vi "Main HMI.vi"() -> ()   [LabVIEW 2023]
uses:
  Classes/DCIR_HPPC_class/HPPC Parameters.ctl
  Classes/DCIR_HPPC_class/HPPC Mode.ctl
  Types/Tabs.ctl
  Types/Power Function.ctl
  Types/Setpoints.ctl
  Classes/Battery_class/Simulation Parameters.ctl
  Types/Range.ctl
  Classes/Battery_class/Battery.lvclass
  Classes/Grapher_class/Grapher.lvclass
  Classes/DCIR_HPPC_class/DCIR_HPPC.lvclass
  Classes/ACIR_EIS_class/ACIR_EIS.lvclass
  Classes/Logger_class/Logger.lvclass
  builds/PowerModuleInterface/PowerModuleInterface.lvlibp/Classes/PowerModule_interface/PowerModuleInterface.lvclass
  Classes/ACIR_EIS_class/EIS Parameters.ctl
  Classes/ACIR_EIS_class/EIS Mode.ctl
  builds/PowerModuleInterface/PowerModuleInterface.lvlibp/Classes/PowerModule_interface/Range.ctl
  builds/PowerModuleInterface/PowerModuleInterface.lvlibp/Classes/PowerModule_interface/Slew Rates.ctl
  Types/Indicators.ctl
  <vilib>/Utility/miscctls.llb/LVStringsAndValuesArrayTypeDef_I16.ctl
  <vilib>/addons/_JKI Toolkits/State Machine/_JKI_lib_State_Machine.llb/Select State(s)_err__jki_lib_state_machine.vi
  <vilib>/Utility/TDMS File Viewer/TDMS - File Viewer (NXG Style).vi
  <vilib>/Utility/file.llb/Read Delimited Spreadsheet (DBL).vi
  <userlib>/_OpenG.lib/appcontrol/appcontrol.llb/openg_application_control.lvlib
  <vilib>/Utility/TDMS File Viewer/NI_TDMS File Viewer.lvlib
panel:
  out "Charge Counter":dbl caption="CHARGE (Ah)" format="%#.2f"
  out "Current Range":T1 caption="RANGE"
  out "Voltage Range":T1 caption="RANGE"
  out "Charging":bool caption="CHARGE"
  out "Discharging":bool caption="DISCHARGE"
  in  "Module Selection":i16(ring)=-1 caption="MODULE" items=["NONE"=-1, "HPS-17000"=0, "Simulated"=1]
  out "EMO Indicator":u16(ring)
  in  "Start Logging":bool
  out "Function":T2=enum."STANDBY" caption="FUNCTION"
  out "MODE":string
  in  "PMOD Clear":bool
  out "Status Message":string
  in  "PMOD Reserve":bool
  in  "PMOD Connect":bool
  out "Fault Message":string
  in  "Acknowledge Faults":bool
  out "Power Maximum":dbl caption="MAX"
  out "Power Minimum":dbl caption="MIN"
  out "Current Maximum":dbl caption="MAX"
  out "Current Minimum":dbl caption="MIN"
  out "Voltage Maximum":dbl caption="MAX"
  out "Voltage Minimum":dbl caption="MIN"
  in  "Main Tab Control":T3=enum."CONTROL"
  out "XY Graph":T4(graph)
  in  "Use Local Time":bool=TRUE caption="LOCAL TIME"
  in  "Pause Chart":bool
  in  "Save Chart":bool
  in  "Erase Chart":bool
  out "Module Plugin Directory":path caption="MODULE PLUGIN DIRECTORY"
  in  "Profile Step dT (ns)":i64=10000 caption="PROFILE STEP TIME (ns)"
  in  "Graph Samples":u32=10000 caption="CHART SAMPLES"
  in  "Graph Data Decimation":i32=100 caption="CHART DECIMATION"
  in  "Log File Directory":path caption="LOG FILE DIRECTORY"
  in  "Power Module Plugins":i32(listbox)=-1 caption="POWER MODULE PLUGINS"
  in  "Apply Slew Rates":bool
  in  "Slew Rates":T5={"Voltage Inc. [V/sec]"=inf, "Voltage Dec. [V/sec]"=inf, "Current Inc. [A/sec]"=inf, "Current Dec. [A/sec]"=inf, "Resistance Inc. [Ohms/sec]"=inf, "Resistance Dec. [Ohms/sec]"=inf} caption="SLEW RATES"
  in  "Output":bool caption="OUTPUT"
  in  "Apply Limits":bool
  in  "Limits":T6 caption="LIMITS"
  in  "Apply Setpoints":bool
  in  "Setpoints":T7 caption="SETPOINTS"
  in  "Energize":bool caption="ENERGIZE"
  in  "Apply Mode & Range":bool
  in  "Mode & Range":cluster{"Mode":u16, "Range":u16}={"Mode"=1, "Range"=1} caption="MODE | RANGE" {"Range" items=["0,1500 V / -240,240 A"=1]; "Mode" items=["CONSTANT CURRENT & VOLTAGE"=1]}
  out "Mini Chart":dbl[][](graph)
  in  "CSV Profile Path":path caption="CSV PROFILE"
  in  "Start Profile":bool
  out "CSV Profile":waveform(dbl)[](graph)
  in  "Battery Cells in Parallel":u16=1 caption="# Cells in Parallel"
  in  "Battery Cells in Series":u16=100 caption="# Cells in Series"
  in  "Battery Simulation Parameters":T8={"# RC Pairs"=1, "R0 (Ohm)"=0.0015, "R1 (Ohm)"=0.001, "C1 (Farad)"=2500.0, "R2 (Ohm)"=0.0008, "C2 (Farad)"=40000.0, "Nominal Capacity (Ah)"=10.0, "Upper Cutoff Voltage"=5.0, "Lower Cutoff Voltage"=2.5, "Coulombic Efficiency"=1.0} {"# RC Pairs" min=1 max=2}
  in  "Reset Battery Simulation":bool
  in  "Enable Battery Simulation":bool caption="ENABLE BATTERY SIMULATION"
  in  "Launch Battery Simulation":bool
  in  "Toggle EIS Profile":bool
  in  "Generate EIS Profile":bool
  in  "EIS Parameters":T9={"EIS Mode"=2, "EIS DC Potential"=650.0, "EIS Start Frequency"=1000.0, "EIS Stop Frequency"=500.0, "EIS Delta Frequency"=100.0, "EIS DC Current"=0.0, "AC Signal (mV/mA RMS)"=20.0, "Cycles at Frequency"=5.0, "EIS AC Step Delay"=1.0} {"EIS Mode" items=["Voltage (PEIS)"=1, "Current (GEIS)"=2]}
  in  "Toggle HPPC Profile":bool
  in  "Generate HPPC Profile":bool
  in  "HPPC Parameters":T10={"HPPC Mode"=1, "Pulse Duration (S)"=10.0, "Charge Current (A)"=25.0, "Rest Duration (S)"=10.0, "Discharge Current (A)"=25.0, "Nominal Capacity (Ah)"=10.0, "Initial SoC (%)"=90.0, "Final SoC (%)"=10.0, "SoC Interval (%)"=10.0, "SoC Step Current (A)"=100.0, "SoC Step Relax (S)"=10.0, "Minimum Voltage (V)"=300.0, "Maximum Voltage (V)"=500.0} {"HPPC Mode" items=["Discharge Only", "Full Cycle"]; "Nominal Capacity (Ah)" min=0.0 max=100.0; "Final SoC (%)" min=0.0 max=100.0; "SoC Interval (%)" min=0.0 max=100.0; "Initial SoC (%)" min=0.0 max=100.0}
  in  "Get Events":bool
  in  "Events":i32(listbox)=-1 caption="POWER MODULE PLUGINS"
  in  "TDMS Viewer":bool
  out "Fault":bool caption="FAULT"
  out "Output Enabled":bool caption="OUTPUT ENABLED"
  out "Output Disabled":bool caption="OUTPUT DISABLED"
  out "System Power":bool caption="SYSTEM POWER"
  out "POWER":dbl(knob) caption="Gauge" scale=150.0..-150.0
  out "CURRENT":T12(knob)={"Numeric Indicator"=0.0, "Numeric Indicator"=-480.0} caption="Gauge" scale=240.0..-240.0
  out "VOLTAGE":T12(knob) caption="Gauge"
  # "-"
  # "-"
  # "OFF               ON"
  # "OFF               ON"
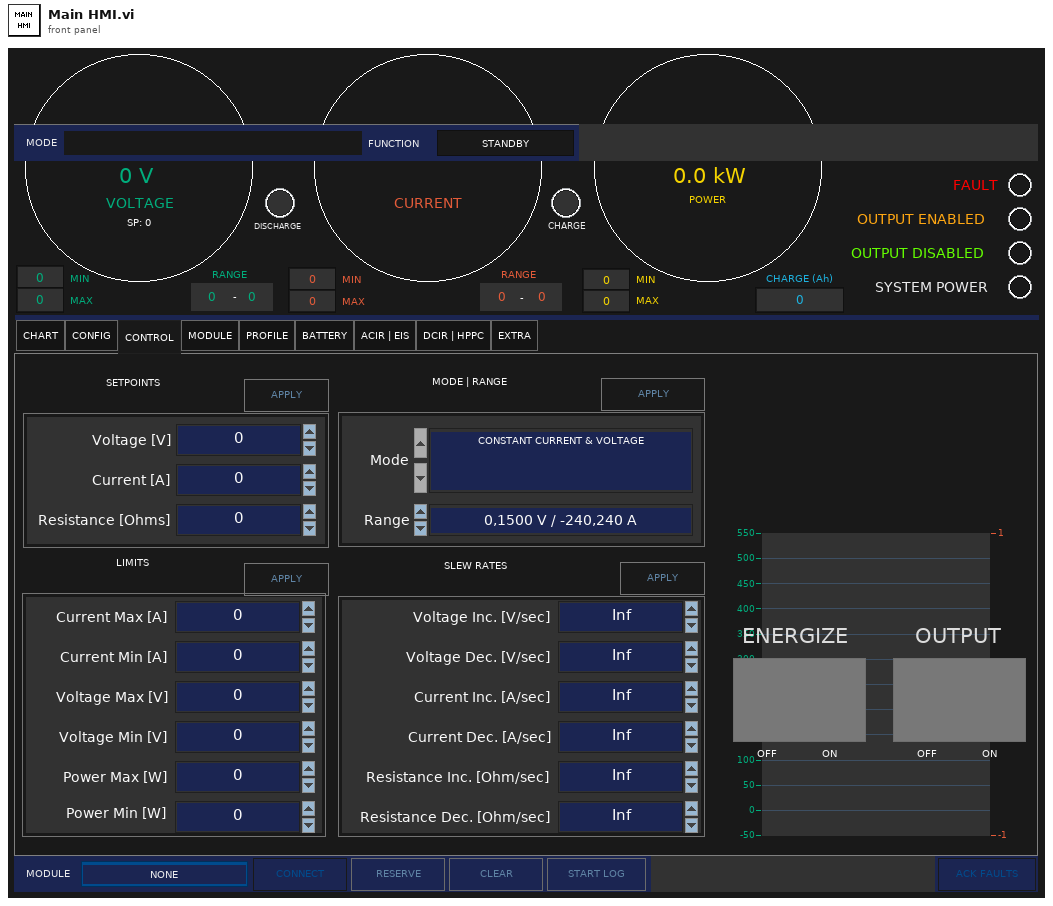
[diagram p1: front panel]
types:
  T1 = typedef "Range.ctl" = cluster{"min":dbl, "max":dbl}
  T2 = typedef "Power Function.ctl" = enum16{"REGEN (LOAD)", "STANDBY", "SUPPLY (SOURCE)"}
  T3 = typedef "Tabs.ctl" = enum32{"CHART", "CONFIG", "CONTROL", "MODULE", "PROFILE", "BATTERY", "ACIR | EIS", "DCIR | HPPC", "EXTRA"}
  T4 = cluster{"timestamp":dbl[], "setpoint current":dbl[]}[]
  T5 = cluster{"Voltage Inc. [V/sec]":sgl, "Voltage Dec. [V/sec]":sgl, "Current Inc. [A/sec]":sgl, "Current Dec. [A/sec]":sgl, "Resistance Inc. [Ohms/sec]":sgl, "Resistance Dec. [Ohms/sec]":sgl}
  T6 = cluster{"Current Max Limit":sgl, "Current Min Limit":sgl, "Voltage Max Limit":sgl, "Voltage Min Limit":sgl, "Power Max Limit":sgl, "Power Min Limit":sgl}
  T7 = typedef "Setpoints.ctl" = cluster{"Voltage":dbl, "Current":dbl, "Resistance [Ohms]":dbl}
  T8 = typedef "Battery.lvclass/Simulation Parameters.ctl" = cluster{"# RC Pairs":u8, "R0 (Ohm)":dbl, "R1 (Ohm)":dbl, "C1 (Farad)":dbl, "R2 (Ohm)":dbl, "C2 (Farad)":dbl, "Nominal Capacity (Ah)":dbl, "Upper Cutoff Voltage":dbl, "Lower Cutoff Voltage":dbl, "Coulombic Efficiency":dbl}
  T9 = cluster{"EIS Mode":u16, "EIS DC Potential":dbl, "EIS Start Frequency":dbl, "EIS Stop Frequency":dbl, "EIS Delta Frequency":dbl, "EIS DC Current":dbl, "AC Signal (mV/mA RMS)":dbl, "Cycles at Frequency":dbl, "EIS AC Step Delay":dbl}
  T10 = typedef "DCIR_HPPC.lvclass/HPPC Parameters.ctl" = cluster{"HPPC Mode":T11, "Pulse Duration (S)":dbl, "Charge Current (A)":dbl, "Rest Duration (S)":dbl, "Discharge Current (A)":dbl, "Nominal Capacity (Ah)":dbl, "Initial SoC (%)":dbl, "Final SoC (%)":dbl, "SoC Interval (%)":dbl, "SoC Step Current (A)":dbl, "SoC Step Relax (S)":dbl, "Minimum Voltage (V)":dbl, "Maximum Voltage (V)":dbl}
  T11 = typedef "DCIR_HPPC.lvclass/HPPC Mode.ctl" = u16
  T12 = cluster{"Numeric Indicator":dbl, "Numeric Indicator":dbl}
  T13 = cluster{"Core":cluster{"Current VI Reference":refnum<vi>, "Close Panel on Exit?":bool}, "Connected":bool, "Reserved":bool, "Battery Ref":refnum<class "Battery.lvclass">, "Grapher Ref":refnum<class "Grapher.lvclass">, "HPPC Ref":refnum<class "DCIR_HPPC.lvclass">, "EIS Ref":refnum<class "ACIR_EIS.lvclass">, "Logger Ref":refnum<class "Logger.lvclass">, "Power Module":refnum<class "PowerModuleInterface.lvclass">, "EIS Profile Completed":refnum<user-event>, "DCIR Profile Completed":refnum<user-event>, "Last Periodic Update":u32, "Loaded Profile":dbl[][], "Plugin Objects":refnum<class "PowerModuleInterface.lvclass">[]}
  T14 = enum8{"Enabled", "Disabled", "Disabled and Grayed Out"}
  T15 = enum32{"Invalid", "Standard", "Closed", "Hidden", "Minimized", "Maximized"}
  T16 = enum32{"invalid app kind", "Development System", "Run Time System", "Student Edition", "Embedded LabVIEW", "Evaluation", "Custom"}
  T17 = typedef "ACIR_EIS.lvclass/EIS Parameters.ctl" = cluster{"EIS Mode":T18, "EIS DC Potential":dbl, "EIS Start Frequency":dbl, "EIS Stop Frequency":dbl, "EIS Delta Frequency":dbl, "EIS DC Current":dbl, "AC Signal (mV/mA RMS)":dbl, "Cycles at Frequency":dbl, "EIS AC Step Delay":dbl}
  T18 = typedef "ACIR_EIS.lvclass/EIS Mode.ctl" = u16
  T19 = typedef "PowerModuleInterface.lvlibp/PowerModuleInterface.lvclass/Range.ctl" = cluster{"Current Max (A)":dbl, "Current Min (A)":dbl, "Voltage Max (V)":dbl, "Voltage Min (V)":dbl}
  T20 = typedef "PowerModuleInterface.lvlibp/PowerModuleInterface.lvclass/Slew Rates.ctl" = cluster{"Current Decrease (A/sec)":dbl, "Current Increase (A/sec)":dbl, "Voltage Decrease (V/sec)":dbl, "Voltage Increase (V/sec)":dbl, "Resistance Decrease (Ohm/sec)":dbl, "Resistance Increase (Ohm/sec)":dbl}
  T21 = typedef "Indicators.ctl" = cluster{"XY Graph":refnum<vi>, "Mini Chart":refnum<vi>, "Voltage":refnum<vi>, "Current":refnum<vi>, "Power":refnum<vi>, "Function":refnum<vi>, "Charging":refnum<vi>, "Discharging":refnum<vi>, "Charge Counter":refnum<vi>}
  T22 = typedef "LVStringsAndValuesArrayTypeDef_I16.ctl" = cluster{"String":string, "Value":i16}[]
  T23 = cluster{"Current VI Reference":refnum<vi>, "Close Panel on Exit?":bool}
  T24 = typedef "PowerModuleInterface.lvlibp/PowerModuleInterface.lvclass/Limits.ctl" = cluster{"Current Max (A)":dbl, "Current Min (A)":dbl, "Voltage Max (V)":dbl, "Voltage Min (V)":dbl, "Power Max (W)":dbl, "Power Min (W)":dbl}
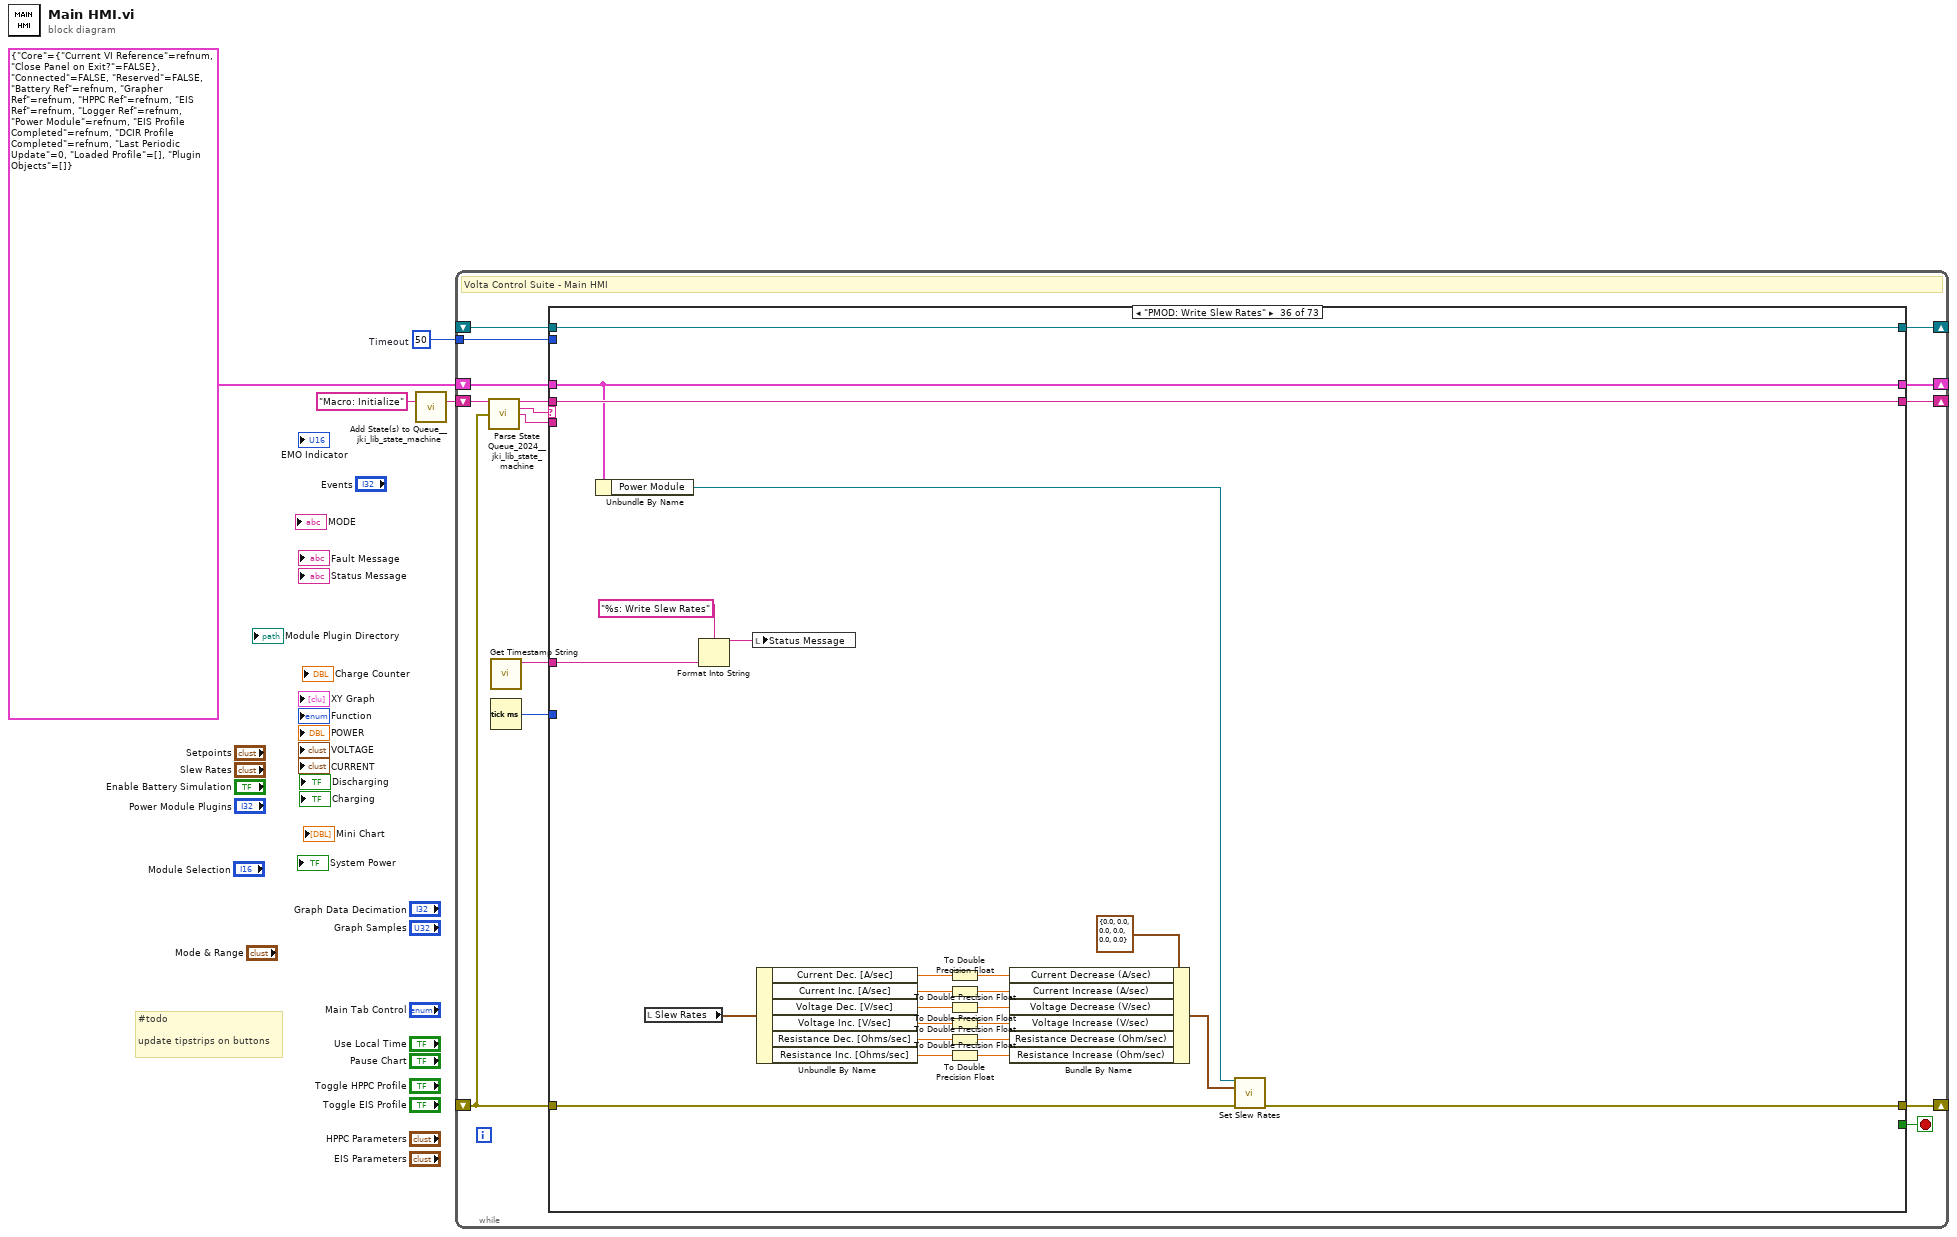
[diagram p0: block diagram]
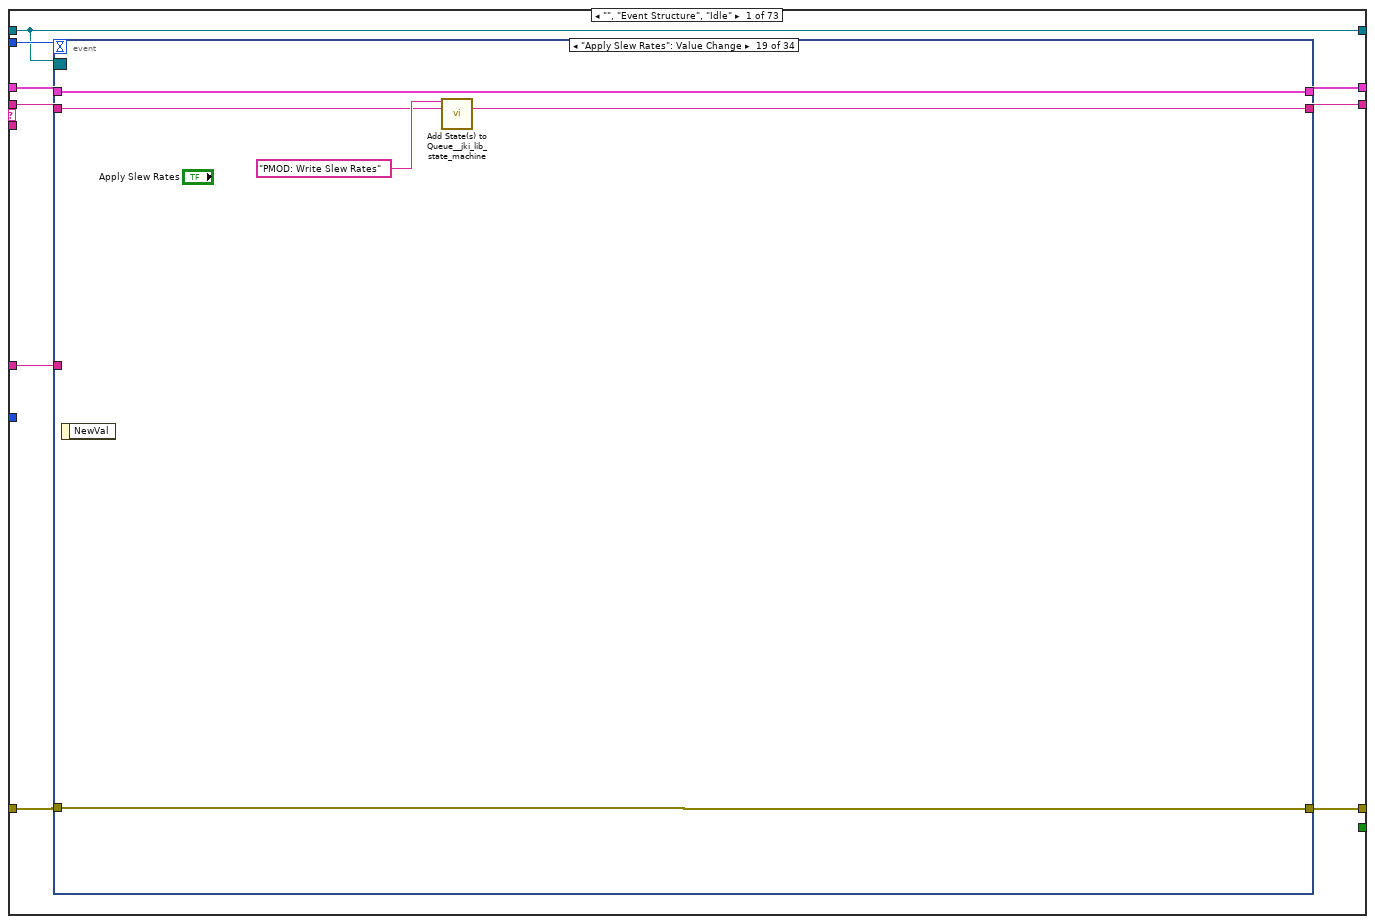
[diagram p2: hidden frame]
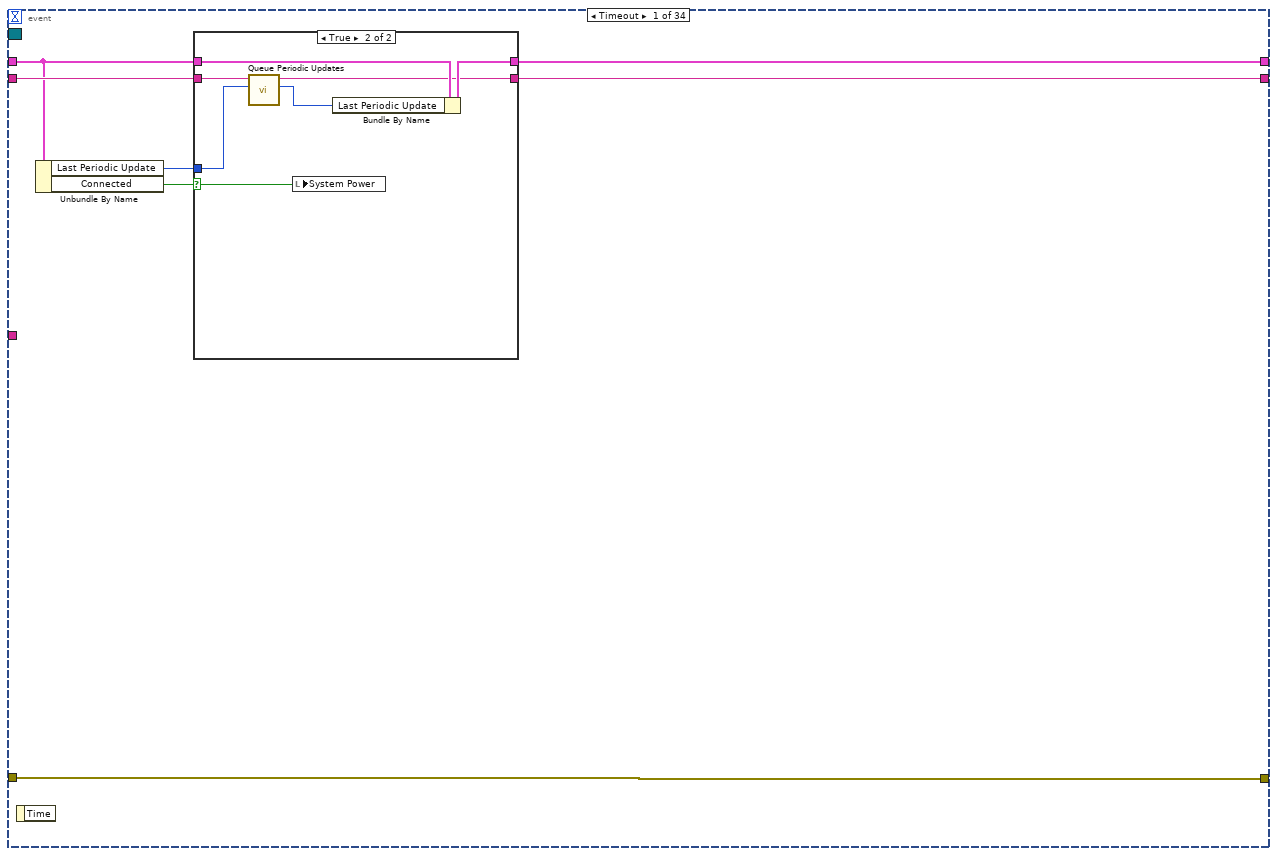
[diagram p3: hidden frame]
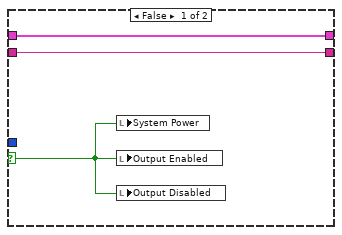
[diagram p4: hidden frame]
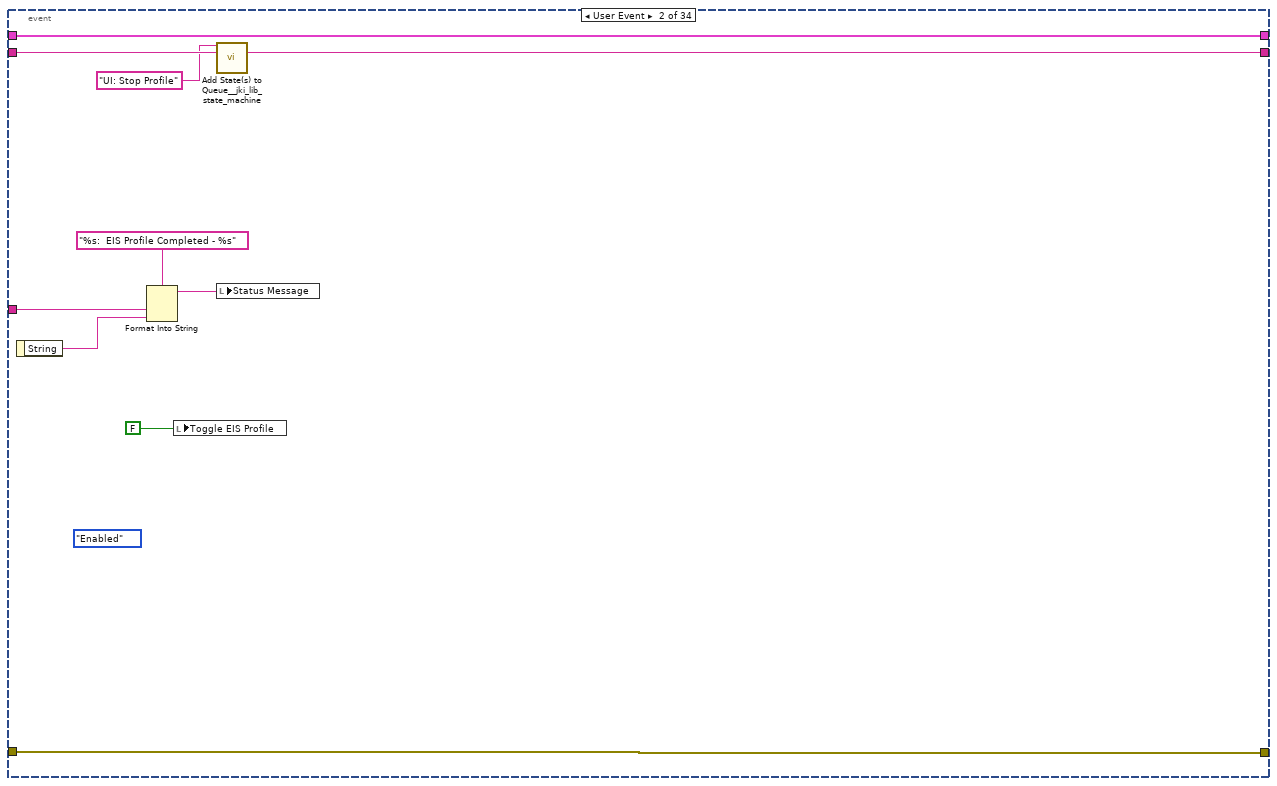
[diagram p5: hidden frame]
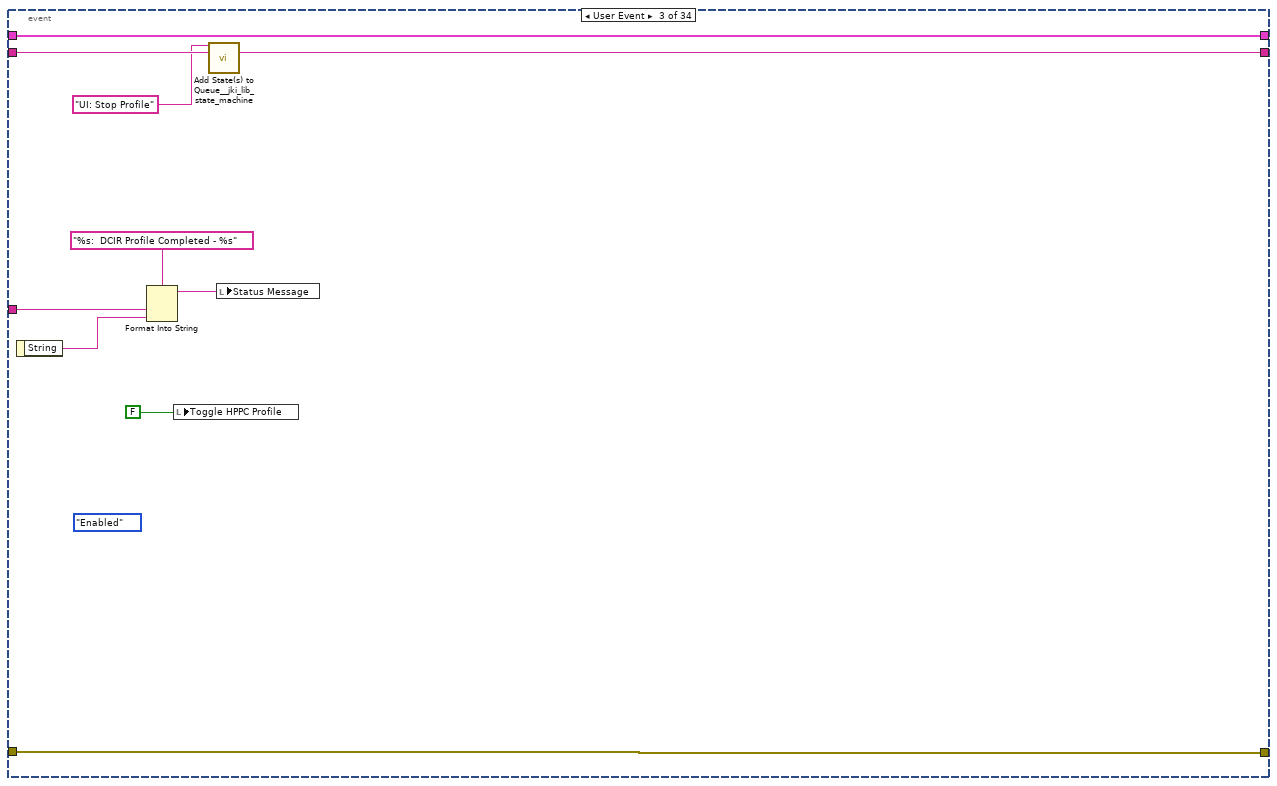
[diagram p6: hidden frame]
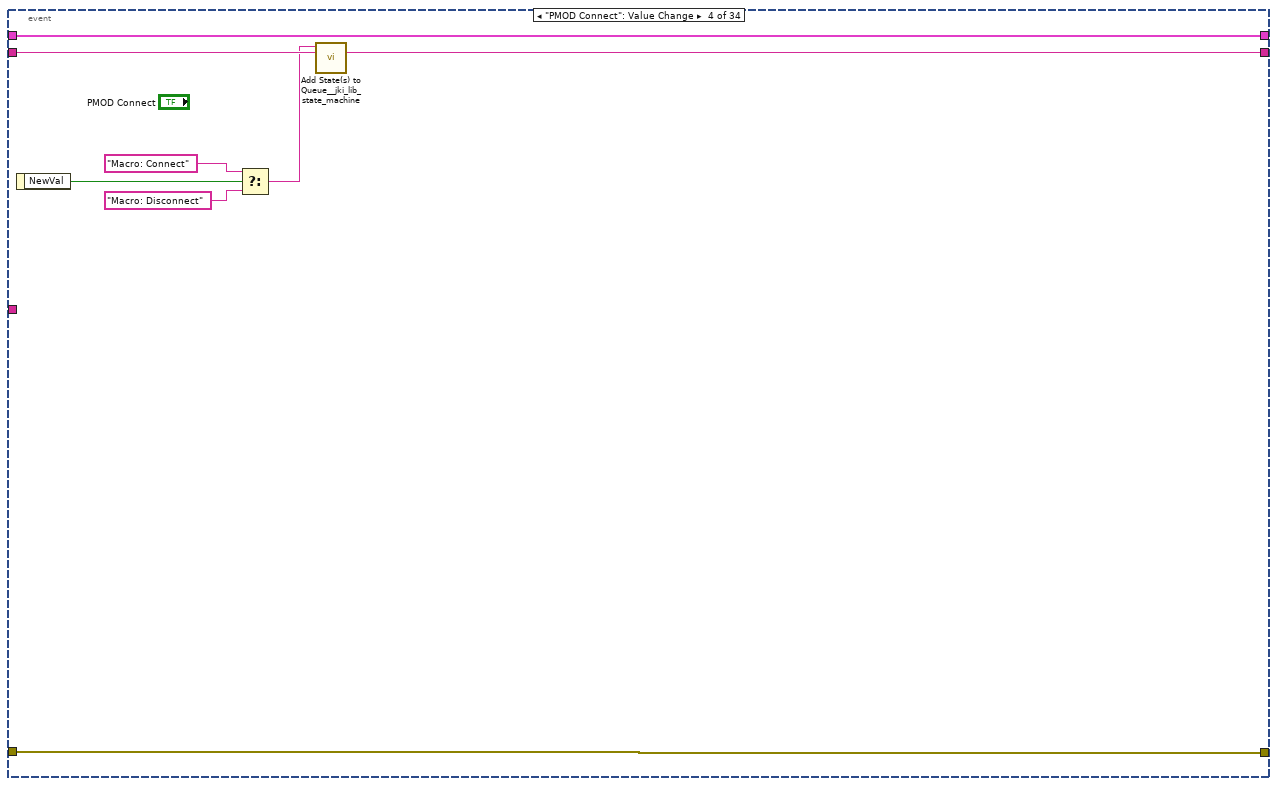
[diagram p7: hidden frame]
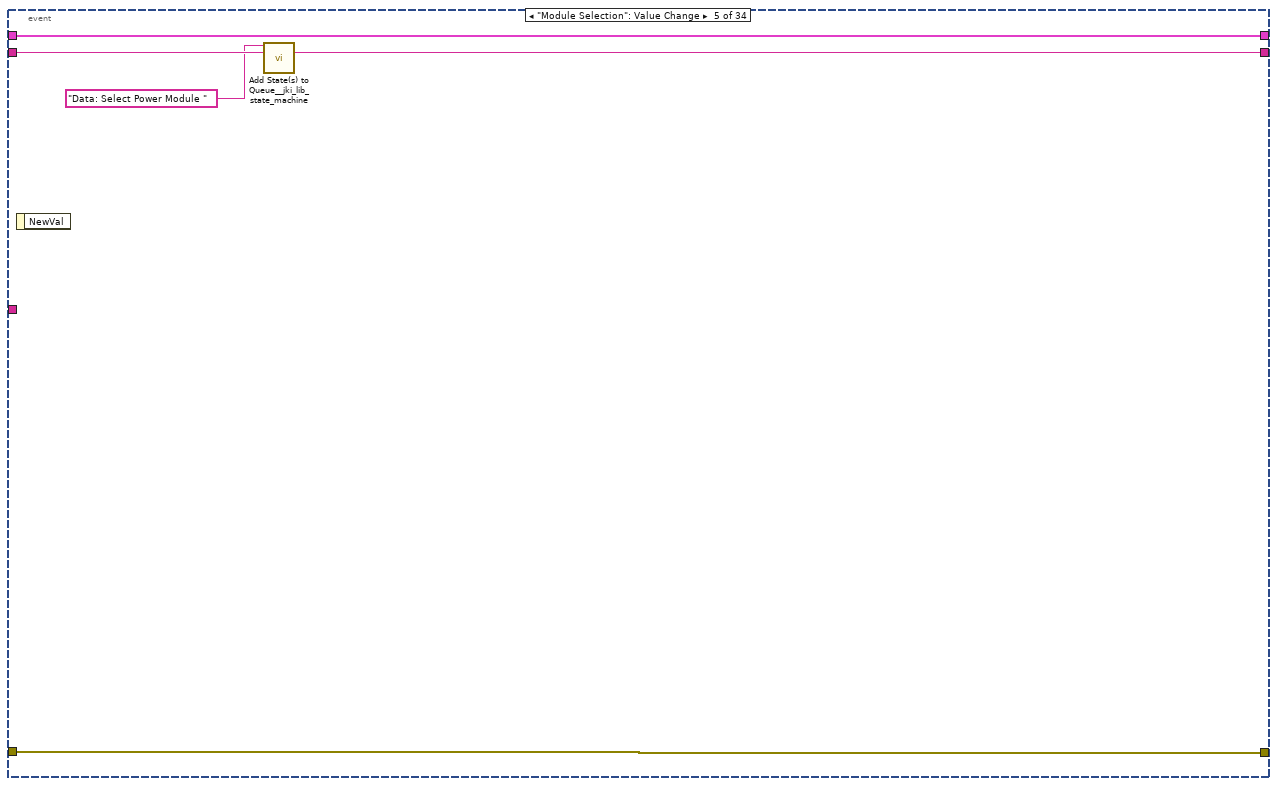
[diagram p8: hidden frame]
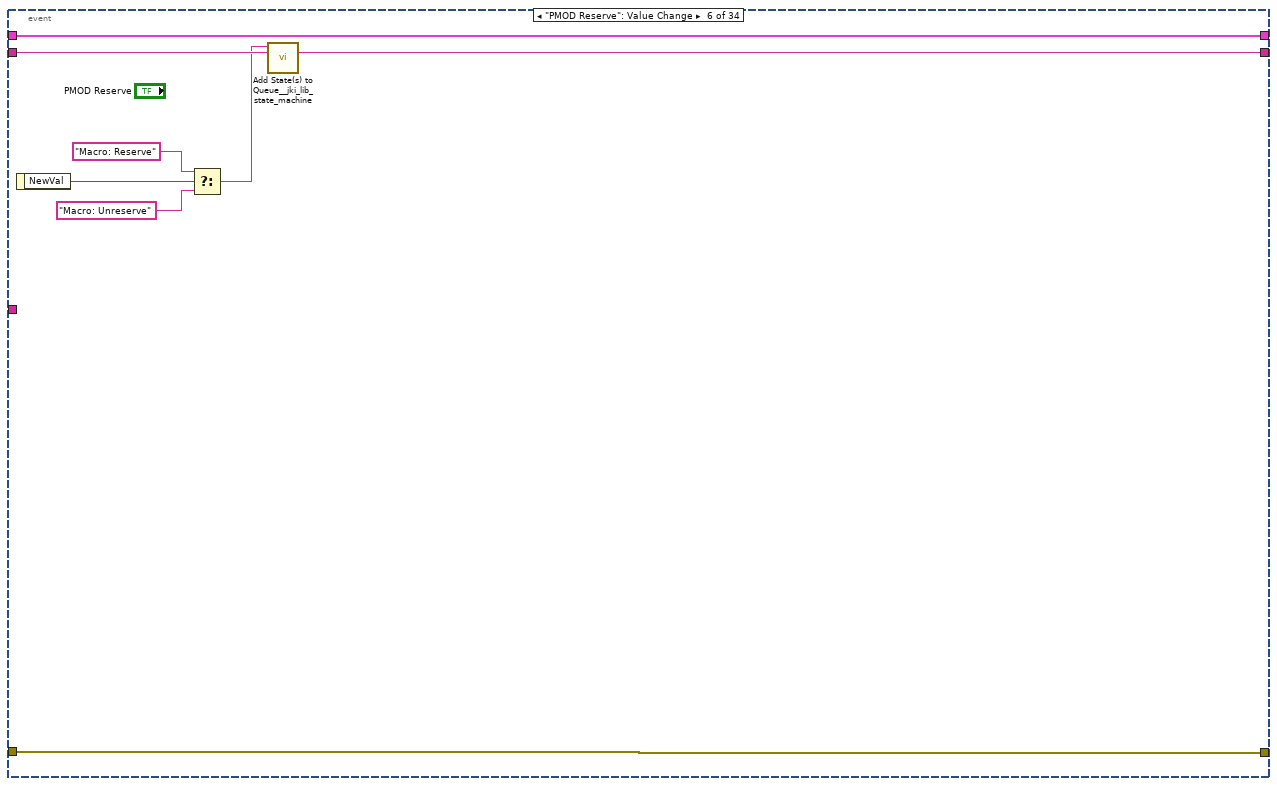
[diagram p9: hidden frame]
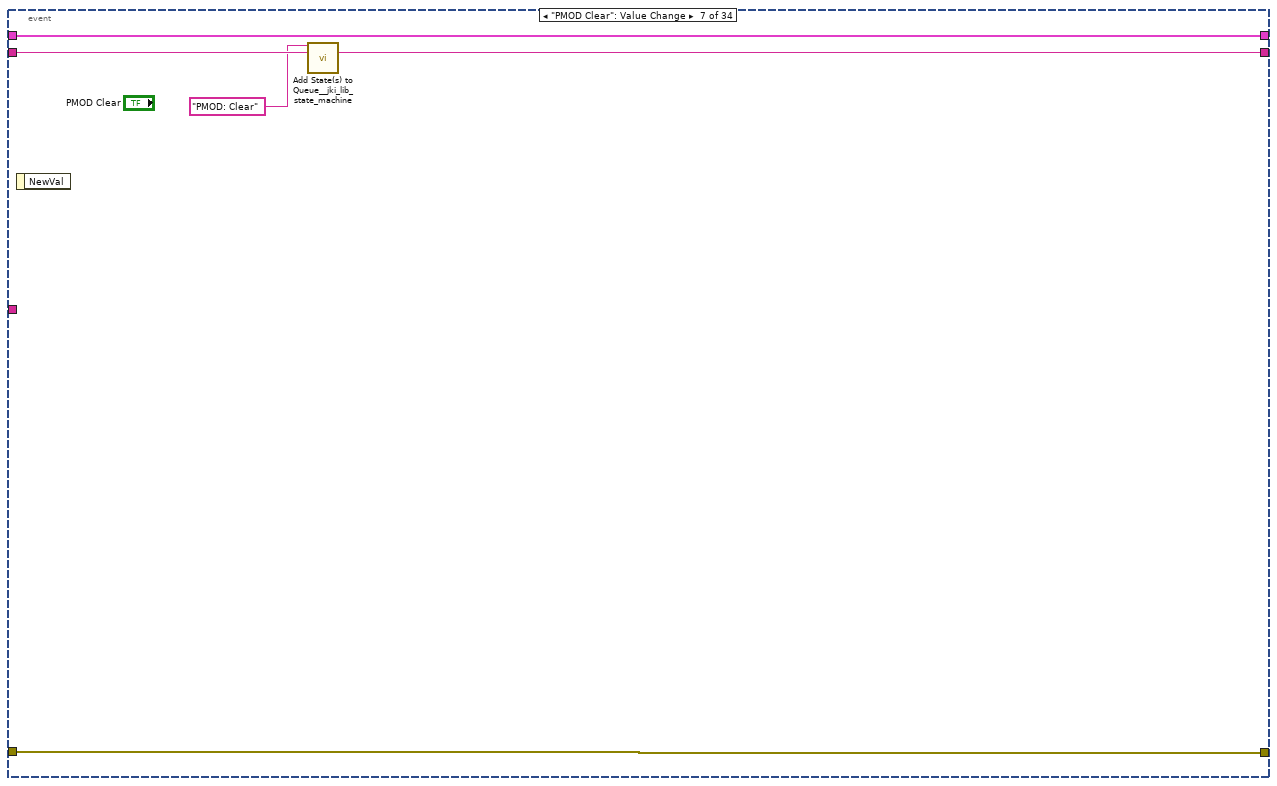
[diagram p10: hidden frame]
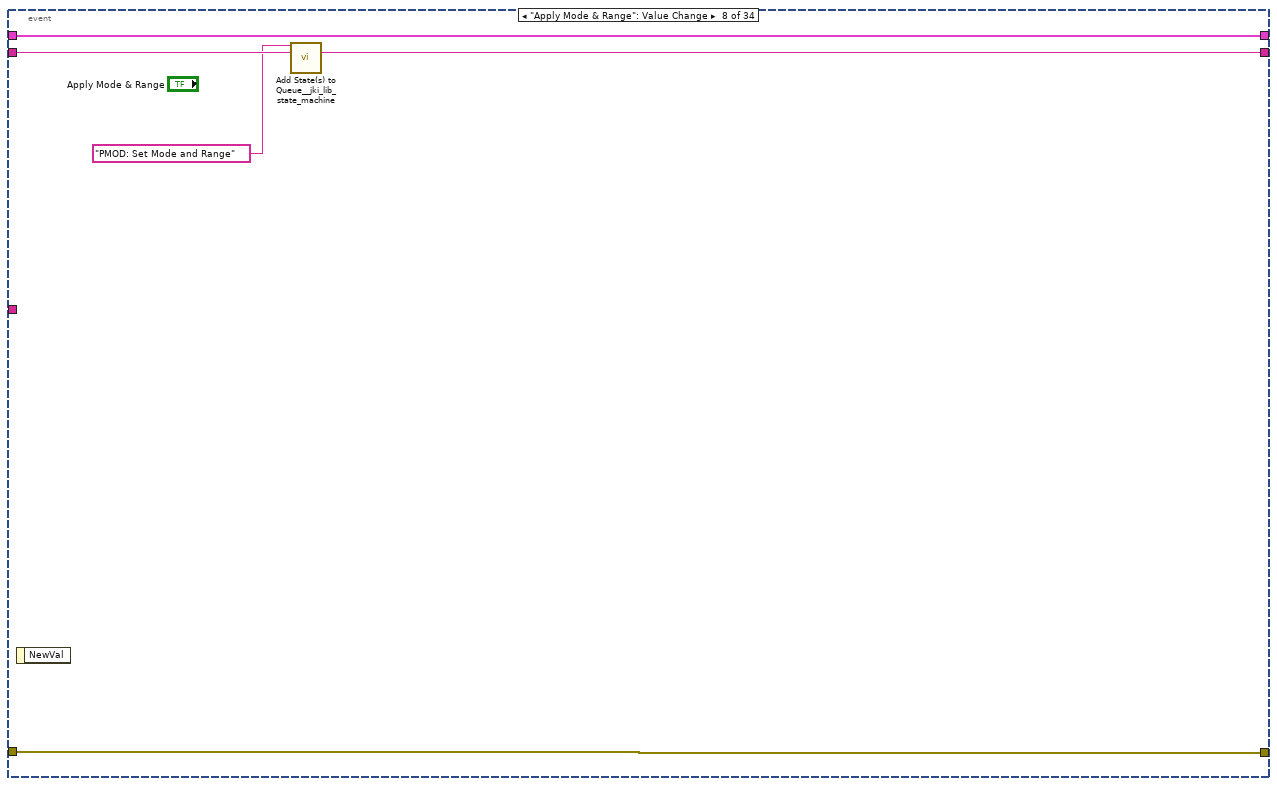
[diagram p11: hidden frame]
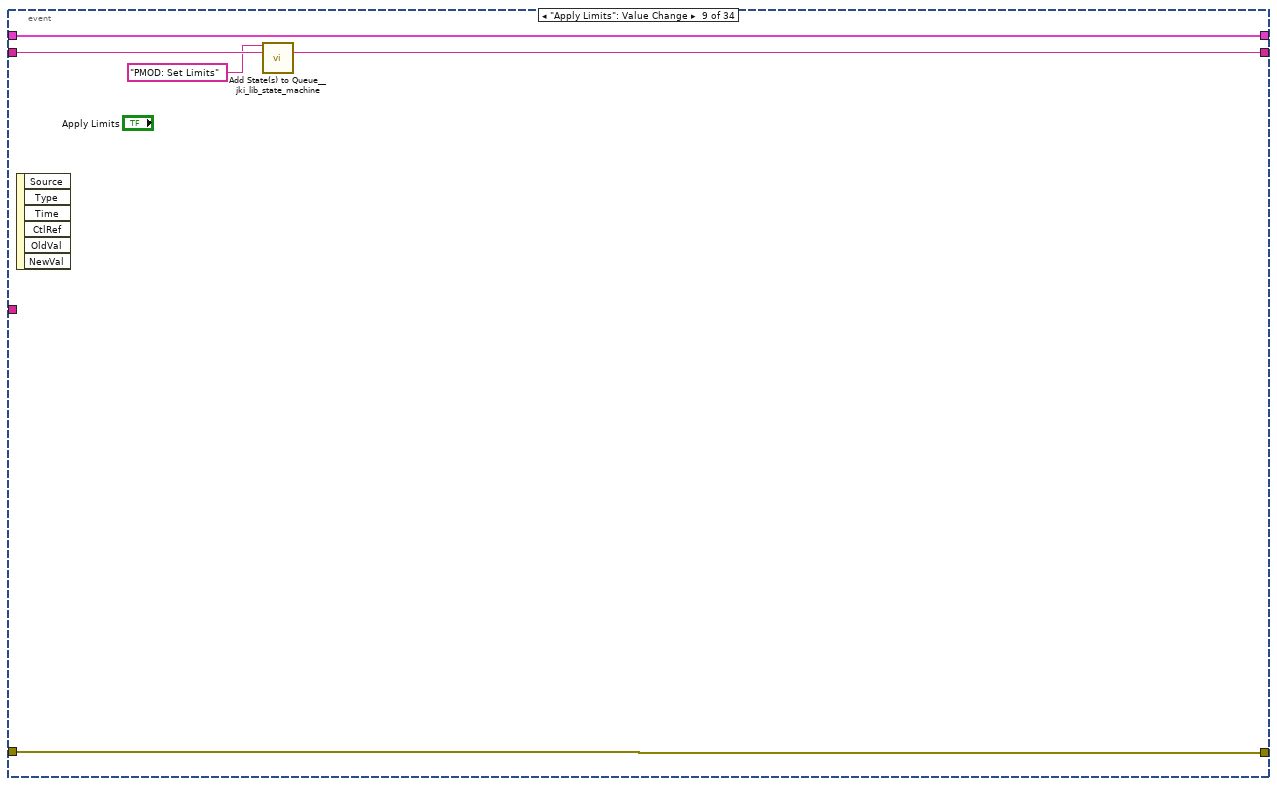
[diagram p12: hidden frame]
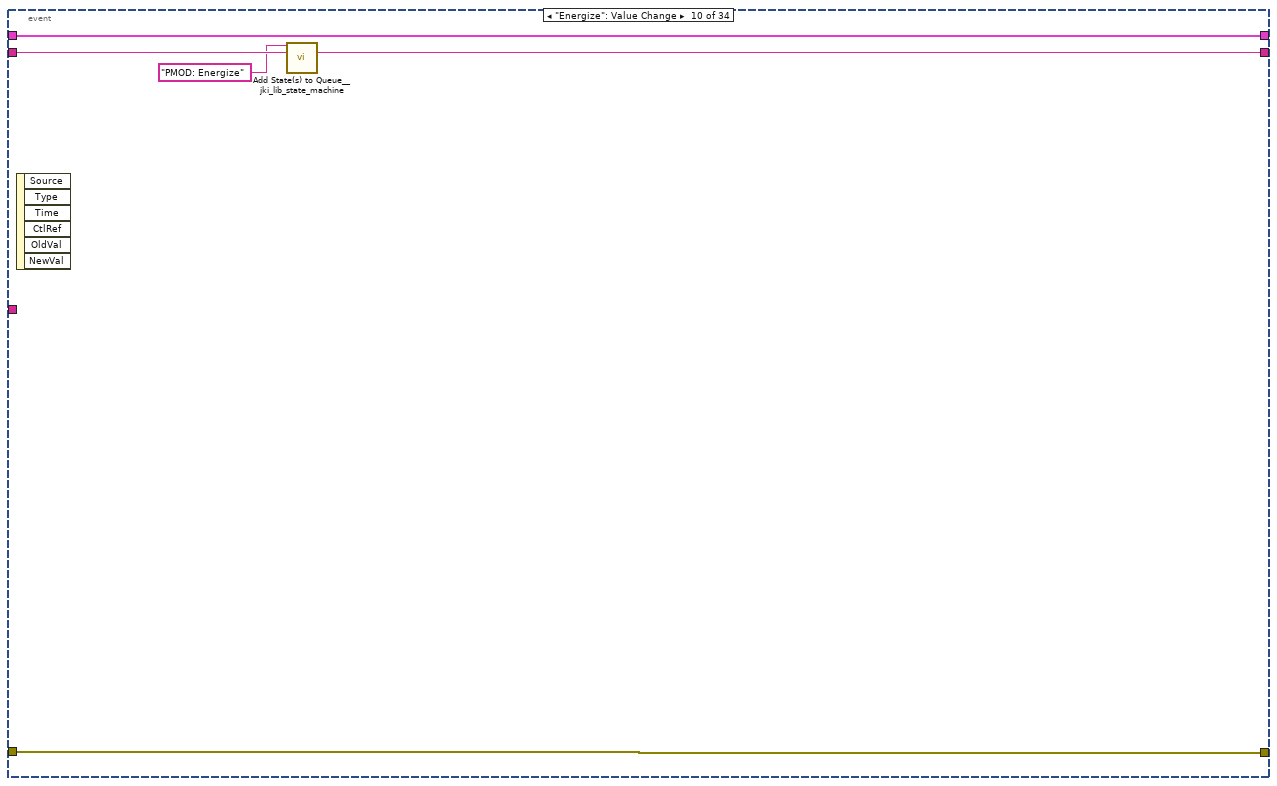
[diagram p13: hidden frame]
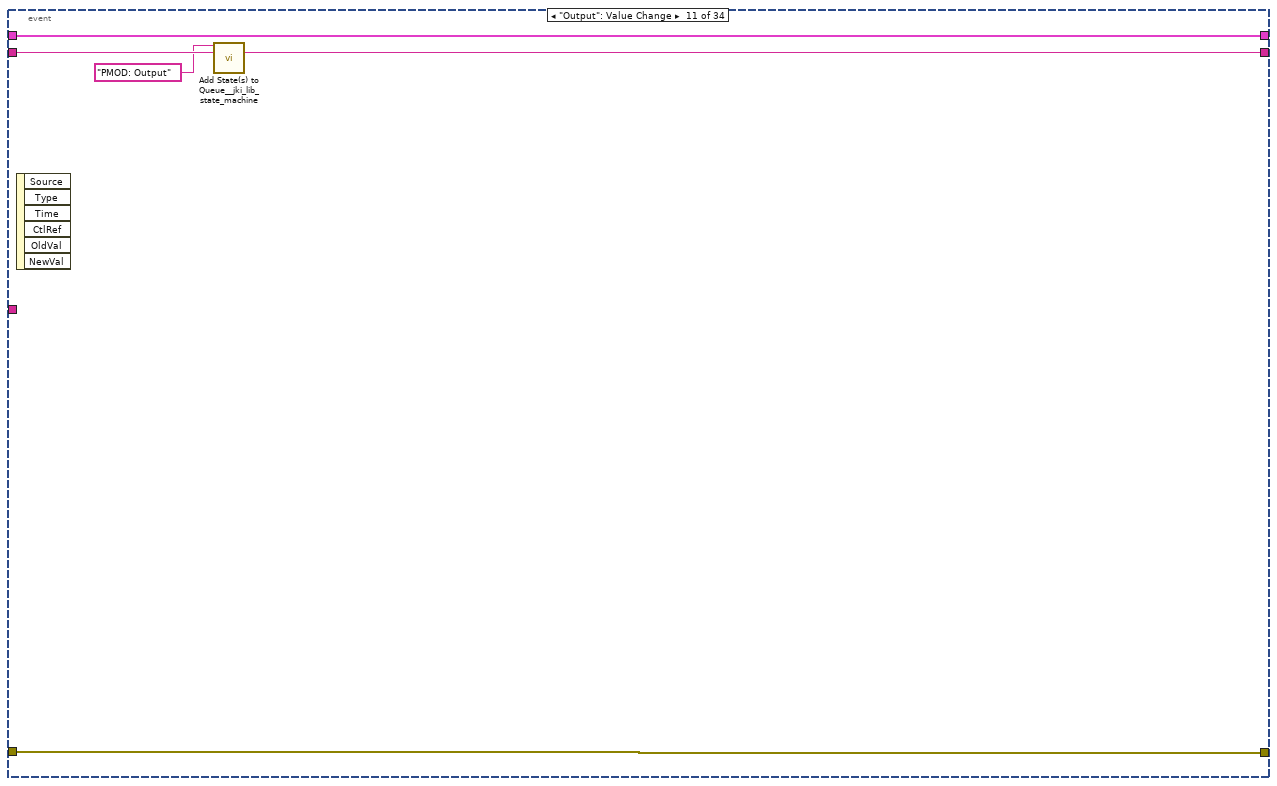
[diagram p14: hidden frame]
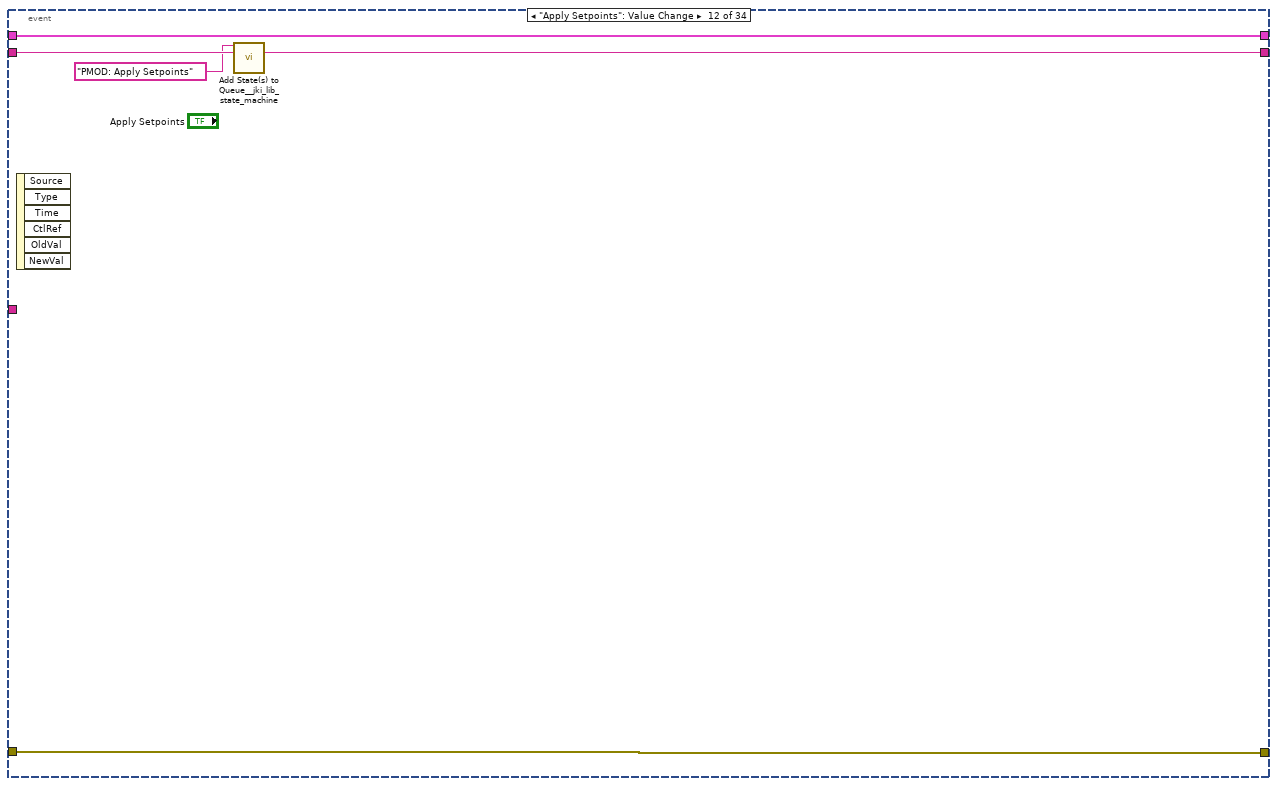
[diagram p15: hidden frame]
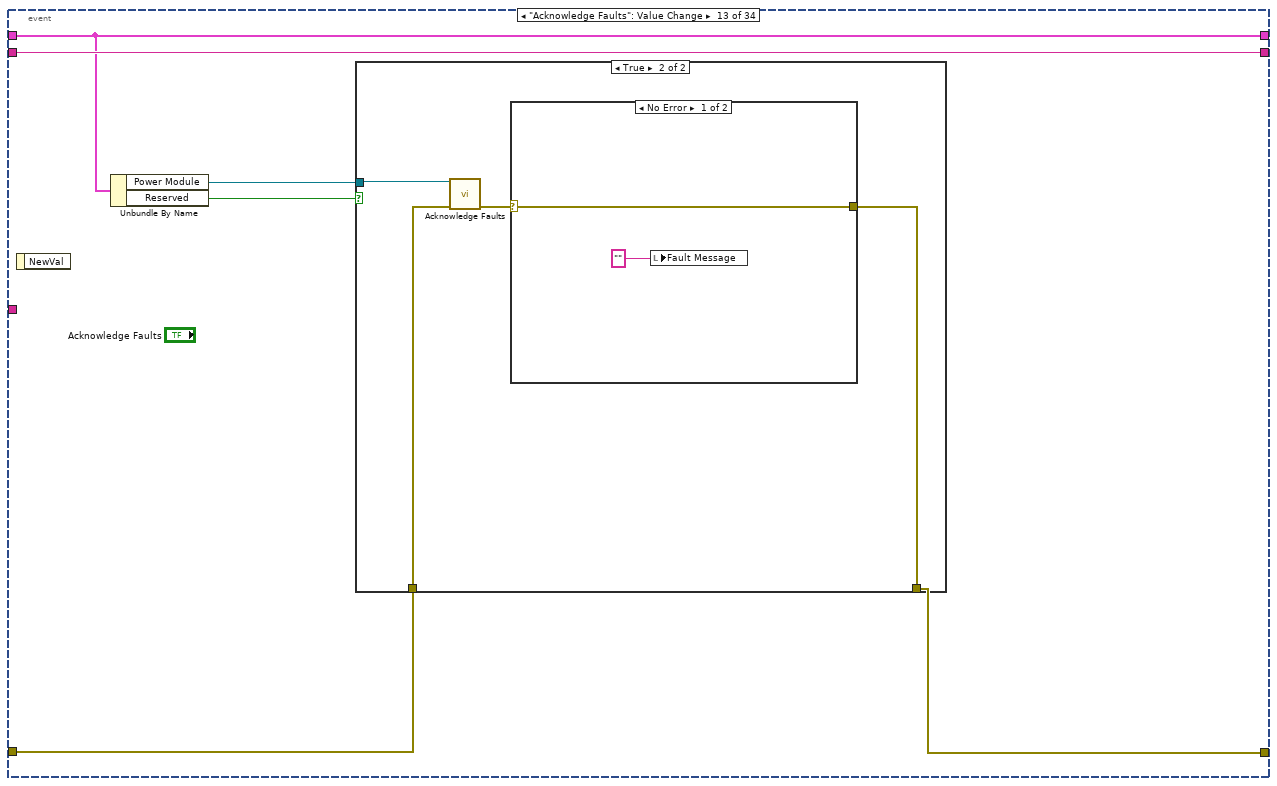
[diagram p16: hidden frame]
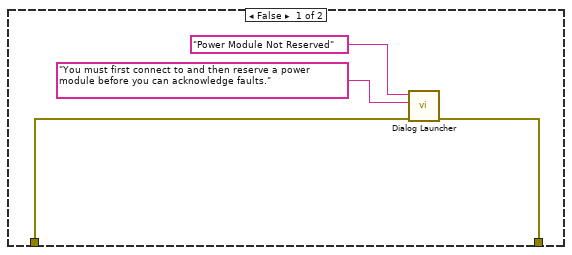
[diagram p17: hidden frame]
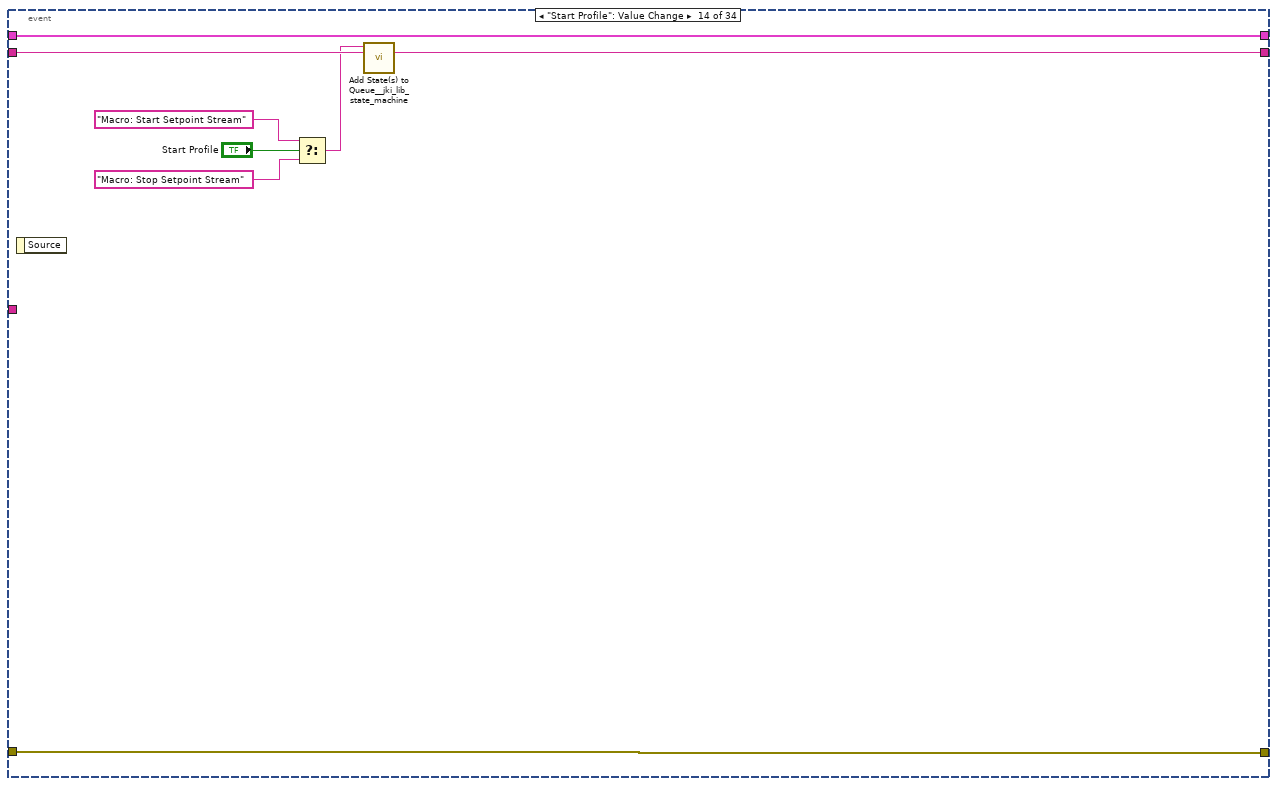
[diagram p19: hidden frame]
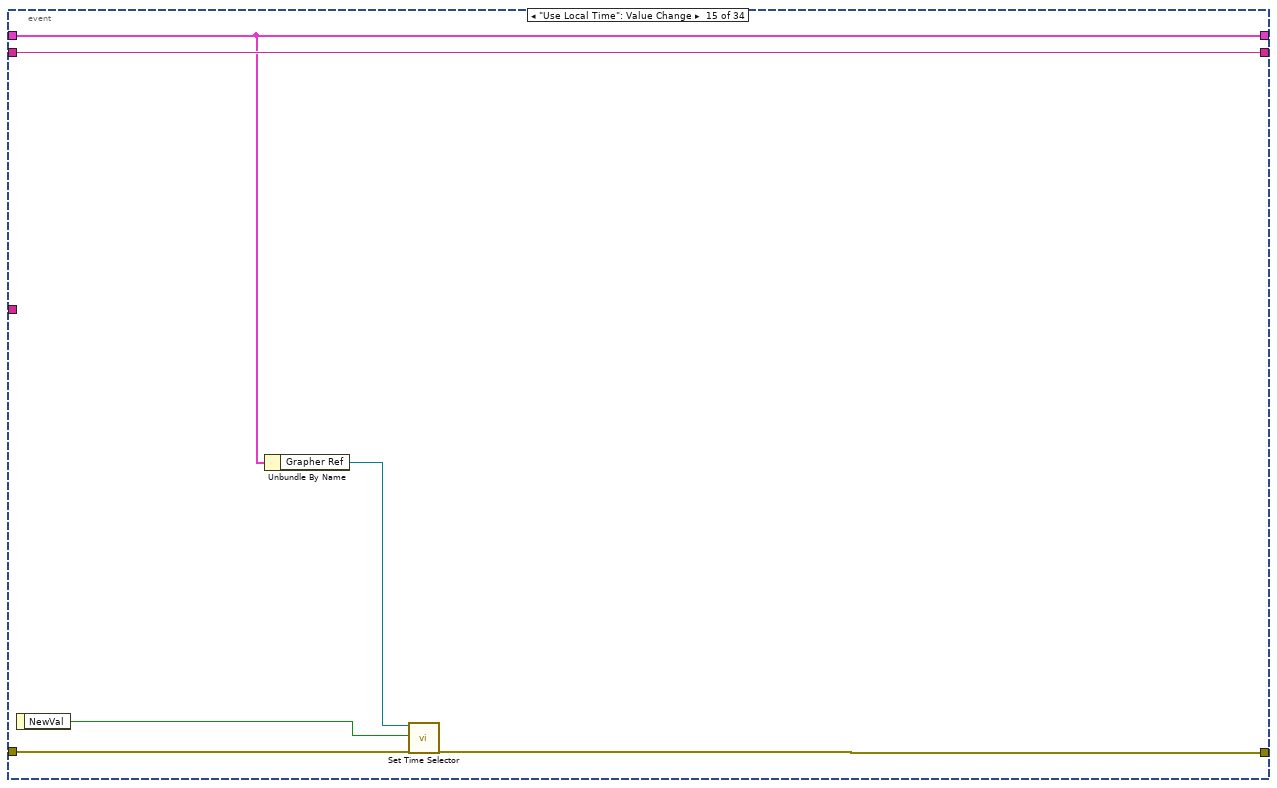
[diagram p20: hidden frame]
diagram:
  w2 = 50  # Timeout
  # "#todo\n\nupdate tipstrips on buttons"
  n1 = call <vilib>:"Add State(s) to Queue__jki_lib_state_machine.vi"("State(s) in (\"\")"="Macro: Initialize") -> ("States Out"=w4:string)  [unwired: 14 in]
  n2 = while "JKI State Machine 2024" {
    shift-right: [w13] -> _
    shift-left: T13 {"Core"={"Current VI Reference"=refnum, "Close Panel on Exit?"=FALSE}, "Connected"=FALSE, "Reserved"=FALSE, "Battery Ref"=refnum, "Grapher Ref"=refnum, "HPPC Ref"=refnum, "EIS Ref"=refnum, "Logger Ref"=refnum, "Power Module"=refnum, "EIS Profile Completed"=refnum, "DCIR Profile Completed"=refnum, "Last Periodic Update"=0, "Loaded Profile"=[], "Plugin Objects"=[]} -> [w12]
    shift-right: [w15] -> _
    shift-left: _ -> [w11]
    shift-right: [w7] -> _
    shift-left: w4 -> [w16]
    tunnel: w2 -> [w10]
    shift-right: [w9] -> _
    shift-left: _ -> [w8]
    stop <- w14 stop-if-true
    # "Volta Control Suite - Main HMI"
    n3 = call <vilib>:"Parse State Queue_2024__jki_lib_state_machine.vi"("State Queue"=w16, "Error In (no error)"=w11) -> ("Remaining States"=w18:string, "Current State"=w19:string, "Arguments"=w17:string)  [unwired: 11 in]
    n4 = call "Get Timestamp String.vi"() -> ("date/time string"=w6:string)  [unwired: 11 in]
    n5 = Tick Count (ms)() -> (millisecond timer value=w5:u32)
    n6 = case shown="\"PMOD: Write Slew Rates\"" w19 {
      selector: w19 -> [_ _ w372 _ _ _ _ _ _ _ _ _ _ _ _ _ _ _ _ _ _ _ _ _ _ _ _ _ _ _ _ _ _ _ _ _ _ _ _ _ _ _ _ _ _ _ _ _ _ _ _ _ _ _ _ _ _ _ _ _ _ _ _ _ _ _ _ _ _ _ _ _ _]
      tunnel: w18 -> [w28 w370 w376 w396 w407 w417 w422 w453 w466 w481 w546 w589 w594 w623 w629 w639 w644 w683 w689 w699 w714 w738 w752 w789 w797 w808 w834 w875 w919 w935 w950 w966 w980 w1007 w1027 w1058 w1082 w1087 w1097 w1145 w1149 w1159 w1180 w1204 w1223 w1249 w1293 w1311 w1341 w1352 w1359 w1364 w1368 w1391 w1415 w1456 w1461 w1462 w1473 w1481 w1488 w1495 w1502 w1509 w1516 w1531 w1600 w1606 w1613 w1619 w1625 w1637 _]
      tunnel: w17 -> [_ _ _ _ w402 _ _ _ _ _ _ _ _ _ _ _ _ _ _ _ _ _ _ _ _ _ _ _ _ _ _ _ _ _ _ _ _ _ _ _ _ _ _ _ _ _ _ _ _ _ _ _ _ _ _ _ _ _ _ _ _ _ _ _ w1512 w1526 _ _ _ _ _ _ _]
      tunnel: w12 -> [w26 w367 w374 w390 w404 w412 w419 w452 w471 w479 w540 w586 w592 w622 w627 w636 w642 w682 w687 w696 w710 w736 w758 w787 w795 w806 w831 w872 w916 w930 w948 w964 w981 w1005 w1019 w1052 w1078 w1085 w1088 w1143 w1147 w1155 w1176 w1200 w1219 w1246 w1286 w1308 w1337 w1350 w1356 w1363 w1366 w1390 w1403 w1455 w1460 w1466 w1472 w1480 w1487 w1494 w1501 w1508 w1515 w1528 w1598 w1603 w1610 w1616 w1621 w1633 w1646]
      tunnel: [w25 w368 w378 w383 errorcluster {"status"=FALSE, "code"=0, "source"=""} ("error out") w413 w420 w423 w467 w476 w530 w587 w590 w624 w625 w637 w640 w684 w685 w697 w704 w726 w755 w778 w791 w804 w828 w869 w913 w928 w945 w961 w985 w1002 w1023 w1053 w1075 w1086 w1091 w1141 w1148 w1156 w1177 w1201 w1220 w1247 w1291 w1309 w1339 w1351 w1357 w1360 w1367 w1387 w1404 w1454 w1459 w1465 w1474 w1482 w1489 w1496 w1503 w1510 w1513 w1529 w1599 w1604 w1611 w1617 w1623 w1635 w1643] -> w15
      tunnel: w11 -> [w22 w368 w377 w383 w403 w413 w420 w424 w467 w477 w544 w587 w591 w624 w626 w637 w641 w684 w686 w697 w708 w729 w760 w780 w792 w801 w829 w870 w914 w931 w946 w962 w986 w1003 w1024 w1054 w1076 w1086 w1095 w1141 w1148 w1157 w1178 w1202 w1221 w1244 w1292 w1310 w1340 w1351 w1355 w1361 w1367 w1388 w1413 w1454 w1459 w1465 w1474 w1482 w1489 w1496 w1503 w1510 w1514 w1530 w1599 w1604 w1611 w1617 w1623 w1635 w1643]
      tunnel: [w27 w369 w375 w395 w406 w416 w421 w453 w466 w481 w546 w588 w594 w623 w629 w638 w644 w683 w689 w698 w713 w738 w750 w789 w797 w808 w833 w874 w918 w935 w950 w966 w980 w1007 w1027 w1058 w1082 w1087 w1097 w1145 w1149 w1159 w1180 w1204 w1223 w1249 w1293 w1311 w1341 w1352 w1359 w1364 w1368 w1391 w1415 w1456 w1461 w1462 w1473 w1481 w1488 w1495 w1502 w1509 w1516 w1531 w1600 w1605 w1612 w1618 w1624 w1636 w1639] -> w7
      tunnel: [_ _ _ _ _ TRUE _ _ _ _ _ _ _ _ _ _ _ _ _ _ _ _ _ _ _ _ _ _ _ _ _ _ _ _ _ _ _ _ _ _ _ _ _ _ _ _ _ _ _ _ _ _ _ _ _ _ _ _ _ _ _ _ _ _ _ _ _ _ _ _ _ _ _] -> w14
      tunnel: [w24 w367 w374 w394 w404 w412 w419 w452 w469 w479 w539 w586 w593 w622 w627 w636 w643 w682 w687 w696 w721 w737 w757 w786 w794 w805 w830 w871 w915 w930 w947 w963 w987 w1004 w1025 w1052 w1078 w1085 w1089 w1142 w1147 w1154 w1175 w1199 w1218 w1245 w1286 w1307 w1338 w1350 w1356 w1363 w1366 w1390 w1402 w1455 w1460 w1466 w1472 w1480 w1487 w1494 w1501 w1508 w1515 w1528 w1598 w1603 w1610 w1616 w1621 w1633 w1646] -> w13
      tunnel: w10 -> [w23 _ _ _ _ _ _ _ _ _ _ _ _ _ _ _ _ _ _ _ _ _ _ _ _ _ _ _ _ _ _ _ _ _ _ _ _ _ _ _ _ _ _ _ _ _ _ _ _ _ _ _ _ _ _ _ _ _ _ _ _ _ _ _ _ _ _ _ _ _ _ _ _]
      tunnel: [w21 w366 w371 w384 w397 w414 w418 w451 w468 w480 w545 w585 w595 w621 w628 w635 w645 w681 w688 w695 w720 w735 w761 w788 w796 w807 w832 w873 w917 w936 w949 w965 w988 w1006 w1026 w1059 w1083 w1084 w1096 w1144 w1146 w1158 w1179 w1203 w1222 w1248 w1294 w1312 w1342 w1349 w1358 w1362 w1365 w1389 w1414 w1453 w1458 w1464 w1471 w1479 w1486 w1493 w1500 w1507 w1511 w1525 w1597 w1601 w1608 w1614 w1622 w1634 w1644] -> w9
      tunnel: w8 -> [w21 w366 w371 w384 w397 w414 w418 w451 w468 w480 w545 w585 w595 w621 w628 w635 w645 w681 w688 w695 w720 w735 w761 w788 w796 w807 w832 w873 w917 w936 w949 w965 w988 w1006 w1026 w1059 w1083 w1084 w1096 w1144 w1146 w1158 w1179 w1203 w1222 w1248 w1294 w1312 w1342 w1349 _ w1362 w1365 w1389 w1414 w1453 w1458 w1464 w1471 w1479 w1486 w1493 w1500 w1507 w1511 w1525 w1597 w1601 w1608 w1614 w1622 w1634 w1644]
      tunnel: w6 -> [w20 _ _ _ _ _ _ _ _ _ _ _ _ _ _ _ _ _ _ _ _ _ _ _ _ _ _ _ _ w932 _ _ w977 _ _ w1055 w1079 _ _ _ _ _ w1171 _ _ _ w1287 _ _ _ _ _ _ w1376 w1407 _ _ _ w1467 w1475 w1483 w1490 w1497 w1504 _ _ _ _ _ _ _ _ _]
      tunnel: w5 -> [_ _ _ _ _ _ _ _ _ _ _ _ _ _ _ _ _ _ _ _ _ _ _ _ _ _ _ _ _ _ _ _ _ _ _ _ _ _ _ _ _ _ _ _ _ _ _ _ _ _ _ _ _ _ w1406 _ _ _ _ _ _ _ _ _ _ _ _ _ _ _ _ _ _]
      frame "", "Event Structure", "Idle" {
        n7 = event shown="[18] \"Apply Slew Rates\": Value Change" {
          selector: w21 -> [_ _ _ _ _ _ _ _ _ _ _ _ _ _ _ _ _ _ _ _ _ _ _ _ _ _ _ _ _ _ _ _ _ _]
          dyn-events: _ -> [_ _ _ _ _ _ _ _ _ _ _ _ _ _ _ _ _ _ _ _ _ _ _ _ _ _ _ _ _ _ _ _ _ _]
          timeout: w23 -> [_ _ _ _ _ _ _ _ _ _ _ _ _ _ _ _ _ _ _ _ _ _ _ _ _ _ _ _ _ _ _ _ _ _]
          tunnel: w28 -> [w35 w48 w59 w71 w76 w84 w89 w95 w99 w104 w109 w114 w122 w139 w147 w153 w159 w162 w166 w171 w176 w184 w192 w199 w214 w220 w235 w265 w283 w293 w305 w313 w345 w360]
          tunnel: [w34 w46 w57 w70 w75 w83 w88 w94 w98 w103 w108 w112 w122 w138 w147 w153 w159 w160 w165 w170 w175 w185 w192 w199 w214 w220 w222 w252 w281 w293 w305 w313 w345 w359] -> w27
          tunnel: w26 -> [w33 w54 w64 w73 w78 w86 w91 w96 w100 w105 w110 w115 w119 w140 w146 w152 w158 w163 w168 w173 w178 w186 w189 w198 w211 w216 w227 w257 w284 w292 w304 w312 w344 w354]
          tunnel: [w30 w55 w65 w72 w77 w85 w90 w92 w101 w106 w111 w116 w120 w141 w142 w148 w156 w164 w169 w174 w179 w187 w190 w193 w212 w217 w231 w261 w285 w286 w299 w310 w336 w358] -> w25
          tunnel: w22 -> [w30 w55 w65 w72 w77 w85 w90 w92 w101 w106 w111 w116 w121 w141 w144 w151 w157 w164 w169 w174 w179 w187 w191 w195 w213 w219 w230 w260 w285 w287 w300 w311 w338 w358]
          tunnel: [w32 w54 w64 w73 w78 w86 w91 w96 w100 w105 w110 w115 w119 w140 w146 w152 w158 w163 w168 w173 w178 w186 w189 w198 w211 w216 w228 w258 w284 w292 w304 w312 w344 w354] -> w24
          tunnel: w20 -> [_ w51 w61 _ _ _ _ _ _ _ _ _ _ _ _ _ _ _ _ _ _ _ _ _ _ _ _ _ _ _ _ _ _ _]
          event Timeout {
            n8 = event-data() -> ()  [unwired: 1 in, 1 out]
            n9 = Unbundle By Name(w33) -> ("Last Periodic Update"=w29:u32, "Connected"=w31:bool)
            n10 = case shown="True" w31 {
              selector: w31 -> [w36 w39]
              tunnel: w35 -> [w38 w43]
              tunnel: [w38 w42] -> w34
              tunnel: w33 -> [w37 w45]
              tunnel: [w37 w44] -> w32
              tunnel: w29 -> [_ w41]
              frame False {
                n11 = local write "System Power"(w36) -> ()
                n12 = local write "Output Enabled"(w36) -> ()
                n13 = local write "Output Disabled"(w36) -> ()
              }
              frame True {
                n14 = call "Queue Periodic Updates.vi"("Last Periodic Update in"=w41, "Remaining States"=w43) -> ("Last Periodic Update out"=w40:u32, "States Out"=w42:string)  [unwired: 8 in]
                n15 = local write "System Power"(w39) -> ()
                n16 = Bundle By Name(cluster=w45, "Last Periodic Update"=w40) -> (w44:T13)
              }
            }
          }
          event User Event {
            (unwired) T14."Enabled" ("Disabled")
            n17 = event-data() -> ("String"=w50:string)  [unwired: 1 in]
            n18 = Format Into String(format string="%s:  EIS Profile Completed - %s", w51, w50) -> (resulting string=w53:string)  [unwired: 2 in, 1 out]
            n19 = local write "Toggle EIS Profile"(FALSE ("Toggle EIS Profile")) -> ()
            n20 = call <vilib>:"Add State(s) to Queue__jki_lib_state_machine.vi"("State(s) in Front (\"\")"="UI: Stop Profile", "State(s) in (\"\")"=w48) -> ("States Out"=w46:string)  [unwired: 13 in]
            n21 = local write "Status Message"(w53) -> ()
          }
          event User Event {
            (unwired) T14."Enabled" ("Disabled")
            n22 = event-data() -> ("String"=w60:string)  [unwired: 1 in]
            n23 = Format Into String(format string="%s:  DCIR Profile Completed - %s", w61, w60) -> (resulting string=w63:string)  [unwired: 2 in, 1 out]
            n24 = local write "Toggle HPPC Profile"(FALSE ("Toggle EIS Profile")) -> ()
            n25 = call <vilib>:"Add State(s) to Queue__jki_lib_state_machine.vi"("State(s) in Front (\"\")"="UI: Stop Profile", "State(s) in (\"\")"=w59) -> ("States Out"=w57:string)  [unwired: 13 in]
            n26 = local write "Status Message"(w63) -> ()
          }
          event "PMOD Connect": Value Change {
            n27 = event-data() -> ("NewVal"=w69:bool)  [unwired: 1 in]
            n28 = Select(t="Macro: Connect", s=w69, f="Macro: Disconnect") -> (s? t:f=w66:string)
            n29 = call <vilib>:"Add State(s) to Queue__jki_lib_state_machine.vi"("State(s) in Front (\"\")"=w66, "State(s) in (\"\")"=w71) -> ("States Out"=w70:string)  [unwired: 13 in]
          }
          event "Module Selection": Value Change {
            n30 = event-data() -> ()  [unwired: 1 in, 1 out]
            n31 = call <vilib>:"Add State(s) to Queue__jki_lib_state_machine.vi"("State(s) in Front (\"\")"="Data: Select Power Module ", "State(s) in (\"\")"=w76) -> ("States Out"=w75:string)  [unwired: 13 in]
          }
          event "PMOD Reserve": Value Change {
            n32 = event-data() -> ("NewVal"=w82:bool)  [unwired: 1 in]
            n33 = Select(t="Macro: Reserve", s=w82, f="Macro: Unreserve") -> (s? t:f=w79:string)
            n34 = call <vilib>:"Add State(s) to Queue__jki_lib_state_machine.vi"("State(s) in Front (\"\")"=w79, "State(s) in (\"\")"=w84) -> ("States Out"=w83:string)  [unwired: 13 in]
          }
          event "PMOD Clear": Value Change {
            n35 = event-data() -> ()  [unwired: 1 in, 1 out]
            n36 = call <vilib>:"Add State(s) to Queue__jki_lib_state_machine.vi"("State(s) in Front (\"\")"="PMOD: Clear", "State(s) in (\"\")"=w89) -> ("States Out"=w88:string)  [unwired: 13 in]
          }
          event "Apply Mode & Range": Value Change {
            n37 = event-data() -> ()  [unwired: 1 in, 1 out]
            n38 = call <vilib>:"Add State(s) to Queue__jki_lib_state_machine.vi"("State(s) in Front (\"\")"="PMOD: Set Mode and Range", "State(s) in (\"\")"=w95) -> ("States Out"=w94:string)  [unwired: 13 in]
          }
          event "Apply Limits": Value Change {
            n39 = event-data() -> ()  [unwired: 1 in, 6 out]
            n40 = call <vilib>:"Add State(s) to Queue__jki_lib_state_machine.vi"("State(s) in Front (\"\")"="PMOD: Set Limits" ("State(s) in Front (\"\")"), "State(s) in (\"\")"=w99) -> ("States Out"=w98:string)  [unwired: 13 in]
          }
          event "Energize": Value Change {
            n41 = event-data() -> ()  [unwired: 1 in, 6 out]
            n42 = call <vilib>:"Add State(s) to Queue__jki_lib_state_machine.vi"("State(s) in Front (\"\")"="PMOD: Energize" ("State(s) in Front (\"\")"), "State(s) in (\"\")"=w104) -> ("States Out"=w103:string)  [unwired: 13 in]
          }
          event "Output": Value Change {
            n43 = event-data() -> ()  [unwired: 1 in, 6 out]
            n44 = call <vilib>:"Add State(s) to Queue__jki_lib_state_machine.vi"("State(s) in Front (\"\")"="PMOD: Output" ("State(s) in Front (\"\")"), "State(s) in (\"\")"=w109) -> ("States Out"=w108:string)  [unwired: 13 in]
          }
          event "Apply Setpoints": Value Change {
            n45 = event-data() -> ()  [unwired: 1 in, 6 out]
            n46 = call <vilib>:"Add State(s) to Queue__jki_lib_state_machine.vi"("State(s) in Front (\"\")"="PMOD: Apply Setpoints" ("State(s) in Front (\"\")"), "State(s) in (\"\")"=w114) -> ("States Out"=w112:string)  [unwired: 13 in]
          }
          event "Acknowledge Faults": Value Change {
            n47 = event-data() -> ()  [unwired: 1 in, 1 out]
            n48 = Unbundle By Name(w119) -> ("Power Module"=w118:refnum<class "PowerModuleInterface.lvclass">, "Reserved"=w117:bool)
            n49 = case shown="True" w117 {
              tunnel: w121 -> [w124 w129]
              tunnel: [w123 w130] -> w120
              tunnel: w118 -> [_ w127]
              frame False {
                n50 = call "Dialog Launcher.vi"("error in (no error)"=w124, "Message"="You must first connect to and then reserve a power module before you can acknowledge faults.", "Title"="Power Module Not Reserved") -> ("error out"=w123:errorcluster)  [unwired: 8 in]
              }
              frame True {
                n51 = call-dynamic "Acknowledge Faults.vi"("object in"=w127, "Error In"=w129) -> ("Error Out"=w128:errorcluster)  [unwired: 12 in, 1 out]
                n52 = case shown="No Error" w128 {
                  selector: w128 -> [w132 w133]
                  tunnel: [w132 w133] -> w130
                  frame No Error {
                    n53 = local write "Fault Message"("" ("Fault Message")) -> ()
                  }
                  frame Error {
                  }
                }
              }
            }
          }
          event "Start Profile": Value Change {
            n54 = event-data() -> ()  [unwired: 1 in, 1 out]
            n55 = Select(t="Macro: Start Setpoint Stream" ("State(s) in Front (\"\")"), s="Start Profile", f="Macro: Stop Setpoint Stream" ("State(s) in Front (\"\")")) -> (s? t:f=w134:string)
            n56 = call <vilib>:"Add State(s) to Queue__jki_lib_state_machine.vi"("State(s) in Front (\"\")"=w134, "State(s) in (\"\")"=w139) -> ("States Out"=w138:string)  [unwired: 13 in]
          }
          event "Use Local Time": Value Change {
            n57 = event-data() -> ("NewVal"=w143:bool)  [unwired: 1 in]
            n58 = Unbundle By Name(w146) -> ("Grapher Ref"=w145:refnum<class "Grapher.lvclass">)
            n59 = call "Set Time Selector.vi"("reference in"=w145, "Use Local Time?"=w143, "Error In"=w144) -> ("Error Out"=w142:errorcluster)  [unwired: 15 in, 1 out]
          }
          event "Graph Samples": Value Change {
            n60 = event-data() -> ("NewVal"=w149:u32)  [unwired: 1 in]
            n61 = Unbundle By Name(w152) -> ("Grapher Ref"=w150:refnum<class "Grapher.lvclass">)
            n62 = call "Set Graph Samples.vi"("reference in"=w150, "Graph Samples"=w149, "Error In"=w151) -> ("Error Out"=w148:errorcluster)  [unwired: 15 in, 1 out]
          }
          event "Graph Data Decimation": Value Change {
            n63 = event-data() -> ("NewVal"=w154:i32)  [unwired: 1 in]
            n64 = Unbundle By Name(w158) -> ("Grapher Ref"=w155:refnum<class "Grapher.lvclass">)
            n65 = call "Set Graph Decimation.vi"("reference in"=w155, "Graph Decimation"=w154, "Error In"=w157) -> ("Error Out"=w156:errorcluster)  [unwired: 15 in, 1 out]
          }
          event "CSV Profile Path": Value Change {
            n66 = event-data() -> ()  [unwired: 1 in, 1 out]
            n67 = call <vilib>:"Add State(s) to Queue__jki_lib_state_machine.vi"("State(s) in Front (\"\")"="Profile: Load" ("State(s) in Front (\"\")"), "State(s) in (\"\")"=w162) -> ("States Out"=w160:string)  [unwired: 13 in]
          }
          event "Apply Slew Rates": Value Change {
            n68 = event-data() -> ()  [unwired: 1 in, 1 out]
            n69 = call <vilib>:"Add State(s) to Queue__jki_lib_state_machine.vi"("State(s) in Front (\"\")"="PMOD: Write Slew Rates", "State(s) in (\"\")"=w166) -> ("States Out"=w165:string)  [unwired: 13 in]
          }
          event "Generate EIS Profile": Value Change {
            (unwired) T14."Disabled and Grayed Out" ("Disabled")
            n70 = event-data() -> ()  [unwired: 1 in, 1 out]
            n71 = call <vilib>:"Add State(s) to Queue__jki_lib_state_machine.vi"("State(s) in Front (\"\")"="EIS: Generate Profile", "State(s) in (\"\")"=w171) -> ("States Out"=w170:string)  [unwired: 13 in]
          }
          event "Generate HPPC Profile": Value Change {
            (unwired) T14."Disabled and Grayed Out" ("Disabled")
            n72 = event-data() -> ()  [unwired: 1 in, 1 out]
            n73 = call <vilib>:"Add State(s) to Queue__jki_lib_state_machine.vi"("State(s) in Front (\"\")"="HPPC: Generate Profile", "State(s) in (\"\")"=w176) -> ("States Out"=w175:string)  [unwired: 13 in]
          }
          event "Start Logging": Value Change {
            n74 = event-data() -> ("NewVal"=w183:bool)  [unwired: 1 in]
            n75 = Select(t="Script: Start Logger", s=w183, f="Script: Stop Logger") -> (s? t:f=w180:string)
            n76 = call <vilib>:"Add State(s) to Queue__jki_lib_state_machine.vi"("State(s) in Front (\"\")"=w180, "State(s) in (\"\")"=w184) -> ("States Out"=w185:string)  [unwired: 13 in]
          }
          event "Save Chart": Value Change {
            n77 = event-data() -> ()  [unwired: 1 in, 1 out]
            n78 = Unbundle By Name(w189) -> ("Grapher Ref"=w188:refnum<class "Grapher.lvclass">)
            n79 = call "Save Chart.vi"("reference in"=w188, "Error In"=w191) -> ("Error Out"=w190:errorcluster)  [unwired: 16 in, 1 out]
          }
          event "Log File Directory": Value Change {
            n80 = event-data() -> ("NewVal"=w200:path)  [unwired: 1 in]
            n81 = Unbundle By Name(w198) -> ("Logger Ref"=w194:refnum<class "Logger.lvclass">)
            n82 = Equal?(x=refnum<class "Logger.lvclass"> refnum, y=w194) -> (x = y?=w196:bool)
            n83 = case shown="False" w196 {
              tunnel: w200 -> [w201 _]
              tunnel: w195 -> [w204 w209]
              tunnel: w194 -> [w202 _]
              tunnel: [w203 w209] -> w193
              frame False {
                n84 = call "Update Log Directory.vi"("reference in"=w202, "Log Directory"=w201, "Error In"=w204) -> ("Error Out"=w203:errorcluster)  [unwired: 15 in, 1 out]
                n85 = Empty String/Path?(string/path=w201) -> (empty?=w205:bool)
                n86 = Select(t=T14."Disabled and Grayed Out" ("Disabled"), s=w205, f=T14."Enabled" ("Disabled")) -> (s? t:f=w206:T14)
                n87 = property on="Start Logging" class="Bool (strict)"("DisabledEnum"=w206) -> ()  [unwired: 2 in, 2 out]
              }
              frame True {
              }
            }
          }
          event "Erase Chart": Value Change {
            n88 = event-data() -> ()  [unwired: 1 in, 1 out]
            n89 = Unbundle By Name(w211) -> ("Grapher Ref"=w210:refnum<class "Grapher.lvclass">)
            n90 = call "Erase Chart.vi"("reference in"=w210, "Error In"=w213) -> ("Error Out"=w212:errorcluster)  [unwired: 16 in, 1 out]
          }
          event "Pause Chart": Value Change {
            n91 = event-data() -> ("NewVal"=w218:bool)  [unwired: 1 in]
            n92 = Unbundle By Name(w216) -> ("Grapher Ref"=w215:refnum<class "Grapher.lvclass">)
            n93 = call "Set Pause.vi"("reference in"=w215, "Set Pause"=w218, "Error In"=w219) -> ("Error Out"=w217:errorcluster)  [unwired: 15 in, 1 out]
          }
          event "Toggle EIS Profile": Value Change {
            n94 = event-data() -> ("NewVal"=w226:bool)  [unwired: 1 in]
            n95 = Unbundle By Name(w227) -> ("EIS Ref"=w232:refnum<class "ACIR_EIS.lvclass">, "EIS Profile Completed"=w224:refnum<user-event>)
            n96 = call <vilib>:"Conditional State String__jki_lib_state_machine.vi"("Do State(s)?"=w226, "State"="Events: Register") -> ("State Out"=w234:string)  [unwired: 7 in]
            n97 = case shown="False" w226 {
              tunnel: w230 -> [w240 w250]
              tunnel: [w238 w248] -> w229
              tunnel: [w241 w247] -> w225
              tunnel: w224 -> [w237 _]
              tunnel: ["UI: Stop Profile" ("State") "UI: Start Profile" ("State")] -> w221
              frame False {
                w241 = refnum<user-event> refnum ("x")
                n98 = Equal?(x=w241, y=w237) -> (x = y?=w239:bool)
                n99 = case shown="False" w239 {
                  tunnel: w240 -> [w244 w245]
                  tunnel: [w242 w245] -> w238
                  tunnel: w237 -> [w243 _]
                  frame False {
                    n100 = Destroy User Event(user event=w243, error in=w244) -> (error out=w242:errorcluster)
                  }
                  frame True {
                  }
                }
              }
              frame True {
                (unwired) T14."Disabled and Grayed Out" ("Disabled")
                w249 = ""  # Message
                n101 = Create User Event(user event datatype=w249, error in=w250) -> (user event=w247:refnum<user-event>, error out=w248:errorcluster)
              }
            }
            n102 = call <vilib>:"Add State(s) to Queue__jki_lib_state_machine.vi"("State(s) in Front (\"\")"=w234, "State(s) in (\"\")"=w235) -> ("States Out"=w223:string)  [unwired: 13 in]
            n103 = call <vilib>:"Add State(s) to Queue__jki_lib_state_machine.vi"("State(s) in Front (\"\")"=w221, "State(s) in (\"\")"=w223) -> ("States Out"=w222:string)  [unwired: 13 in]
            n104 = call "Start Stop Profile.vi"("reference in"=w232, "Start Stop Profile"=w226, "Profile Complete Event"=w225, "Error In"=w229) -> ("Error Out"=w231:errorcluster)  [unwired: 10 in, 1 out]
            n105 = Bundle By Name(cluster=w227, "EIS Profile Completed"=w225) -> (w228:T13)
          }
          event "Toggle HPPC Profile": Value Change {
            n106 = event-data() -> ("NewVal"=w256:bool)  [unwired: 1 in]
            n107 = Unbundle By Name(w257) -> ("HPPC Ref"=w262:refnum<class "DCIR_HPPC.lvclass">, "DCIR Profile Completed"=w254:refnum<user-event>)
            n108 = call <vilib>:"Conditional State String__jki_lib_state_machine.vi"("Do State(s)?"=w256, "State"="Events: Register") -> ("State Out"=w264:string)  [unwired: 7 in]
            n109 = case shown="False" w256 {
              tunnel: w260 -> [w270 w280]
              tunnel: [w268 w278] -> w259
              tunnel: [w271 w277] -> w255
              tunnel: w254 -> [w267 _]
              tunnel: ["UI: Stop Profile" ("State") "UI: Start Profile" ("State")] -> w251
              frame False {
                w271 = refnum<user-event> refnum ("x")
                n110 = Equal?(x=w271, y=w267) -> (x = y?=w269:bool)
                n111 = case shown="False" w269 {
                  tunnel: w270 -> [w274 w275]
                  tunnel: [w272 w275] -> w268
                  tunnel: w267 -> [w273 _]
                  frame False {
                    n112 = Destroy User Event(user event=w273, error in=w274) -> (error out=w272:errorcluster)
                  }
                  frame True {
                  }
                }
              }
              frame True {
                (unwired) T14."Disabled and Grayed Out" ("Disabled")
                w279 = ""  # Message
                n113 = Create User Event(user event datatype=w279, error in=w280) -> (user event=w277:refnum<user-event>, error out=w278:errorcluster)
              }
            }
            n114 = call <vilib>:"Add State(s) to Queue__jki_lib_state_machine.vi"("State(s) in Front (\"\")"=w264, "State(s) in (\"\")"=w265) -> ("States Out"=w253:string)  [unwired: 13 in]
            n115 = call <vilib>:"Add State(s) to Queue__jki_lib_state_machine.vi"("State(s) in Front (\"\")"=w251, "State(s) in (\"\")"=w253) -> ("States Out"=w252:string)  [unwired: 13 in]
            n116 = call "Start Stop Profile.vi"("reference in"=w262, "Start Stop Profile"=w256, "Profile Complete Event"=w255, "Error In"=w259) -> ("Error Out"=w261:errorcluster)  [unwired: 10 in, 1 out]
            n117 = Bundle By Name(cluster=w257, "DCIR Profile Completed"=w255) -> (w258:T13)
          }
          event "Launch Battery Simulation": Value Change {
            n118 = event-data() -> ()  [unwired: 1 in, 6 out]
            n119 = call <vilib>:"Add State(s) to Queue__jki_lib_state_machine.vi"("State(s) in Front (\"\")"="Script: Stop Battery\nScript: Launch Battery", "State(s) in (\"\")"=w283) -> ("States Out"=w281:string)  [unwired: 13 in]
          }
          event "Enable Battery Simulation": Value Change {
            n120 = event-data() -> ("NewVal"=w288:bool)  [unwired: 1 in]
            n121 = Unbundle By Name(w292) -> ("Battery Ref"=w290:refnum<class "Battery.lvclass">)
            n122 = Equal?(x=refnum<class "Battery.lvclass"> refnum, y=w290) -> (x = y?=w289:bool)
            n123 = case shown="False" w289 {
              tunnel: w290 -> [w297 _]
              tunnel: w288 -> [w296 _]
              tunnel: w287 -> [w295 w298]
              tunnel: [w294 w298] -> w286
              frame False {
                n124 = call-dynamic "Enable.vi"("reference in"=w297, "Enable"=w296, "Error In"=w295) -> ("Error Out"=w294:errorcluster)  [unwired: 15 in, 1 out]
              }
              frame True {
              }
            }
          }
          event "Reset Battery Simulation": Value Change {
            n125 = event-data() -> ()  [unwired: 1 in, 1 out]
            n126 = Unbundle By Name(w304) -> ("Battery Ref"=w302:refnum<class "Battery.lvclass">)
            n127 = Equal?(x=refnum<class "Battery.lvclass"> refnum, y=w302) -> (x = y?=w301:bool)
            n128 = case shown="False" w301 {
              tunnel: w302 -> [w308 _]
              tunnel: w300 -> [w307 w309]
              tunnel: [w306 w309] -> w299
              frame False {
                n129 = call-dynamic "Reset Simulation.vi"("reference in"=w308, "Error In"=w307) -> ("Error Out"=w306:errorcluster)  [unwired: 15 in, 2 out]
              }
              frame True {
              }
            }
          }
          event "TDMS Viewer": Value Change {
            n130 = event-data() -> ()  [unwired: 1 in, 1 out]
            n131 = disable-structure shown="TARGET_TYPE==RT" {
              disable-tunnel: w311 -> [w315 w335]
              disable-tunnel: [w314 w335] -> w310
              frame condition #0 (active) {
                n132 = call "File Dialog"("error in"=w315) -> ("selected path"=w316:path, "cancelled"=w317:bool, "error out"=w318:errorcluster)  [unwired: 11 in, 1 out]
                n133 = case shown="No Error" w318 {
                  selector: w318 -> [w319 _]
                  tunnel: w316 -> [w322 _]
                  tunnel: [w321 errorcluster {"status"=FALSE, "code"=0, "source"=""} ("error IO")] -> w314
                  tunnel: w317 -> [w320 _]
                  frame No Error {
                    n134 = case shown="False" w320 {
                      tunnel: w319 -> [w332 w333]
                      tunnel: w322 -> [w325 _]
                      tunnel: [w323 w333] -> w321
                      frame False {
                        w327 = 128  # call & forget
                        n135 = vi-ref "NI_TDMS File Viewer.lvlib:TDMS - File Viewer (NXG Style).vi"() -> (w331:refnum<vi>)
                        n136 = property class="VI Interface Type 4"(reference=w331, error in=w332) -> (reference out=w329:refnum<vi>, error out=w330:errorcluster, "Path"=w328:path)
                        n137 = Open VI Reference(type specifier VI Refnum (for type only)=w329, vi path=w328, options=w327, error in (no error)=w330) -> (vi reference=w326:refnum<vi>, error out=w324:errorcluster)  [unwired: 2 in]
                        n138 = call-by-ref "Start Asynchronous Call"(reference=w326, error in=w324, "error in"=w324, "file in"=w325) -> (error out=w323:errorcluster)  [unwired: 8 in, 3 out]
                      }
                      frame True {
                      }
                    }
                  }
                  frame Error {
                  }
                }
              }
              frame condition #1 {
              }
            }
          }
          event "Get Events": Value Change {
            w343 = 200  # Number of Events
            # "limit to the most recent 200 events to prevent\ntaking unnecessary memory space for old\nhistory"
            n139 = event-data() -> ()  [unwired: 1 in, 6 out]
            n140 = call <vilib>:"Set Busy.vi"("error in (no error)"=w338) -> ("error out"=w337:errorcluster)  [unwired: 9 in, 1 out]
            n141 = call "Get System Events.vi"("error in (no error)"=w337) -> ("error out"=w340:errorcluster, "system events"=w342:cluster{"timestamp":string, "message":string}[])  [unwired: 9 in]
            n142 = for {
              N: w343 -> [_]
              tunnel: w342 -> [w351]
              tunnel: [w346] -> w341 mode=indexing
              i -> [w350]
              n143 = Index Array(array=w351, index=w350) -> (element=w349:cluster{"timestamp":string, "message":string})
              n144 = Unbundle By Name(w349) -> ("message"=w348:string, "timestamp"=w347:string)
              n145 = Build Array(w348, w347) -> (w346:string[])
            }
            n146 = property on="Events" class="MCListbox (strict)"(error in=w340, "ItemNames"=w341) -> (error out=w339:errorcluster)  [unwired: 1 in, 1 out]
            n147 = call <vilib>:"Unset Busy.vi"("error in (no error)"=w339) -> ("error out"=w336:errorcluster)  [unwired: 10 in]
          }
          event Panel Close? {
            # "Close Panel button (pressed) Event\n(this executes Macro: Exit to terminate the VI)"
            n148 = event-data() -> ()  [unwired: 1 in, 1 out]
            n149 = Unbundle By Name(w354) -> ("Connected"=w353:bool)
            n150 = case shown="False" w353 {
              tunnel: [TRUE ("T button?") w362] -> w356
              frame False {
              }
              frame True {
                n151 = Two Button Dialog(message="Are you sure you want to close Volta Control Suite?  Your control to the power module will be relinquished which could impact connected devices.", 1:"No" ("F button name (\"Cancel\")"), 2:"Yes" ("T button name (\"OK\")")) -> (T button?=w362:bool)
              }
            }
            n152 = call <vilib>:"Conditional State String__jki_lib_state_machine.vi"("Do State(s)?"=w356, "State"="Macro: Exit") -> ("State Out"=w355:string)  [unwired: 7 in]
            n153 = call <vilib>:"Add State(s) to Queue__jki_lib_state_machine.vi"("State(s) in Front (\"\")"=w355, "State(s) in (\"\")"=w360) -> ("States Out"=w359:string)  [unwired: 13 in]
            n154 = event-data("Discard?"=TRUE) -> ()  [unwired: 1 in, 1 out]
          }
        }
      }
      frame "---------- Core ----------" {
        # "Do not put any code in this frame.\n(it is a separator no-op)"
        n155 = call <vilib>:"Add State(s) to Queue__jki_lib_state_machine.vi"("State(s) in (\"\")"=w370) -> ("States Out"=w369:string)  [unwired: 14 in]
      }
      frame Default {
        w381 = 42 items=["No error", "Argument error", "Memory is full", "Out of zone", "End of file", "File already open", "Generic file I/O error", "File not found", "File permission error", "Disk is full", "Duplicate path", "Too many files open", "System feature not enabled", "Resource file not found", "Cannot add resource", "Resource not found", "Image not found", "Image memory error", "Pen does not exist", "Config type invalid", "Config token not found", "Config parse error", "Config memory error", "Bad external code format", "Bad external code offset", "External code not present", "Null window", "Destroy window error", "Null menu", "Print aborted", "Bad print record", "Print driver error", "Windows error during printing", "Memory error during printing", "Print dialog error", "Generic print error", "Invalid device refnum", "Device not found", "Device parameter error", "Device unit error", "Cannot open device", "Device call aborted", "Generic error", "Cancelled by user", "Object ID too low", "Object ID too high", "Object not in heap", "Unknown heap", "Unknown object (invalid DefProc)", "Unknown object (DefProc not in table)", "Message out of range", "Invalid (null) method", "Unknown message", "Manager call not supported", "Bad address", "Network operation in progress", "Network operation timed out", "Connection is busy", "Network attribute not supported", "Network error", "Address in use", "System out of memory", "Connection aborted", "Connection refused", "Not connected", "Already connected", "Connection closed", "Initialization error (interapplication manager)", "Bad occurrence", "Wait on unbound occurrence handler", "Occurrence queue overflow", "Datalog type conflict", "Unused", "Unrecognized type (interapplication manager)", "Memory corrupt", "Failed to make temporary DLL", "Old CIN version", "Drag socket not found", "Failed to load drop-object", "Failed to register OLE object", "Failed to release OLE object", "Format specifier type mismatch", "Unknown format specifier", "Too few format specifiers", "Too many format specifiers", "Scan failed", "Newer CIN version", "Error converting to variant", "Runtime menu error", "Password tampered", "Variant attribute not found", "Incompatible variant data type", "Event data is not available", "Event Store is not present", "Occurrence is not found", "Event Queue is not created", "Event info is not available", "Refnum passed is NULL", "Error retrieving Class GUID", "Error retrieving CoClass GUID", "Error retrieving TypeLib GUID.", "Bad built application magic bytes.", "Specific driver is different from the specific driver associated with the Logical Name.", "There is no session opened to the class driver.", "Max Error", "MAX - Error with config objects", "MAX - Error loading configuration", "MAX - Group not supported"]
        # "Current State"
        # "Do not delete, rename, or modify this frame.\n(this is used to capture unhandled states and typos)"
        # "Handle mistyped state name (developer tool)"
        n156 = Format Into String(format string="Software Exception: Unhandled State \"%s\"." ("message"), error in=w377, w372) -> (resulting string=w380:string, error out=w379:errorcluster)  [unwired: 1 in]
        n157 = call <vilib>:"Error Cluster From Error Code.vi"("show call chain? (False)"=TRUE, "error in (no error)"=w379, "error message (\"\")"=w380, "error code (0)"=w381) -> ("error out"=w378:errorcluster)  [unwired: 5 in]
        n158 = call <vilib>:"Add State(s) to Queue__jki_lib_state_machine.vi"("State(s) in (\"\")"=w376) -> ("States Out"=w375:string)  [unwired: 14 in]
      }
      frame "Initialize Core Data" {
        # "Do not delete, rename, or modify this frame.\n(this is used to determine panel behavior on exit)"
        # "originally closed?"
        # "exe?"
        # "If panel starts closed or is an EXE, then close it when we exit"
        n159 = property class="VI"() -> ("FP.State"=w387:T15)  [unwired: 2 in, 2 out]
        n160 = property class="App"() -> ("App.Kind"=w393:T16)  [unwired: 2 in, 2 out]
        n161 = control-ref of="Current VI Reference"() -> (w388:refnum<vi>)
        n162 = Equal?(x=w387, y=T15."Closed" ("Front Panel Window:State")) -> (x = y?=w385:bool)
        n163 = Equal?(x=w393, y=T16."Run Time System" ("Application:Kind")) -> (x = y?=w391:bool)
        n164 = Or(x=w385, y=w391) -> (x .or. y?=w389:bool)
        n165 = call <vilib>:"Add State(s) to Queue__jki_lib_state_machine.vi"("State(s) in (\"\")"=w396) -> ("States Out"=w395:string)  [unwired: 14 in]
        n166 = Bundle By Name(cluster=w390, "Core.Current VI Reference"=w388, "Core.Close Panel on Exit?"=w389) -> (w394:T13)
      }
      frame "Error Handler" {
        # "When running as sourcecode, this function will add previous state data to the error message to aid the developer in troubleshoot errors.\nIf run as an executable, no additional information is added to the error message."
        # "This state receives both Errors and Warnings which is how the Status of this wire can be FALSE"
        # "Unhandled Error -- Display it"
        # "Handle any errors or warnings here.\nYou can also output any states to clean-up after errors or warnings occur"
        # "Clear error or warning"
        n167 = disable-structure shown="Default" {
          disable-tunnel: w403 -> [w410 w411]
          disable-tunnel: w402 -> [w409 _]
          disable-tunnel: [w408 w411] -> w401
          frame condition #0 (active) {
            n168 = call <vilib>:"Append Error Details__jki_lib_state_machine.vi"("error in (no error)"=w410, "Previous State and Argument(s)"=w409) -> ("error out"=w408:errorcluster)  [unwired: 9 in]
          }
          frame condition #1 {
          }
        }
        n169 = call <vilib>:"General Error Handler.vi"("error in (no error)"=w401) -> ()  [unwired: 10 in, 5 out]
        n170 = call-poly <vilib>:"Select State(s)__jki_lib_state_machine.vi"("State(s) if True (\"\")"="/* Post Error States", "Select"=w401, "State(s) if False (\"\")"="/* Post Warning States") -> ("States Out"=w399:string)  [unwired: 12 in]
        n171 = call <vilib>:"Add State(s) to Queue__jki_lib_state_machine.vi"("State(s) in Front (\"\")"=w399, "State(s) in (\"\")"=w407) -> ("States Out"=w406:string)  [unwired: 13 in]
      }
      frame "Exit" {
        # "Do not put any code in this frame.\n(No errors that occur here will be handled.)"
        n172 = call <vilib>:"Add State(s) to Queue__jki_lib_state_machine.vi"("State(s) in (\"\")"=w417) -> ("States Out"=w416:string)  [unwired: 14 in]
      }
      frame "---------- Data ----------" {
        # "Do not put any code in this frame.\n(It is a separator no-op. You can make a copy of this frame to create a new Data frame)"
        n173 = call <vilib>:"Add State(s) to Queue__jki_lib_state_machine.vi"("State(s) in (\"\")"=w422) -> ("States Out"=w421:string)  [unwired: 14 in]
      }
      frame "Data: Cleanup" {
        # "Cleanup any data and references, here.\n(this is called automatically, by the Macro: Exit)"
        n174 = Unbundle By Name(w452) -> ("Power Module"=w438:refnum<class "PowerModuleInterface.lvclass">, "Logger Ref"=w444:refnum<class "Logger.lvclass">, "Grapher Ref"=w429:refnum<class "Grapher.lvclass">, "Battery Ref"=w433:refnum<class "Battery.lvclass">, "HPPC Ref"=w442:refnum<class "DCIR_HPPC.lvclass">, "EIS Ref"=w450:refnum<class "ACIR_EIS.lvclass">, "Core.Current VI Reference"=w425:refnum<vi>)
        n175 = Equal?(x=w444, y=refnum<class "Logger.lvclass"> refnum ("reference in")) -> (x = y?=w446:bool)
        n176 = Equal?(x=w429, y=refnum<class "Grapher.lvclass"> refnum ("Grapher Ref")) -> (x = y?=w427:bool)
        n177 = Equal?(x=w433, y=refnum<class "Battery.lvclass"> refnum ("Battery Ref")) -> (x = y?=w432:bool)
        n178 = Equal?(x=w438, y=refnum<class "PowerModuleInterface.lvclass"> refnum ("Power Module")) -> (x = y?=w437:bool)
        n179 = Equal?(x=w442, y=refnum<class "DCIR_HPPC.lvclass"> refnum ("DCIR")) -> (x = y?=w441:bool)
        n180 = Equal?(x=refnum<class "ACIR_EIS.lvclass"> refnum, y=w450) -> (x = y?=w447:bool)
        n181 = case shown="False" w437 {
          tunnel: w438 -> [w459 _]
          tunnel: [w458 _] -> w436
          frame False {
            n182 = call-dynamic "Destroy.vi"("object in"=w459) -> ("Error Out"=w458:errorcluster)  [unwired: 13 in, 1 out]
          }
          frame True {
          }
        }
        n183 = case shown="False" w446 {
          tunnel: w444 -> [w463 _]
          tunnel: [w462 _] -> w435
          frame False {
            n184 = call-dynamic "Destroy.vi"("reference in"=w463) -> ("Error Out"=w462:errorcluster)  [unwired: 17 in, 1 out]
          }
          frame True {
          }
        }
        n185 = case shown="False" w427 {
          tunnel: [w455 _] -> w430
          tunnel: w429 -> [w454 _]
          frame False {
            n186 = call-dynamic "Destroy.vi"("reference in"=w454) -> ("Error Out"=w455:errorcluster)  [unwired: 17 in, 1 out]
          }
          frame True {
          }
        }
        n187 = case shown="False" w432 {
          tunnel: [w457 _] -> w431
          tunnel: w433 -> [w456 _]
          frame False {
            n188 = call-dynamic "Battery_Destroy.vi"("reference in"=w456) -> ("Error Out"=w457:errorcluster)  [unwired: 17 in, 1 out]
          }
          frame True {
          }
        }
        n189 = case shown="False" w441 {
          tunnel: w442 -> [w461 _]
          tunnel: [w460 _] -> w440
          frame False {
            n190 = call-dynamic "Destroy.vi"("reference in"=w461) -> ("Error Out"=w460:errorcluster)  [unwired: 17 in, 1 out]
          }
          frame True {
          }
        }
        n191 = case shown="False" w447 {
          tunnel: w450 -> [w465 _]
          tunnel: [w464 _] -> w448
          frame False {
            n192 = call-dynamic "Destroy.vi"("reference in"=w465) -> ("Error Out"=w464:errorcluster)  [unwired: 17 in, 1 out]
          }
          frame True {
          }
        }
        n193 = Merge Errors(w436, w435, w430, w431, w440, w448, w424) -> (w426:errorcluster)
        n194 = Close Reference(reference=w425, error in (no error)=w426) -> (error out=w423:errorcluster)
      }
      frame "Data: Initialize" {
        w470 = T23 {"Current VI Reference"=refnum, "Close Panel on Exit?"=FALSE}  # Core
        n195 = Bundle By Name(cluster=w471, "Core"=w470) -> (w469:T13)
      }
      frame "Data: Update Periodic" {
        n196 = Unbundle By Name(w479) -> ("Connected"=w475:bool, "Power Module"=w474:refnum<class "PowerModuleInterface.lvclass">)
        n197 = Not Equal?(x=w474, y=refnum<class "PowerModuleInterface.lvclass"> refnum) -> (x != y?=w472:bool)
        n198 = And(x=w475, y=w472) -> (x .and. y?=w478:bool)
        n199 = case shown="True" w478 {
          tunnel: w477 -> [w482 w500]
          tunnel: [w482 w516] -> w476
          tunnel: w474 -> [_ w499]
          frame False {
          }
          frame True {
            w505 = T1 {"min"=0.0, "max"=0.0} ("Voltage Range")
            n200 = call-dynamic "Get Limits.vi"("object in"=w499, "Error In"=w500) -> ("Limits"=w513:T24, "Error Out"=w514:errorcluster)  [unwired: 11 in, 1 out]
            n201 = call-dynamic "Get Output Enable.vi"("object in"=w499, "Error In"=w500) -> ("output"=w511:bool, "Error Out"=w512:errorcluster)  [unwired: 11 in, 1 out]
            "Output Enabled" <- w511
            n202 = call-dynamic "Get Faults.vi"("object in"=w499, "Error In"=w500) -> ("active faults"=w493:string[], "fault"=w496:bool, "Error Out"=w498:errorcluster)  [unwired: 10 in, 1 out]
            "Fault" <- w496
            n203 = call-dynamic "Get Mode.vi"("object in"=w499, "Error In"=w500) -> ("mode"=w497:string, "Error Out"=w510:errorcluster)  [unwired: 11 in, 1 out]
            n204 = call-dynamic "Get Range.vi"("object in"=w499, "Error In"=w500) -> ("Range"=w508:T19, "Error Out"=w509:errorcluster)  [unwired: 11 in, 1 out]
            n205 = Unbundle By Name(w508) -> ("Current Max (A)"=w507:dbl, "Current Min (A)"=w506:dbl, "Voltage Max (V)"=w504:dbl, "Voltage Min (V)"=w503:dbl)
            n206 = Not(x=w511) -> (.not. x?=→"Output Disabled":bool)
            n207 = Unbundle By Name(w513) -> ("Current Max (A)"=→"Current Maximum":dbl, "Current Min (A)"=→"Current Minimum":dbl, "Voltage Max (V)"=→"Voltage Maximum":dbl, "Voltage Min (V)"=→"Voltage Minimum":dbl, "Power Max (W)"=w522:dbl, "Power Min (W)"=w520:dbl)
            n208 = Array To Spreadsheet String(delimiter (Tab)=",", array=w493, 3:"%s" ("format string")) -> (spreadsheet string=w484:string)
            n209 = Array Size(array=w493) -> (size(s)=w492:i32)
            n210 = local write "MODE"(w497) -> ()
            n211 = Search and Replace String(input string=w484, search string="\r") -> (result string=w483:string)  [unwired: 6 in, 3 out]
            n212 = property on="CURRENT" class="Knob (strict)"("Scale.Maximum"=w507, "Scale.Minimum"=w506) -> ()  [unwired: 2 in, 2 out]
            n213 = property on="VOLTAGE" class="Knob (strict)"("Scale.Maximum"=w504, "Scale.Minimum"=w503) -> ()  [unwired: 2 in, 2 out]
            n214 = Divide(x=w522, y=sgl 1000.0) -> (x/y=→"Power Maximum":dbl)
            n215 = Search and Replace String(input string=w483, search string="\n") -> (result string=w486:string)  [unwired: 6 in, 3 out]
            n216 = Divide(x=w520, y=sgl 1000.0) -> (x/y=→"Power Minimum":dbl)
            n217 = Bundle By Name(cluster=w505, "max"=w507, "min"=w506) -> (→"Current Range":T1)
            n218 = Bundle By Name(cluster=w505, "max"=w504, "min"=w503) -> (→"Voltage Range":T1)
            n219 = Format Into String(format string="%d active fault(s) on power module\\r\\n%s", w492, w486) -> (resulting string=w489:string)  [unwired: 2 in, 1 out]
            n220 = Select(t=w489, s=w496, f="") -> (s? t:f=w488:string)
            n221 = local write "Fault Message"(w488) -> ()
            n222 = Merge Errors(w498, w510, w509, w514, w512) -> (w516:errorcluster)
          }
        }
      }
      frame "Data: Select Power Module" {
        n223 = local read "Module Selection"() -> (w542:i16)
        n224 = Unbundle By Name(w540) -> ("Plugin Objects"=w543:refnum<class "PowerModuleInterface.lvclass">[])
        n225 = Index Array(array=w543, index=w542) -> (element=w541:refnum<class "PowerModuleInterface.lvclass">)
        n226 = call-dynamic "Create.vi"("object in"=w541, "Error In"=w544) -> ("object out"=w529:refnum<class "PowerModuleInterface.lvclass">, "ProcessVI Ref"=w536:refnum<vi>, "Error Out"=w538:errorcluster)  [unwired: 11 in]
        n227 = call <userlib>:"Fit VI window to Largest Dec__ogtk.vi"("error in (no error)"=w538, "border spacing (2 px)"=-4, "VI Ref (calling VI)"=w536) -> ("error out"=w537:errorcluster, "dup VI Ref"=w535:refnum<vi>)  [unwired: 3 in]
        n228 = invoke on="Module Subpanel" class="SubPnl" method="Insert VI"(error in=w537, "VI Ref"=w535) -> (error out=w533:errorcluster)  [unwired: 2 in, 3 out]
        n229 = case shown="No Error" w533 {
          selector: w533 -> [w567 w584]
          tunnel: [w554 w584] -> w530
          tunnel: [T14."Enabled" ("Disabled") T14."Disabled and Grayed Out" ("Disabled")] -> w532
          tunnel: [T14."Disabled" ("Disabled") T14."Enabled" ("Disabled")] -> w531
          tunnel: w529 -> [w566 _]
          tunnel: [w565 refnum<class "PowerModuleInterface.lvclass"> refnum ("Power Module")] -> w528
          tunnel: [Tabs."MODULE" ("Main Tab Control") Tabs."CONFIG" ("Main Tab Control")] -> w527
          frame No Error {
            w551 = cluster{"String":string, "Value":ext} {"String"="", "Value"=0.0}
            w561 = refnum<vi> refnum  # Ring
            n230 = call-dynamic "Get Capabilities.vi"("object in"=w566, "Error In"=w567) -> ("object out"=w565:refnum<class "PowerModuleInterface.lvclass">, "modes"=w552:string[], "ranges"=w553:string[], "Error Out"=w556:errorcluster)  [unwired: 10 in]
            n231 = for {
              tunnel: w552 -> [w578] mode=indexing
              tunnel: w551 -> [w579]
              tunnel: [w575] -> w549 mode=indexing
              i -> [w577]
              n232 = Increment(x=w577) -> (x+1=w576:i32)
              n233 = Bundle By Name(cluster=w579, "String"=w578, "Value"=w576) -> (w575:cluster{"String":string, "Value":ext})
            }
            n234 = for {
              tunnel: w553 -> [w573] mode=indexing
              tunnel: w551 -> [w574]
              tunnel: [w570] -> w550 mode=indexing
              i -> [w572]
              n235 = Increment(x=w572) -> (x+1=w571:i32)
              n236 = Bundle By Name(cluster=w574, "String"=w573, "Value"=w571) -> (w570:cluster{"String":string, "Value":ext})
            }
            n237 = property on="Mode & Range" class="Clust (strict)"() -> ("Controls[]"=w564:refnum<vi>[])  [unwired: 2 in, 2 out]
            n238 = Index Array(array=w564) -> (element #1=w563:refnum<vi>, element #2=w562:refnum<vi>)  [unwired: 2 in]
            n239 = To More Specific Class(target class=w561, reference=w563, error in=w556) -> (specific class reference=w559:refnum<vi>, error out=w560:errorcluster)
            n240 = To More Specific Class(target class=w561, reference=w562, error in=w556) -> (specific class reference=w557:refnum<vi>, error out=w558:errorcluster)
            n241 = property class="Ring"(reference=w559, error in=w560, "StringsAndValues[]"=w549) -> (error out=w548:errorcluster)  [unwired: 1 out]
            n242 = property class="Ring"(reference=w557, error in=w558, "StringsAndValues[]"=w550) -> (error out=w555:errorcluster)  [unwired: 1 out]
            n243 = Merge Errors(w548, w555) -> (w554:errorcluster)
          }
          frame Error {
          }
        }
        n244 = property on="PMOD Connect" class="Bool (strict)"("DisabledEnum"=w532) -> ()  [unwired: 2 in, 2 out]
        n245 = local write "Main Tab Control"(w527) -> ()
        n246 = property on="Module Selection" class="Ring (strict)"("DisabledEnum"=w531) -> ()  [unwired: 2 in, 2 out]
        n247 = Bundle By Name(cluster=w540, "Power Module"=w528) -> (w539:T13)
      }
      frame "---------- HPPC ----------" {
        # "Do not put any code in this frame.\n(It is a separator no-op. You can make a copy of this frame to create a new UI frame)"
        n248 = call <vilib>:"Add State(s) to Queue__jki_lib_state_machine.vi"("State(s) in (\"\")"=w589) -> ("States Out"=w588:string)  [unwired: 14 in]
      }
      frame "HPPC: Generate Profile" {
        n249 = disable-structure shown="TARGET_TYPE==Windows, Default" {
          disable-tunnel: [w613 w620] -> w593
          disable-tunnel: w592 -> [w612 w620]
          disable-tunnel: w591 -> [w611 w619]
          disable-tunnel: [w610 w619] -> w590
          frame condition #0 (active) {
            n250 = Unbundle By Name(w612) -> ("HPPC Ref"=w604:refnum<class "DCIR_HPPC.lvclass">, "Logger Ref"=w599:refnum<class "Logger.lvclass">, "Power Module"=w597:refnum<class "PowerModuleInterface.lvclass">)
            n251 = Equal?(x=refnum<class "DCIR_HPPC.lvclass"> refnum ("DCIR Ref"), y=w604) -> (x = y?=w606:bool)
            n252 = case shown="False" w606 {
              tunnel: w611 -> [w617 w618]
              tunnel: [w615 w618] -> w605
              tunnel: w604 -> [w614 _]
              frame False {
                n253 = invoke on="HPPC Subpanel" class="SubPnl" method="Remove VI"(error in=w617) -> (error out=w616:errorcluster)  [unwired: 2 in, 2 out]
                n254 = call-dynamic "Destroy.vi"("reference in"=w614, "Error In"=w616) -> ("Error Out"=w615:errorcluster)  [unwired: 16 in, 1 out]
              }
              frame True {
              }
            }
            n255 = local read "HPPC Parameters"() -> (w596:T10)
            n256 = call "DCIR_HPPC_Create.vi"("HPPC Parameters"=w596, "Logger"=w599, "Power Module"=w597, "Error In"=w605) -> ("reference out"=w607:refnum<class "DCIR_HPPC.lvclass">, "ProcessViRef"=w608:refnum<vi>, "Error Out"=w609:errorcluster)  [unwired: 9 in]
            n257 = call <userlib>:"Fit VI window to Largest Dec__ogtk.vi"("error in (no error)"=w609, "VI Ref (calling VI)"=w608) -> ("error out"=w603:errorcluster, "dup VI Ref"=w602:refnum<vi>)  [unwired: 4 in]
            n258 = Bundle By Name(cluster=w612, "HPPC Ref"=w607) -> (w613:T13)
            n259 = invoke on="HPPC Subpanel" class="SubPnl" method="Insert VI"(error in=w603, "VI Ref"=w602) -> (error out=w601:errorcluster)  [unwired: 2 in, 3 out]
            n260 = property on="Toggle HPPC Profile" class="Bool (strict)"(error in=w601, "DisabledEnum"=T14."Enabled" ("Disabled")) -> (error out=w610:errorcluster)  [unwired: 1 in, 1 out]
          }
          frame condition #1 {
          }
        }
      }
      frame "HPPC: Load Data" {
        (unwired) T14."Enabled" ("Disabled")
        # "#todo\n\nload TDMS file method on DCIR class"
      }
      frame "HPPC: Generate Report" {
        n261 = disable-structure shown="TARGET_TYPE==Windows, Default" {
          disable-tunnel: w627 -> [w633 _]
          disable-tunnel: w626 -> [w632 w634]
          disable-tunnel: [w631 w634] -> w625
          frame condition #0 (active) {
            n262 = Unbundle By Name(w633) -> ("HPPC Ref"=w630:refnum<class "DCIR_HPPC.lvclass">)
            n263 = call "Generate Plots.vi"("reference in"=w630, "Error In"=w632) -> ("Error Out"=w631:errorcluster)  [unwired: 16 in, 1 out]
          }
          frame condition #1 {
          }
        }
      }
      frame "---------- EIS ----------" {
        # "Do not put any code in this frame.\n(It is a separator no-op. You can make a copy of this frame to create a new UI frame)"
        n264 = call <vilib>:"Add State(s) to Queue__jki_lib_state_machine.vi"("State(s) in (\"\")"=w639) -> ("States Out"=w638:string)  [unwired: 14 in]
      }
      frame "EIS: Generate Profile" {
        n265 = disable-structure shown="TARGET_TYPE==Windows, Default" {
          disable-tunnel: [w670 w680] -> w643
          disable-tunnel: w642 -> [w668 w680]
          disable-tunnel: w641 -> [w663 w679]
          disable-tunnel: [w658 w679] -> w640
          frame condition #0 (active) {
            n266 = Unbundle By Name(w668) -> ("EIS Ref"=w664:refnum<class "ACIR_EIS.lvclass">, "Logger Ref"=w656:refnum<class "Logger.lvclass">)  [unwired: 1 out]
            n267 = Equal?(x=refnum<class "ACIR_EIS.lvclass"> refnum ("y"), y=w664) -> (x = y?=w666:bool)
            n268 = case shown="False" w666 {
              tunnel: w663 -> [w677 w678]
              tunnel: [w675 w678] -> w665
              tunnel: w664 -> [w674 _]
              frame False {
                n269 = invoke on="EIS Subpanel" class="SubPnl" method="Remove VI"(error in=w677) -> (error out=w676:errorcluster)  [unwired: 2 in, 2 out]
                n270 = call-dynamic "Destroy.vi"("reference in"=w674, "Error In"=w676) -> ("Error Out"=w675:errorcluster)  [unwired: 16 in, 1 out]
              }
              frame True {
              }
            }
            n271 = local read "EIS Parameters"() -> (w655:T9)
            n272 = Unbundle By Name(w655) -> ("EIS Mode"=w654:u16, "EIS DC Potential"=w653:dbl, "EIS Start Frequency"=w652:dbl, "EIS Stop Frequency"=w651:dbl, "EIS Delta Frequency"=w650:dbl, "EIS DC Current"=w649:dbl, "AC Signal (mV/mA RMS)"=w648:dbl, "Cycles at Frequency"=w647:dbl, "EIS AC Step Delay"=w646:dbl)
            n273 = Bundle By Name(cluster=T17 {"EIS Mode"=2, "EIS DC Potential"=650.0, "EIS Start Frequency"=1000.0, "EIS Stop Frequency"=500.0, "EIS Delta Frequency"=100.0, "EIS DC Current"=0.0, "AC Signal (mV/mA RMS)"=20.0, "Cycles at Frequency"=1000.0, "EIS AC Step Delay"=1.0} ("EIS Parameters"), "EIS Mode"=w654, "EIS DC Potential"=w653, "EIS Start Frequency"=w652, "EIS Stop Frequency"=w651, "EIS Delta Frequency"=w650, "EIS DC Current"=w649, "AC Signal (mV/mA RMS)"=w648, "Cycles at Frequency"=w647, "EIS AC Step Delay"=w646) -> (w662:T17)
            n274 = call "ACIR_EIS_Create.vi"("EIS Parameters"=w662, "Logger"=w656, "Error In"=w665) -> ("reference out"=w669:refnum<class "ACIR_EIS.lvclass">, "ProcessViRef"=w671:refnum<vi>, "Error Out"=w672:errorcluster)  [unwired: 10 in]
            n275 = call <userlib>:"Fit VI window to Largest Dec__ogtk.vi"("error in (no error)"=w672, "VI Ref (calling VI)"=w671) -> ("error out"=w661:errorcluster, "dup VI Ref"=w660:refnum<vi>)  [unwired: 4 in]
            n276 = Bundle By Name(cluster=w668, "EIS Ref"=w669) -> (w670:T13)
            n277 = invoke on="EIS Subpanel" class="SubPnl" method="Insert VI"(error in=w661, "VI Ref"=w660) -> (error out=w659:errorcluster)  [unwired: 2 in, 3 out]
            n278 = property on="Toggle EIS Profile" class="Bool (strict)"(error in=w659, "DisabledEnum"=T14."Enabled" ("Disabled")) -> (error out=w658:errorcluster)  [unwired: 1 in, 1 out]
          }
          frame condition #1 {
          }
        }
      }
      frame "EIS: Load EIS Data" {
        (unwired) T14."Enabled" ("Disabled")
        # "#todo\n\nload TDMS file method on EIS class"
      }
      frame "EIS: Generate Report" {
        n279 = disable-structure shown="TARGET_TYPE==Windows, Default" {
          disable-tunnel: w687 -> [w693 _]
          disable-tunnel: w686 -> [w692 w694]
          disable-tunnel: [w690 w694] -> w685
          frame condition #0 (active) {
            n280 = Unbundle By Name(w693) -> ("EIS Ref"=w691:refnum<class "ACIR_EIS.lvclass">)
            n281 = call "Generate Plots.vi"("reference in"=w691, "Error In"=w692) -> ("Error Out"=w690:errorcluster)  [unwired: 16 in, 1 out]
          }
          frame condition #1 {
          }
        }
      }
      frame "---------- POWER MODULE ----------" {
        # "Do not put any code in this frame.\n(It is a separator no-op. You can make a copy of this frame to create a new UI frame)"
        n282 = call <vilib>:"Add State(s) to Queue__jki_lib_state_machine.vi"("State(s) in (\"\")"=w699) -> ("States Out"=w698:string)  [unwired: 14 in]
      }
      frame "PMOD: Connect" {
        # "If we fail to connect the unit,\nthen cancel the remaining steps"
        n283 = Unbundle By Name(w710) -> ("Power Module"=w709:refnum<class "PowerModuleInterface.lvclass">)
        n284 = call-dynamic "Connect.vi"("object in"=w709, "Error In"=w708) -> ("object out"=w705:refnum<class "PowerModuleInterface.lvclass">, "Error Out"=w706:errorcluster)  [unwired: 12 in]
        n285 = call-dynamic "Get Capabilities.vi"("object in"=w705, "Error In"=w706) -> ("object out"=w703:refnum<class "PowerModuleInterface.lvclass">, "Error Out"=w704:errorcluster)  [unwired: 10 in, 2 out]
        n286 = property on="Module Selection" class="Ring (strict)"() -> ("RingText.Text"=w701:string)  [unwired: 2 in, 2 out]
        n287 = Format Into String(format string="VOLTA CONTROL SUITE - %s CONNECTED" ("Front Panel Window:Title"), w701) -> (resulting string=w700:string)  [unwired: 2 in, 1 out]
        n288 = Unbundle By Name(w704) -> ("status"=w719:bool)
        n289 = Not(x=w719) -> (.not. x?=w707:bool)
        n290 = Select(t=w714, s=w707, f="UI: Connection Failed\nUI: Cursor Set >> Idle") -> (s? t:f=w713:string)
        n291 = Select(t=w700, s=w707, f="VOLTA CONTROL SUITE" ("Front Panel Window:Title")) -> (s? t:f=w711:string)
        n292 = Select(t=T14."Enabled" ("Disabled"), s=w707, f=T14."Disabled and Grayed Out" ("Disabled")) -> (s? t:f=w716:T14)
        n293 = local write "PMOD Connect"(w707) -> ()
        n294 = property class="VI"("Front Panel.Title"=w711) -> ()  [unwired: 2 in, 2 out]
        n295 = property on="PMOD Clear" class="Bool"("DisabledEnum"=w716) -> ()  [unwired: 2 in, 2 out]
        n296 = property on="PMOD Reserve" class="Bool (strict)"("DisabledEnum"=w716) -> ()  [unwired: 2 in, 2 out]
        n297 = Bundle By Name(cluster=w710, "Power Module"=w703, "Connected"=w707) -> (w721:T13)
      }
      frame "PMOD: Disconnect" {
        n298 = Unbundle By Name(w736) -> ("Power Module"=w728:refnum<class "PowerModuleInterface.lvclass">)
        n299 = call-dynamic "Disconnect.vi"("object in"=w728, "Error In"=w729) -> ("object out"=w727:refnum<class "PowerModuleInterface.lvclass">, "Error Out"=w726:errorcluster)  [unwired: 12 in]
        n300 = Unbundle By Name(w726) -> ("status"=w725:bool)
        n301 = local write "PMOD Connect"(w725) -> ()
        n302 = Bundle By Name(cluster=w736, "Power Module"=w727, "Connected"=w725) -> (w737:T13)
        n303 = Select(t=T14."Enabled" ("Disabled"), s=w725, f=T14."Disabled and Grayed Out" ("Disabled")) -> (s? t:f=w732:T14)
        n304 = property on="Module Selection" class="Ring (strict)"() -> ("RingText.Text"=w723:string)  [unwired: 2 in, 2 out]
        n305 = property on="PMOD Reserve" class="Bool (strict)"("DisabledEnum"=w732) -> ()  [unwired: 2 in, 2 out]
        n306 = property on="PMOD Clear" class="Bool"("DisabledEnum"=w732) -> ()  [unwired: 2 in, 2 out]
        n307 = Format Into String(format string="VOLTA CONTROL SUITE - %s CONNECTED" ("Front Panel Window:Title"), w723) -> (resulting string=w722:string)  [unwired: 2 in, 1 out]
        n308 = Select(t=w722, s=w725, f="VOLTA CONTROL SUITE" ("Front Panel Window:Title")) -> (s? t:f=w731:string)
        n309 = property class="VI"("Front Panel.Title"=w731) -> ()  [unwired: 2 in, 2 out]
      }
      frame "PMOD: Reserve" {
        w747 = T14."Disabled and Grayed Out" ("Disabled")
        w748 = T14."Enabled" ("Disabled")
        # "If we fail to reserve the unit,\nthen cancel the remaining steps"
        n310 = Unbundle By Name(w758) -> ("Power Module"=w759:refnum<class "PowerModuleInterface.lvclass">, "Reserved"=w754:bool)
        n311 = case shown="False" w754 {
          selector: w754 -> [_ w768]
          tunnel: w760 -> [w767 w769]
          tunnel: w759 -> [w766 w770]
          tunnel: [w765 w770] -> w756
          tunnel: [w764 w769] -> w755
          tunnel: [w762 w768] -> w744
          frame False {
            n312 = call-dynamic "Reserve.vi"("object in"=w766, "Error In"=w767) -> ("object out"=w765:refnum<class "PowerModuleInterface.lvclass">, "Error Out"=w764:errorcluster)  [unwired: 12 in]
            n313 = Unbundle By Name(w764) -> ("status"=w763:bool)
            n314 = Not(x=w763) -> (.not. x?=w762:bool)
          }
          frame True {
          }
        }
        n315 = Select(t=w752, s=w744, f="UI: Reservation Failed\nUI: Cursor Set >> Idle") -> (s? t:f=w750:string)
        n316 = Bundle By Name(cluster=w758, "Power Module"=w756, "Reserved"=w744) -> (w757:T13)
        n317 = local write "PMOD Reserve"(w744) -> ()
        n318 = Select(t=w748, s=w744, f=w747) -> (s? t:f=w745:T14)
        n319 = Select(t=w748, s=w744, f=w747) -> (s? t:f=w746:T14)
        n320 = Select(t=w747, s=w744, f=w748) -> (s? t:f=w753:T14)
        n321 = property on="Module Selection" class="Ring (strict)"() -> ("RingText.Text"=w740:string)  [unwired: 2 in, 2 out]
        n322 = property on="Apply Mode & Range" class="Bool"("DisabledEnum"=w745) -> ()  [unwired: 2 in, 2 out]
        n323 = property on="Apply Limits" class="Bool"("DisabledEnum"=w745) -> ()  [unwired: 2 in, 2 out]
        n324 = property on="Apply Slew Rates" class="Bool"("DisabledEnum"=w745) -> ()  [unwired: 2 in, 2 out]
        n325 = property on="Start Profile" class="Bool (strict)"("DisabledEnum"=w746) -> ()  [unwired: 2 in, 2 out]
        n326 = property on="PMOD Clear" class="Bool"("DisabledEnum"=w753) -> ()  [unwired: 2 in, 2 out]
        n327 = property on="Apply Setpoints" class="Bool"("DisabledEnum"=w745) -> ()  [unwired: 2 in, 2 out]
        n328 = property on="Energize" class="Bool (strict)"("DisabledEnum"=w745) -> ()  [unwired: 2 in, 2 out]
        n329 = property on="Output" class="Bool (strict)"("DisabledEnum"=w745) -> ()  [unwired: 2 in, 2 out]
        n330 = property on="Launch Battery Simulation" class="Bool"("DisabledEnum"=w745) -> ()  [unwired: 2 in, 2 out]
        n331 = property on="Generate HPPC Profile" class="Bool"("DisabledEnum"=w745) -> ()  [unwired: 2 in, 2 out]
        n332 = property on="Generate EIS Profile" class="Bool"("DisabledEnum"=w745) -> ()  [unwired: 2 in, 2 out]
        n333 = Format Into String(format string="VOLTA CONTROL SUITE - %s RESERVED" ("Front Panel Window:Title"), w740) -> (resulting string=w742:string)  [unwired: 2 in, 1 out]
        n334 = Format Into String(format string="VOLTA CONTROL SUITE - %s CONNECTED" ("Front Panel Window:Title"), w740) -> (resulting string=w739:string)  [unwired: 2 in, 1 out]
        n335 = Select(t=w742, s=w744, f=w739) -> (s? t:f=w749:string)
        n336 = property class="VI"("Front Panel.Title"=w749) -> ()  [unwired: 2 in, 2 out]
      }
      frame "PMOD: Unreserve" {
        w784 = T14."Disabled and Grayed Out" ("Disabled")
        w783 = T14."Enabled" ("Disabled")
        n337 = Unbundle By Name(w787) -> ("Power Module"=w781:refnum<class "PowerModuleInterface.lvclass">)
        n338 = call-dynamic "Unreserve.vi"("object in"=w781, "Error In"=w780) -> ("object out"=w779:refnum<class "PowerModuleInterface.lvclass">, "Error Out"=w778:errorcluster)  [unwired: 12 in]
        n339 = Unbundle By Name(w778) -> ("status"=w773:bool)
        n340 = local write "PMOD Reserve"(w773) -> ()
        n341 = Bundle By Name(cluster=w787, "Power Module"=w779, "Reserved"=w773) -> (w786:T13)
        n342 = Select(t=w784, s=w773, f=w783) -> (s? t:f=w785:T14)
        n343 = Select(t=w783, s=w773, f=w784) -> (s? t:f=w782:T14)
        n344 = property on="PMOD Clear" class="Bool"("DisabledEnum"=w785) -> ()  [unwired: 2 in, 2 out]
        n345 = property on="Apply Mode & Range" class="Bool"("DisabledEnum"=w782) -> ()  [unwired: 2 in, 2 out]
        n346 = property on="Apply Limits" class="Bool"("DisabledEnum"=w782) -> ()  [unwired: 2 in, 2 out]
        n347 = property on="Apply Setpoints" class="Bool"("DisabledEnum"=w782) -> ()  [unwired: 2 in, 2 out]
        n348 = property on="Energize" class="Bool (strict)"("DisabledEnum"=w782) -> ()  [unwired: 2 in, 2 out]
        n349 = property on="Output" class="Bool (strict)"("DisabledEnum"=w782) -> ()  [unwired: 2 in, 2 out]
        n350 = property on="Apply Slew Rates" class="Bool"("DisabledEnum"=w782) -> ()  [unwired: 2 in, 2 out]
        n351 = property on="Start Profile" class="Bool (strict)"("DisabledEnum"=w782) -> ()  [unwired: 2 in, 2 out]
        n352 = property on="Module Selection" class="Ring (strict)"() -> ("RingText.Text"=w772:string)  [unwired: 2 in, 2 out]
        n353 = property on="Generate EIS Profile" class="Bool"("DisabledEnum"=w782) -> ()  [unwired: 2 in, 2 out]
        n354 = property on="Launch Battery Simulation" class="Bool"("DisabledEnum"=w782) -> ()  [unwired: 2 in, 2 out]
        n355 = property on="Generate HPPC Profile" class="Bool"("DisabledEnum"=w782) -> ()  [unwired: 2 in, 2 out]
        n356 = Format Into String(format string="VOLTA CONTROL SUITE - %s RESERVED" ("Front Panel Window:Title"), w772) -> (resulting string=w775:string)  [unwired: 2 in, 1 out]
        n357 = Format Into String(format string="VOLTA CONTROL SUITE - %s CONNECTED" ("Front Panel Window:Title"), w772) -> (resulting string=w771:string)  [unwired: 2 in, 1 out]
        n358 = Select(t=w775, s=w773, f=w771) -> (s? t:f=w777:string)
        n359 = property class="VI"("Front Panel.Title"=w777) -> ()  [unwired: 2 in, 2 out]
      }
      frame "PMOD: Clear" {
        n360 = Unbundle By Name(w795) -> ("Power Module"=w793:refnum<class "PowerModuleInterface.lvclass">)
        n361 = call-dynamic "Clear Reservation.vi"("object in"=w793, "Error In"=w792) -> ("object out"=w790:refnum<class "PowerModuleInterface.lvclass">, "Error Out"=w791:errorcluster)  [unwired: 12 in]
        n362 = Bundle By Name(cluster=w795, "Power Module"=w790) -> (w794:T13)
      }
      frame "PMOD: Apply Setpoints" {
        n363 = Unbundle By Name(w806) -> ("Power Module"=w803:refnum<class "PowerModuleInterface.lvclass">, "Connected"=w800:bool, "Reserved"=w799:bool)
        n364 = And(x=w800, y=w799) -> (x .and. y?=w798:bool)
        n365 = case shown="True" w798 {
          tunnel: w801 -> [w809 w820]
          tunnel: [w809 w812] -> w804
          tunnel: w803 -> [w810 w821]
          tunnel: [w810 w811] -> w802
          frame False {
          }
          frame True {
            n366 = local read "Setpoints"() -> (w822:T7)
            n367 = Unbundle By Name(w822) -> ("Voltage"=w815:dbl, "Current"=w813:dbl, "Resistance [Ohms]"=w814:dbl)
            n368 = call-dynamic "Set Resistance.vi"("object in"=w821, "resistance (Ohm)"=w814, "Error In"=w820) -> ("object out"=w818:refnum<class "PowerModuleInterface.lvclass">, "Error Out"=w819:errorcluster)  [unwired: 11 in]
            n369 = call-dynamic "Set Current.vi"("object in"=w818, "current (A)"=w813, "Error In"=w819) -> ("object out"=w817:refnum<class "PowerModuleInterface.lvclass">, "Error Out"=w816:errorcluster)  [unwired: 11 in]
            n370 = call-dynamic "Set Voltage.vi"("object in"=w817, "voltage (V)"=w815, "Error In"=w816) -> ("object out"=w811:refnum<class "PowerModuleInterface.lvclass">, "Error Out"=w812:errorcluster)  [unwired: 11 in]
          }
        }
        n371 = Bundle By Name(cluster=w806, "Power Module"=w802) -> (w805:T13)
      }
      frame "PMOD: Set Mode and Range" {
        n372 = Unbundle By Name(w831) -> ("Power Module"=w827:refnum<class "PowerModuleInterface.lvclass">, "Connected"=w825:bool, "Reserved"=w824:bool)
        n373 = And(x=w825, y=w824) -> (x .and. y?=w823:bool)
        n374 = case shown="True" w823 {
          tunnel: w829 -> [w835 w854]
          tunnel: [w835 w851] -> w828
          tunnel: w827 -> [w836 w848]
          tunnel: [w836 w852] -> w826
          frame False {
          }
          frame True {
            w861 = refnum<vi> refnum  # Ring
            n375 = property on="Mode & Range" class="Clust (strict)"() -> ("Controls[]"=w855:refnum<vi>[])  [unwired: 2 in, 2 out]
            n376 = Index Array(array=w855) -> (element #1=w863:refnum<vi>, element #2=w862:refnum<vi>)  [unwired: 2 in]
            n377 = To More Specific Class(target class=w861, reference=w863, error in=w854) -> (specific class reference=w859:refnum<vi>, error out=w860:errorcluster)
            n378 = To More Specific Class(target class=w861, reference=w862, error in=w854) -> (specific class reference=w857:refnum<vi>, error out=w858:errorcluster)
            n379 = property class="Ring"(reference=w859, error in=w860) -> (error out=w856:errorcluster, "RingText.Text"=w853:string)  [unwired: 1 out]
            n380 = property class="Ring"(reference=w857, error in=w858) -> (error out=w843:errorcluster, "RingText.Text"=w845:string)  [unwired: 1 out]
            n381 = Scan From String(format string="%f,%f V / %f,%f A", input string=w845, error in=w843) -> (error out=w842:errorcluster, output 1=w841:dbl, output 2=w840:dbl, output 3=w839:dbl, output 4=w838:dbl)  [unwired: 5 in, 2 out]
            n382 = Merge Errors(w856, w842) -> (w847:errorcluster)
            n383 = Bundle By Name(cluster=T19 {"Current Max (A)"=0.0, "Current Min (A)"=0.0, "Voltage Max (V)"=0.0, "Voltage Min (V)"=0.0} ("Range"), "Voltage Min (V)"=w841, "Voltage Max (V)"=w840, "Current Min (A)"=w839, "Current Max (A)"=w838) -> (w837:T19)
            n384 = call-dynamic "Set Range.vi"("object in"=w848, "Range"=w837, "Error In"=w847) -> ("object out"=w849:refnum<class "PowerModuleInterface.lvclass">, "Error Out"=w850:errorcluster)  [unwired: 11 in]
            n385 = call-dynamic "Set Mode.vi"("object in"=w849, "mode"=w853, "Error In"=w850) -> ("object out"=w852:refnum<class "PowerModuleInterface.lvclass">, "Error Out"=w851:errorcluster)  [unwired: 11 in]
          }
        }
        n386 = Bundle By Name(cluster=w831, "Power Module"=w826) -> (w830:T13)
        n387 = call <vilib>:"Add State(s) to Queue__jki_lib_state_machine.vi"("State(s) in (\"\")"=w834) -> ("States Out"=w833:string)  [unwired: 14 in]
      }
      frame "PMOD: Get Mode and Range" {
        n388 = Unbundle By Name(w872) -> ("Power Module"=w868:refnum<class "PowerModuleInterface.lvclass">, "Connected"=w866:bool, "Reserved"=w865:bool)
        n389 = And(x=w866, y=w865) -> (x .and. y?=w864:bool)
        n390 = case shown="True" w864 {
          tunnel: w870 -> [w876 w886]
          tunnel: [w876 w879] -> w869
          tunnel: w868 -> [w877 w885]
          tunnel: [w877 w881] -> w867
          frame False {
          }
          frame True {
            n391 = call-dynamic "Get Range.vi"("object in"=w885, "Error In"=w886) -> ("object out"=w883:refnum<class "PowerModuleInterface.lvclass">, "Range"=w880:T19, "Error Out"=w882:errorcluster)  [unwired: 11 in]
            n392 = call-dynamic "Get Mode.vi"("object in"=w883, "Error In"=w882) -> ("object out"=w881:refnum<class "PowerModuleInterface.lvclass">, "mode"=w878:string, "Error Out"=w884:errorcluster)  [unwired: 11 in]
            n393 = disable-structure shown="Disabled" {
              disable-tunnel: w884 -> [w897 _]
              disable-tunnel: w880 -> [w896 _]
              disable-tunnel: [w888 _] -> w879
              disable-tunnel: w878 -> [w887 _]
              frame Disabled {
                w904 = refnum<vi> refnum  # Ring
                n394 = Unbundle By Name(w896) -> ("Voltage Min (V)"=w894:dbl, "Voltage Max (V)"=w893:dbl, "Current Min (A)"=w892:dbl, "Current Max (A)"=w891:dbl)
                n395 = local write "MODE"(w887) -> ()
                n396 = property on="Mode & Range" class="Clust (strict)"() -> ("Controls[]"=w898:refnum<vi>[])  [unwired: 2 in, 2 out]
                n397 = Format Into String(format string="%.0f,%.0f V / %.0f,%.0f A", w894, w893, w892, w891) -> (resulting string=w890:string)  [unwired: 2 in, 1 out]
                n398 = Index Array(array=w898) -> (element #1=w906:refnum<vi>, element #2=w905:refnum<vi>)  [unwired: 2 in]
                n399 = To More Specific Class(target class=w904, reference=w906, error in=w897) -> (specific class reference=w902:refnum<vi>, error out=w903:errorcluster)
                n400 = To More Specific Class(target class=w904, reference=w905, error in=w897) -> (specific class reference=w900:refnum<vi>, error out=w901:errorcluster)
                n401 = property class="Ring"(reference=w902, error in=w903, "RingText.Text"=w887) -> (error out=w899:errorcluster)  [unwired: 1 out]
                n402 = property class="Ring"(reference=w900, error in=w901, "RingText.Text"=w890) -> (error out=w889:errorcluster)  [unwired: 1 out]
                n403 = Merge Errors(w899, w889) -> (w888:errorcluster)
              }
              frame Enabled {
              }
            }
          }
        }
        n404 = Bundle By Name(cluster=w872, "Power Module"=w867) -> (w871:T13)
        n405 = call <vilib>:"Add State(s) to Queue__jki_lib_state_machine.vi"("State(s) in (\"\")"=w875) -> ("States Out"=w874:string)  [unwired: 14 in]
      }
      frame "PMOD: Set Limits" {
        n406 = Unbundle By Name(w916) -> ("Power Module"=w912:refnum<class "PowerModuleInterface.lvclass">, "Connected"=w909:bool, "Reserved"=w910:bool)
        n407 = And(x=w909, y=w910) -> (x .and. y?=w908:bool)
        n408 = case shown="True" w908 {
          tunnel: w914 -> [w921 w926]
          tunnel: [w921 w925] -> w913
          tunnel: w912 -> [w920 w923]
          tunnel: [w920 w924] -> w911
          tunnel: "Limits" -> [_ w922]
          frame False {
          }
          frame True {
            # "#coercion"
            n409 = call-dynamic "Set Limits.vi"("object in"=w923, "limits"=w922, "Error In"=w926) -> ("object out"=w924:refnum<class "PowerModuleInterface.lvclass">, "Error Out"=w925:errorcluster)  [unwired: 11 in]
          }
        }
        n410 = Bundle By Name(cluster=w916, "Power Module"=w911) -> (w915:T13)
        n411 = call <vilib>:"Add State(s) to Queue__jki_lib_state_machine.vi"("State(s) in (\"\")"=w919) -> ("States Out"=w918:string)  [unwired: 14 in]
      }
      frame "PMOD: Get Limits" {
        n412 = Unbundle By Name(w930) -> ("Power Module"=w929:refnum<class "PowerModuleInterface.lvclass">, "Connected"=w927:bool)
        n413 = Format Into String(format string="%s: Read Setpoint Limits", w932) -> (resulting string=w934:string)  [unwired: 2 in, 1 out]
        n414 = local write "Status Message"(w934) -> ()
        n415 = case shown="True" w927 {
          tunnel: w931 -> [w937 w941]
          tunnel: w929 -> [_ w940]
          tunnel: [w937 w939] -> w928
          frame False {
          }
          frame True {
            # "#coercion"
            n416 = call-dynamic "Get Limits.vi"("object in"=w940, "Error In"=w941) -> ("Limits"=w938:T24, "Error Out"=w939:errorcluster)  [unwired: 11 in, 1 out]
            n417 = local write "Limits"(w938) -> ()
          }
        }
      }
      frame "PMOD: Energize" {
        n418 = Unbundle By Name(w948) -> ("Power Module"=w944:refnum<class "PowerModuleInterface.lvclass">, "Connected"=w943:bool)
        n419 = case shown="True" w943 {
          tunnel: w946 -> [w951 w957]
          tunnel: [w951 w953] -> w945
          tunnel: w944 -> [w952 w955]
          tunnel: [w952 w954] -> w942
          frame False {
          }
          frame True {
            n420 = call-dynamic "Set Energize Enable.vi"("object in"=w955, "energize"="Energize", "Error In"=w957) -> ("object out"=w954:refnum<class "PowerModuleInterface.lvclass">, "Error Out"=w953:errorcluster)  [unwired: 11 in]
          }
        }
        n421 = Bundle By Name(cluster=w948, "Power Module"=w942) -> (w947:T13)
      }
      frame "PMOD: Output" {
        n422 = Unbundle By Name(w964) -> ("Power Module"=w960:refnum<class "PowerModuleInterface.lvclass">, "Connected"=w959:bool)
        n423 = case shown="True" w959 {
          tunnel: w962 -> [w967 w973]
          tunnel: [w967 w972] -> w961
          tunnel: w960 -> [w968 w971]
          tunnel: [w968 w970] -> w958
          frame False {
          }
          frame True {
            n424 = call-dynamic "Set Output Enable.vi"("object in"=w971, "output"="Output", "Error In"=w973) -> ("object out"=w970:refnum<class "PowerModuleInterface.lvclass">, "Error Out"=w972:errorcluster)  [unwired: 11 in]
          }
        }
        n425 = Bundle By Name(cluster=w964, "Power Module"=w958) -> (w963:T13)
      }
      frame "PMOD: Start Setpoint Stream" {
        n426 = Unbundle By Name(w981) -> ("Power Module"=w984:refnum<class "PowerModuleInterface.lvclass">, "Connected"=w983:bool, "Reserved"=w976:bool)
        n427 = Format Into String(format string="%s: Starting Setpoint Stream", w977) -> (resulting string=w979:string)  [unwired: 2 in, 1 out]
        n428 = local write "Status Message"(w979) -> ()
        n429 = And(x=w983, y=w976) -> (x .and. y?=w982:bool)
        n430 = case shown="True" w982 {
          tunnel: w986 -> [w990 w995]
          tunnel: [w990 w994] -> w985
          tunnel: w984 -> [w991 w997]
          tunnel: [w991 w996] -> w975
          tunnel: [FALSE w992] -> w974
          frame False {
          }
          frame True {
            n431 = call-dynamic "Start Profile.vi"("object in"=w997, "Error In"=w995) -> ("object out"=w996:refnum<class "PowerModuleInterface.lvclass">, "Error Out"=w994:errorcluster)  [unwired: 12 in]
            n432 = Unbundle By Name(w994) -> ("status"=w993:bool)
            n433 = Not(x=w993) -> (.not. x?=w992:bool)
          }
        }
        n434 = local write "Start Profile"(w974) -> ()
        n435 = Bundle By Name(cluster=w981, "Power Module"=w975) -> (w987:T13)
      }
      frame "PMOD: Update Setpoint Stream" {
        n436 = Unbundle By Name(w1005) -> ("Power Module"=w1001:refnum<class "PowerModuleInterface.lvclass">, "Loaded Profile"=w999:dbl[][], "Connected"=w1000:bool)
        n437 = case shown="True" w1000 {
          tunnel: w1003 -> [w1008 w1012]
          tunnel: [w1008 w1015] -> w1002
          tunnel: w1001 -> [w1009 w1013]
          tunnel: [w1009 w1014] -> w998
          tunnel: w999 -> [_ w1010]
          frame False {
          }
          frame True {
            n438 = call-dynamic "Load Profile.vi"("object in"=w1013, "profile"=w1010, "step dt"="Profile Step dT (ns)", "Error In"=w1012) -> ("object out"=w1014:refnum<class "PowerModuleInterface.lvclass">, "Error Out"=w1015:errorcluster)  [unwired: 10 in]
          }
        }
        n439 = Bundle By Name(cluster=w1005, "Power Module"=w998) -> (w1004:T13)
      }
      frame "PMOD: Stop Setpoint Stream" {
        n440 = Unbundle By Name(w1019) -> ("Power Module"=w1022:refnum<class "PowerModuleInterface.lvclass">, "Connected"=w1021:bool, "Reserved"=w1016:bool)
        n441 = And(x=w1021, y=w1016) -> (x .and. y?=w1020:bool)
        n442 = case shown="True" w1020 {
          tunnel: w1024 -> [w1029 w1034]
          tunnel: [w1029 w1031] -> w1023
          tunnel: w1022 -> [w1030 w1033]
          tunnel: [w1030 w1032] -> w1017
          tunnel: [w1028 w1035] -> w1018
          frame False {
            n443 = local read "Start Profile"() -> (w1028:bool)
          }
          frame True {
            n444 = call-dynamic "Stop Profile.vi"("object in"=w1033, "Error In"=w1034) -> ("object out"=w1032:refnum<class "PowerModuleInterface.lvclass">, "Error Out"=w1031:errorcluster)  [unwired: 12 in]
            n445 = Unbundle By Name(w1031) -> ("status"=w1035:bool)
          }
        }
        n446 = local write "Start Profile"(w1018) -> ()
        n447 = Bundle By Name(cluster=w1019, "Power Module"=w1017) -> (w1025:T13)
      }
      frame "PMOD: Write Slew Rates" {
        n448 = Unbundle By Name(w1052) -> ("Power Module"=w1049:refnum<class "PowerModuleInterface.lvclass">)
        n449 = local read "Slew Rates"() -> (w1036:T5)
        n450 = Format Into String(format string="%s: Write Slew Rates", w1055) -> (resulting string=w1057:string)  [unwired: 2 in, 1 out]
        n451 = local write "Status Message"(w1057) -> ()
        n452 = Unbundle By Name(w1036) -> ("Current Dec. [A/sec]"=w1048:sgl, "Current Inc. [A/sec]"=w1046:sgl, "Voltage Dec. [V/sec]"=w1044:sgl, "Voltage Inc. [V/sec]"=w1042:sgl, "Resistance Dec. [Ohms/sec]"=w1040:sgl, "Resistance Inc. [Ohms/sec]"=w1037:sgl)
        n453 = To Double Precision Float(number=w1048) -> (double precision float=w1047:dbl)
        n454 = To Double Precision Float(number=w1046) -> (double precision float=w1045:dbl)
        n455 = To Double Precision Float(number=w1044) -> (double precision float=w1043:dbl)
        n456 = To Double Precision Float(number=w1042) -> (double precision float=w1041:dbl)
        n457 = To Double Precision Float(number=w1040) -> (double precision float=w1039:dbl)
        n458 = To Double Precision Float(number=w1037) -> (double precision float=w1038:dbl)
        n459 = Bundle By Name(cluster=T20 {"Current Decrease (A/sec)"=0.0, "Current Increase (A/sec)"=0.0, "Voltage Decrease (V/sec)"=0.0, "Voltage Increase (V/sec)"=0.0, "Resistance Decrease (Ohm/sec)"=0.0, "Resistance Increase (Ohm/sec)"=0.0} ("Slew Rates"), "Current Decrease (A/sec)"=w1047, "Current Increase (A/sec)"=w1045, "Voltage Decrease (V/sec)"=w1043, "Voltage Increase (V/sec)"=w1041, "Resistance Decrease (Ohm/sec)"=w1039, "Resistance Increase (Ohm/sec)"=w1038) -> (w1050:T20)
        n460 = call-dynamic "Set Slew Rates.vi"("object in"=w1049, "Slew Rates"=w1050, "Error In"=w1054) -> ("Error Out"=w1053:errorcluster)  [unwired: 11 in, 1 out]
      }
      frame "PMOD: Read Slew Rates" {
        n461 = Unbundle By Name(w1078) -> ("Power Module"=w1077:refnum<class "PowerModuleInterface.lvclass">)
        n462 = Format Into String(format string="%s: Read Slew Rates", w1079) -> (resulting string=w1081:string)  [unwired: 2 in, 1 out]
        n463 = local write "Status Message"(w1081) -> ()
        n464 = call-dynamic "Get Slew Rates.vi"("object in"=w1077, "Error In"=w1076) -> ("Slew Rates"=w1072:T20, "Error Out"=w1075:errorcluster)  [unwired: 11 in, 1 out]
        n465 = Unbundle By Name(w1072) -> ("Voltage Increase (V/sec)"=w1071:dbl, "Voltage Decrease (V/sec)"=w1069:dbl, "Current Increase (A/sec)"=w1067:dbl, "Current Decrease (A/sec)"=w1065:dbl, "Resistance Increase (Ohm/sec)"=w1063:dbl, "Resistance Decrease (Ohm/sec)"=w1061:dbl)
        n466 = To Single Precision Float(number=w1071) -> (single precision float=w1070:sgl)
        n467 = To Single Precision Float(number=w1069) -> (single precision float=w1068:sgl)
        n468 = To Single Precision Float(number=w1067) -> (single precision float=w1066:sgl)
        n469 = To Single Precision Float(number=w1065) -> (single precision float=w1064:sgl)
        n470 = To Single Precision Float(number=w1063) -> (single precision float=w1062:sgl)
        n471 = To Single Precision Float(number=w1061) -> (single precision float=w1060:sgl)
        n472 = Bundle By Name(cluster=T5 {"Voltage Inc. [V/sec]"=inf, "Voltage Dec. [V/sec]"=inf, "Current Inc. [A/sec]"=inf, "Current Dec. [A/sec]"=inf, "Resistance Inc. [Ohms/sec]"=inf, "Resistance Dec. [Ohms/sec]"=inf} ("Slew Rates"), "Voltage Inc. [V/sec]"=w1070, "Voltage Dec. [V/sec]"=w1068, "Current Inc. [A/sec]"=w1066, "Current Dec. [A/sec]"=w1064, "Resistance Inc. [Ohms/sec]"=w1062, "Resistance Dec. [Ohms/sec]"=w1060) -> (w1073:T5)
        n473 = local write "Slew Rates"(w1073) -> ()
      }
      frame "---------- Profile ----------" {
        # "Do not put any code in this frame.\n(It is a separator no-op. You can make a copy of this frame to create a new UI frame)"
      }
      frame "Profile: Load" {
        n474 = call-poly <vilib>:"Read Delimited Spreadsheet.vi"("file path (dialog if empty)"="CSV Profile Path", "error in (no error)"=w1095, "delimiter (\\t)"="," ("delimiter (\\t)")) -> ("all rows"=w1090:dbl[][], "error out"=w1092:errorcluster)  [unwired: 7 in, 4 out]
        n475 = case shown="No Error" w1092 {
          selector: w1092 -> [w1130 w1139]
          tunnel: [w1130 w1139] -> w1091
          tunnel: w1090 -> [w1115 _]
          tunnel: w1088 -> [w1128 w1138]
          tunnel: [w1127 w1138] -> w1089
          tunnel: w1088 -> [w1102 _]
          frame No Error {
            w1100 = 1500  # max profile steps
            # "#todo\n\nwarning about decimated profile resolution for profiles larger than 1500 steps"
            # "remove header\nrow"
            n476 = Unbundle By Name(w1102) -> ("Reserved"=w1101:bool)
            n477 = Delete From Array(array=w1115, index (row)=0) -> (array with subset deleted=w1109:dbl[][])  [unwired: 2 in, 1 out]
            n478 = local read "Profile Step dT (ns)"() -> (w1124:i64)
            n479 = Array Size(array=w1109) -> (size(s)=w1117:i32[])
            n480 = Index Array(array=w1117, index=0) -> (element=w1110:i32)
            n481 = Divide(x=w1110, y=w1100) -> (x/y=w1113:dbl)
            n482 = Less Or Equal?(x=w1110, y=w1100) -> (x <= y?=w1114:bool)
            n483 = Divide(x=w1124, y=i64 1000000000) -> (x/y=w1121:dbl)
            n484 = Index Array(array=w1109, index (col) #1=0 ("disabled index (col)"), index (col) #2=1 ("index (col)")) -> (element #1=w1118:dbl[], element #2=w1120:dbl[])  [unwired: 2 in]
            n485 = Round Toward +Infinity(x=w1113) -> (ceil(x): smallest int >= x=w1112:dbl)
            n486 = Select(t=T14."Enabled" ("Disabled"), s=w1101, f=T14."Disabled and Grayed Out" ("Disabled")) -> (s? t:f=w1103:T14)
            n487 = Bundle By Name(cluster=waveform(dbl) {"t0"=timestamp(0 s since 1904-01-01), "dt"=1.0, "Y"=[]} ("waveform"), "dt"=w1121) -> (w1107:waveform(dbl))
            n488 = To Long Integer(number=w1112) -> (32bit integer=w1111:i32)
            n489 = Bundle By Name(cluster=w1107, "Y"=w1118) -> (w1119:waveform(dbl))
            n490 = Bundle By Name(cluster=w1107, "Y"=w1120) -> (w1108:waveform(dbl))
            n491 = for {
              tunnel: w1115 -> [w1134] mode=indexing
              workers-P: _ -> [_]
              tunnel: [w1134] -> w1099 mode=indexing if=w1131
              tunnel: w1111 -> [w1136]
              tunnel: w1114 -> [w1132]
              i -> [w1137]
              n492 = Quotient & Remainder(x=w1137, y=w1136) -> (x-y*floor(x/y)=w1135:i32)  [unwired: 1 out]
              n493 = Equal To 0?(x=w1135) -> (x = 0?=w1133:bool)
              n494 = And(x=w1133, y=w1132) -> (x .and. y?=w1131:bool)
            }
            n495 = property on="Start Profile" class="Bool (strict)"("DisabledEnum"=w1103) -> ()  [unwired: 2 in, 2 out]
            n496 = Build Array(w1119, w1108) -> (→"CSV Profile":waveform(dbl)[])
            n497 = local write "Main Tab Control"(Tabs."PROFILE" ("Main Tab Control")) -> ()
            n498 = Bundle By Name(cluster=w1128, "Loaded Profile"=w1099) -> (w1127:T13)
          }
          frame Error {
          }
        }
      }
      frame "Profile: Unload" {
        n499 = Bundle By Name(cluster=w1143, "Loaded Profile"=dbl[][] []) -> (w1142:T13)
      }
      frame "---------- Scripts ----------" {
        # "Do not put any code in this frame.\n(It is a separator no-op. You can make a copy of this frame to create a new UI frame)"
      }
      frame "Script: Launch Logger" {
        n500 = Unbundle By Name(w1155) -> ("Power Module"=w1150:refnum<class "PowerModuleInterface.lvclass">, "Logger Ref"=w1151:refnum<class "Logger.lvclass">)
        n501 = Equal?(x=w1151, y=refnum<class "Logger.lvclass"> refnum) -> (x = y?=w1153:bool)
        n502 = case shown="True" w1153 {
          tunnel: [w1160 w1164] -> w1156
          tunnel: w1157 -> [w1160 w1168]
          tunnel: w1155 -> [w1161 w1170]
          tunnel: [w1161 w1169] -> w1154
          tunnel: w1150 -> [_ w1162]
          frame False {
          }
          frame True {
            n503 = call "Logger_Create.vi"("Output Directory"="Log File Directory", "Power Module"=w1162, "Error In"=w1168, "Log File Type"=enum16{"TDMS", "CSV"}."TDMS") -> ("reference out"=w1165:refnum<class "Logger.lvclass">, "Error Out"=w1164:errorcluster)  [unwired: 14 in]
            n504 = property on="Start Logging" class="Bool (strict)"("DisabledEnum"=T14."Enabled" ("Disabled")) -> ()  [unwired: 2 in, 2 out]
            n505 = Bundle By Name(cluster=w1170, "Logger Ref"=w1165) -> (w1169:T13)
          }
        }
      }
      frame "Script: Start Logger" {
        n506 = Unbundle By Name(w1176) -> ("Logger Ref"=w1172:refnum<class "Logger.lvclass">)
        n507 = Equal?(x=w1172, y=refnum<class "Logger.lvclass"> refnum) -> (x = y?=w1174:bool)
        n508 = case shown="False" w1174 {
          tunnel: [w1190 w1194] -> w1177
          tunnel: w1178 -> [w1186 w1194]
          tunnel: w1176 -> [w1193 w1195]
          tunnel: [w1192 w1195] -> w1175
          tunnel: w1172 -> [w1187 _]
          tunnel: w1171 -> [w1183 _]
          frame False {
            n509 = call "Create Log.vi"("reference in"=w1187, "Error In"=w1186) -> ("reference out"=w1189:refnum<class "Logger.lvclass">, "created file"=w1182:path, "Error Out"=w1191:errorcluster)  [unwired: 15 in]
            n510 = Path To String(path=w1182) -> (string=w1181:string)
            n511 = Format Into String(format string="%s:  Log file created at - %s", w1183, w1181) -> (resulting string=w1185:string)  [unwired: 2 in, 1 out]
            n512 = call "Start Log.vi"("reference in"=w1189, "Error In"=w1191) -> ("reference out"=w1188:refnum<class "Logger.lvclass">, "Error Out"=w1190:errorcluster)  [unwired: 16 in]
            n513 = local write "Status Message"(w1185) -> ()
            n514 = Bundle By Name(cluster=w1193, "Logger Ref"=w1188) -> (w1192:T13)
          }
          frame True {
          }
        }
      }
      frame "Script: Destroy Logger" {
        n515 = Unbundle By Name(w1200) -> ("Logger Ref"=w1196:refnum<class "Logger.lvclass">)
        n516 = Equal?(x=w1196, y=refnum<class "Logger.lvclass"> refnum) -> (x = y?=w1198:bool)
        n517 = case shown="False" w1198 {
          tunnel: [w1207 w1212] -> w1201
          tunnel: w1202 -> [w1209 w1212]
          tunnel: w1200 -> [w1211 w1213]
          tunnel: [w1210 w1213] -> w1199
          tunnel: w1196 -> [w1208 _]
          frame False {
            n518 = call-dynamic "Destroy.vi"("reference in"=w1208, "Error In"=w1209) -> ("Error Out"=w1207:errorcluster)  [unwired: 16 in, 1 out]
            n519 = property on="Start Logging" class="Bool (strict)"("DisabledEnum"=T14."Disabled and Grayed Out" ("Disabled")) -> ()  [unwired: 2 in, 2 out]
            n520 = Bundle By Name(cluster=w1211, "Logger Ref"=refnum<class "Logger.lvclass"> refnum) -> (w1210:T13)
          }
          frame True {
          }
        }
      }
      frame "Script: Launch Grapher" {
        n521 = Unbundle By Name(w1219) -> ("Power Module"=w1215:refnum<class "PowerModuleInterface.lvclass">, "Grapher Ref"=w1217:refnum<class "Grapher.lvclass">)
        n522 = Equal?(x=w1217, y=refnum<class "Grapher.lvclass"> refnum) -> (x = y?=w1216:bool)
        n523 = case shown="True" w1216 {
          tunnel: [w1224 w1228] -> w1220
          tunnel: w1221 -> [w1224 w1241]
          tunnel: w1219 -> [w1225 w1243]
          tunnel: [w1225 w1242] -> w1218
          tunnel: w1215 -> [_ w1232]
          frame False {
          }
          frame True {
            w1240 = 50  # Update Rate (ms)
            n524 = control-ref of="Mini Chart"() -> (w1231:refnum<vi>)
            n525 = control-ref of="XY Graph"() -> (w1238:refnum<vi>)
            n526 = control-ref of="Charging"() -> (w1235:refnum<vi>)
            n527 = control-ref of="Discharging"() -> (w1234:refnum<vi>)
            n528 = control-ref of="Charge Counter"() -> (w1226:refnum<vi>)
            n529 = control-ref of="Function"() -> (w1233:refnum<vi>)
            n530 = control-ref of="VOLTAGE"() -> (w1230:refnum<vi>)
            n531 = control-ref of="CURRENT"() -> (w1229:refnum<vi>)
            n532 = control-ref of="POWER"() -> (w1237:refnum<vi>)
            n533 = Bundle By Name(cluster=T21 {"XY Graph"=refnum, "Mini Chart"=refnum, "Voltage"=refnum, "Current"=refnum, "Power"=refnum, "Function"=refnum, "Charging"=refnum, "Discharging"=refnum, "Charge Counter"=refnum} ("Indicator Refs"), "Mini Chart"=w1231, "XY Graph"=w1238, "Voltage"=w1230, "Current"=w1229, "Power"=w1237, "Function"=w1233, "Charging"=w1235, "Discharging"=w1234, "Charge Counter"=w1226) -> (w1236:T21)
            n534 = call "Grapher_Create.vi"("Indicator Refs"=w1236, "Update Rate (ms)"=w1240, "Power Module"=w1232, "Error In"=w1241) -> ("reference out"=w1227:refnum<class "Grapher.lvclass">, "Error Out"=w1228:errorcluster)  [unwired: 14 in]
            n535 = Bundle By Name(cluster=w1243, "Grapher Ref"=w1227) -> (w1242:T13)
          }
        }
      }
      frame "Script: Launch Battery" {
        n536 = disable-structure shown="TARGET_TYPE==Windows, Default" {
          disable-tunnel: [w1257 w1284] -> w1247
          disable-tunnel: w1246 -> [w1256 w1285]
          disable-tunnel: [w1255 w1285] -> w1245
          disable-tunnel: w1244 -> [w1250 w1284]
          frame condition #0 (active) {
            n537 = Unbundle By Name(w1256) -> ("Power Module"=w1251:refnum<class "PowerModuleInterface.lvclass">, "Battery Ref"=w1253:refnum<class "Battery.lvclass">)
            n538 = Equal?(x=w1253, y=refnum<class "Battery.lvclass"> refnum) -> (x = y?=w1252:bool)
            n539 = case shown="True" w1252 {
              tunnel: [w1258 w1261] -> w1257
              tunnel: w1250 -> [w1258 w1281]
              tunnel: w1256 -> [w1259 w1283]
              tunnel: [w1259 w1282] -> w1255
              tunnel: w1251 -> [_ w1267]
              frame False {
              }
              frame True {
                # "#todo\n\npath for python\nneeds to work properly for development and runtime engine"
                n540 = call "Battery_Create.vi"("Python venv"=path "C:/Repo/volta-control-suite/venv", "Python module"=path "C:/Repo/volta-control-suite/src/Python/hps17k-pybamm-wrapper.py", "Power Module"=w1267, "Error In"=w1281, "# Cells in Series"="Battery Cells in Series", "# Cells in Parallel"="Battery Cells in Parallel") -> ("reference out"=w1263:refnum<class "Battery.lvclass">, "ProcessViRef"=w1276:refnum<vi>, "Error Out"=w1277:errorcluster)  [unwired: 11 in]
                n541 = call <userlib>:"Fit VI window to Largest Dec__ogtk.vi"("error in (no error)"=w1277, "border spacing (2 px)"=0, "VI Ref (calling VI)"=w1276) -> ("error out"=w1274:errorcluster, "dup VI Ref"=w1275:refnum<vi>)  [unwired: 3 in]
                n542 = invoke on="Battery Subpanel" class="SubPnl" method="Insert VI"(error in=w1274, "VI Ref"=w1275) -> (error out=w1262:errorcluster)  [unwired: 2 in, 3 out]
                n543 = call-dynamic "Get SOC OCV Curve.vi"("reference in"=w1263, "Error In"=w1262) -> ("reference out"=w1265:refnum<class "Battery.lvclass">, "Error Out"=w1264:errorcluster)  [unwired: 15 in, 1 out]
                n544 = call-dynamic "Load Simulation.vi"("reference in"=w1265, "Simulation Parameters"="Battery Simulation Parameters", "Error In"=w1264) -> ("reference out"=w1260:refnum<class "Battery.lvclass">, "Error Out"=w1261:errorcluster)  [unwired: 14 in, 1 out]
                n545 = Unbundle By Name(w1261) -> ("status"=w1270:bool)
                n546 = Select(t=T14."Disabled and Grayed Out" ("Disabled"), s=w1270, f=T14."Enabled" ("Disabled")) -> (s? t:f=w1266:T14)
                n547 = Bundle By Name(cluster=w1283, "Battery Ref"=w1260) -> (w1282:T13)
                n548 = property on="Reset Battery Simulation" class="Bool"("DisabledEnum"=w1266) -> ()  [unwired: 2 in, 2 out]
                n549 = property on="Enable Battery Simulation" class="Bool (strict)"("DisabledEnum"=w1266) -> ()  [unwired: 2 in, 2 out]
              }
            }
          }
          frame condition #1 {
          }
        }
      }
      frame "Script: Stop Logger" {
        n550 = Unbundle By Name(w1286) -> ("Logger Ref"=w1289:refnum<class "Logger.lvclass">)
        n551 = Equal?(x=w1289, y=refnum<class "Logger.lvclass"> refnum) -> (x = y?=w1290:bool)
        n552 = case shown="False" w1290 {
          tunnel: w1292 -> [w1300 w1306]
          tunnel: [w1304 w1306] -> w1291
          tunnel: w1289 -> [w1301 _]
          tunnel: w1287 -> [w1302 _]
          frame False {
            w1305 = -1  # timeout in ms (-1)
            n553 = call "Stop Log.vi"("reference in"=w1301, "Error In"=w1300) -> ("reference out"=w1298:refnum<class "Logger.lvclass">, "Error Out"=w1299:errorcluster)  [unwired: 16 in]
            n554 = call "Close Log.vi"("reference in"=w1298, "timeout in ms (-1)"=w1305, "Error In"=w1299) -> ("log file path"=w1303:path, "Error Out"=w1295:errorcluster)  [unwired: 14 in, 1 out]
            n555 = Format Into String(format string="%s: Log File Saved to %s", w1302, w1303) -> (resulting string=w1296:string)  [unwired: 2 in, 1 out]
            n556 = property on="Status Message" class="Str"(error in=w1295, "Value"=w1296) -> (error out=w1304:errorcluster)  [unwired: 1 in, 1 out]
          }
          frame True {
          }
        }
      }
      frame "Script: Stop Battery" {
        n557 = disable-structure shown="TARGET_TYPE==Windows, Default" {
          disable-tunnel: w1310 -> [w1320 w1332]
          disable-tunnel: [w1319 w1332] -> w1309
          disable-tunnel: w1308 -> [w1316 _]
          disable-tunnel: w1308 -> [w1314 _]
          disable-tunnel: [w1313 _] -> w1307
          frame condition #0 (active) {
            n558 = Unbundle By Name(w1316) -> ("Battery Ref"=w1317:refnum<class "Battery.lvclass">)
            n559 = Equal?(x=w1317, y=refnum<class "Battery.lvclass"> refnum ("Battery Ref")) -> (x = y?=w1318:bool)
            n560 = case shown="True" w1318 {
              tunnel: w1320 -> [w1327 w1331]
              tunnel: [w1328 w1331] -> w1319
              tunnel: w1317 -> [w1329 _]
              tunnel: w1314 -> [w1324 w1330]
              tunnel: [w1323 w1330] -> w1313
              frame False {
                w1325 = T14."Disabled and Grayed Out" ("Disabled")
                n561 = invoke on="Battery Subpanel" class="SubPnl" method="Remove VI"(error in=w1327) -> (error out=w1326:errorcluster)  [unwired: 2 in, 2 out]
                n562 = call-dynamic "Battery_Destroy.vi"("reference in"=w1329, "Error In"=w1326) -> ("Error Out"=w1328:errorcluster)  [unwired: 16 in, 1 out]
                n563 = property on="Reset Battery Simulation" class="Bool"("DisabledEnum"=w1325) -> ()  [unwired: 2 in, 2 out]
                n564 = property on="Enable Battery Simulation" class="Bool (strict)"("DisabledEnum"=w1325, "Value"=FALSE ("Enable Battery Simulation")) -> ()  [unwired: 2 in, 2 out]
                n565 = Bundle By Name(cluster=w1324, "Battery Ref"=refnum<class "Battery.lvclass"> refnum) -> (w1323:T13)
              }
              frame True {
              }
            }
          }
          frame condition #1 {
          }
        }
      }
      frame "Script: Stop Grapher" {
        n566 = Unbundle By Name(w1337) -> ("Grapher Ref"=w1335:refnum<class "Grapher.lvclass">)
        n567 = Equal?(x=w1335, y=refnum<class "Grapher.lvclass"> refnum) -> (x = y?=w1336:bool)
        n568 = case shown="False" w1336 {
          tunnel: w1340 -> [w1346 w1348]
          tunnel: [w1345 w1348] -> w1339
          tunnel: w1335 -> [w1344 w1347]
          tunnel: [refnum<class "Grapher.lvclass"> refnum ("y") w1347] -> w1334
          frame False {
            n569 = call-dynamic "Destroy.vi"("reference in"=w1344, "Error In"=w1346) -> ("Error Out"=w1345:errorcluster)  [unwired: 16 in, 1 out]
          }
          frame True {
          }
        }
        n570 = Bundle By Name(cluster=w1337, "Grapher Ref"=w1334) -> (w1338:T13)
      }
      frame "---------- Events ----------" {
        # "Do not put any code in this frame.\n(It is a separator no-op. You can make a copy of this frame to create a new UI frame)"
      }
      frame "Events: Register" {
        n571 = Unbundle By Name(w1356) -> ("EIS Profile Completed"=w1354:refnum<user-event>, "DCIR Profile Completed"=w1353:refnum<user-event>)
        n572 = register-events(error in=w1355, w1354, w1353) -> (reference out=w1358:refnum<event-registration>, error out=w1357:errorcluster)  [unwired: 1 in]
      }
      frame "Events: Unregister" {
        n573 = Unregister For Events(event registration refnum=w1362, error in=w1361) -> (error out=w1360:errorcluster)
      }
      frame "---------- UI ----------" {
        # "Do not put any code in this frame.\n(It is a separator no-op. You can make a copy of this frame to create a new UI frame)"
      }
      frame "UI: Initialize" {
        w1373 = T12 {"Numeric Indicator"=0.0, "Numeric Indicator"=0.0} ("CURRENT")
        w1371 = string[][] [] ("Item Names")
        w1375 = i16 -1 items=["NONE"=-1] ("Module Selection")
        w1380 = FALSE ("HPS Connect")
        w1370 = 0.0 ("POWER")
        w1372 = T14."Disabled and Grayed Out" ("Disabled")
        # "Initialize the User Interface, here.\n(this is called automatically, by the Macro: Initialize)"
        n574 = Format Into String(format string="%s: Initialize UI", w1376) -> (resulting string=w1378:string)  [unwired: 2 in, 1 out]
        n575 = call <userlib>:"Fit VI window to Largest Dec__ogtk.vi"("error in (no error)"=w1388) -> ("error out"=w1387:errorcluster)  [unwired: 5 in, 1 out]
        n576 = local write "Status Message"(w1378) -> ()
        n577 = property on="Enable Battery Simulation" class="Bool (strict)"("DisabledEnum"=w1372) -> ()  [unwired: 2 in, 2 out]
        n578 = property on="Apply Setpoints" class="Bool"("DisabledEnum"=w1372) -> ()  [unwired: 2 in, 2 out]
        n579 = property on="Energize" class="Bool (strict)"("DisabledEnum"=w1372) -> ()  [unwired: 2 in, 2 out]
        n580 = property on="Output" class="Bool (strict)"("DisabledEnum"=w1372) -> ()  [unwired: 2 in, 2 out]
        n581 = property on="PMOD Reserve" class="Bool (strict)"("DisabledEnum"=w1372) -> ()  [unwired: 2 in, 2 out]
        n582 = property on="Apply Mode & Range" class="Bool"("DisabledEnum"=w1372) -> ()  [unwired: 2 in, 2 out]
        n583 = property on="Apply Limits" class="Bool"("DisabledEnum"=w1372) -> ()  [unwired: 2 in, 2 out]
        n584 = property on="PMOD Clear" class="Bool"("DisabledEnum"=w1372) -> ()  [unwired: 2 in, 2 out]
        n585 = property on="Toggle EIS Profile" class="Bool (strict)"("DisabledEnum"=w1372) -> ()  [unwired: 2 in, 2 out]
        n586 = property on="Start Profile" class="Bool (strict)"("DisabledEnum"=w1372) -> ()  [unwired: 2 in, 2 out]
        n587 = property on="Power Module Plugins" class="MCListbox (strict)"("ItemNames"=w1371) -> ()  [unwired: 2 in, 2 out]
        n588 = property on="Events" class="MCListbox (strict)"("ItemNames"=w1371) -> ()  [unwired: 2 in, 2 out]
        n589 = property on="Apply Slew Rates" class="Bool"("DisabledEnum"=w1372) -> ()  [unwired: 2 in, 2 out]
        n590 = property on="Start Logging" class="Bool (strict)"("DisabledEnum"=w1372) -> ()  [unwired: 2 in, 2 out]
        n591 = property on="Launch Battery Simulation" class="Bool"("DisabledEnum"=w1372) -> ()  [unwired: 2 in, 2 out]
        n592 = property on="Reset Battery Simulation" class="Bool"("DisabledEnum"=w1372) -> ()  [unwired: 2 in, 2 out]
        n593 = property on="Generate EIS Profile" class="Bool"("DisabledEnum"=w1372) -> ()  [unwired: 2 in, 2 out]
        n594 = property on="Toggle HPPC Profile" class="Bool (strict)"("DisabledEnum"=w1372) -> ()  [unwired: 2 in, 2 out]
        n595 = property on="PMOD Connect" class="Bool (strict)"("DisabledEnum"=w1372) -> ()  [unwired: 2 in, 2 out]
        n596 = disable-structure shown="TARGET_TYPE==Windows, Default" {
          disable-tunnel: [w1392 path "/home/lvuser/natinst/bin" ("name or relative path")] -> w1379
          frame condition #0 (active) {
            n597 = property class="App"() -> ("App.Kind"=w1393:T16)  [unwired: 2 in, 2 out]
            n598 = case shown="\"Run Time System\"" w1393 {
              tunnel: [w1394 w1399] -> w1392
              frame "Development System", Default {
                n599 = Current VI's Path() -> (path=w1396:path)
                n600 = Build Path(base path=w1396, name or relative path=path "../../builds/Power Modules") -> (appended path=w1394:path)
              }
              frame "Run Time System" {
                n601 = call <vilib>:"Application Directory.vi"() -> ("Application Directory"=w1397:path)
                n602 = Build Path(base path=w1397, name or relative path="Power Modules") -> (appended path=w1399:path)
              }
            }
          }
          frame condition #1 {
          }
        }
        n603 = property on="Module Selection" class="Ring (strict)"("StringsAndValues[]"=T22 [{"String"="NONE", "Value"=-1}] ("Strings And Values []"), "Value"=w1375, "DisabledEnum"=T14."Enabled" ("Disabled")) -> ()  [unwired: 2 in, 2 out]
        n604 = local write "XY Graph"(T4 [] ("appended array")) -> ()
        n605 = property class="VI"("Front Panel.Title"="VOLTA CONTROL SUITE" ("Front Panel Window:Title")) -> ()  [unwired: 2 in, 2 out]
        n606 = local write "Main Tab Control"(Tabs."CONFIG" ("Main Tab Control")) -> ()
        n607 = local write "CURRENT"(w1373) -> ()
        n608 = local write "VOLTAGE"(w1373) -> ()
        n609 = local write "Charge Counter"(w1370) -> ()
        n610 = local write "POWER"(w1370) -> ()
        n611 = property on="EMO Indicator" class="Ring (strict)"("Value"=u16 0 ("EMO Indicator")) -> ()  [unwired: 2 in, 2 out]
        n612 = property on="Fault Message" class="Str"("Value"="" ("Error Message")) -> ()  [unwired: 2 in, 2 out]
        n613 = local write "Enable Battery Simulation"(w1380) -> ()
        n614 = local write "PMOD Connect"(w1380) -> ()
        n615 = local write "PMOD Reserve"(w1380) -> ()
        n616 = local write "Energize"(w1380) -> ()
        n617 = local write "Output"(w1380) -> ()
        n618 = local write "Start Profile"(w1380) -> ()
        n619 = local write "Module Plugin Directory"(w1379) -> ()
        n620 = local write "CSV Profile"(waveform(dbl)[] [] ("CSV Profile")) -> ()
      }
      frame "UI: Load Power Modules" {
        n621 = local read "Module Plugin Directory"() -> (w1412:path)
        n622 = Format Into String(format string="%s:  Loading Power Modules", w1407) -> (resulting string=w1409:string)  [unwired: 2 in, 1 out]
        n623 = local write "Status Message"(w1409) -> ()
        n624 = call "Load PPL Versions.vi"("error in"=w1413, "Module Plugin Directory"=w1412) -> ("error out"=w1405:errorcluster, "Plugin Objects"=w1401:refnum<class "PowerModuleInterface.lvclass">[], "Plugin Names"=w1411:string[], "Plugin Versions"=w1410:string[])  [unwired: 6 in]
        n625 = case shown="No Error" w1405 {
          selector: w1405 -> [w1424 w1448]
          tunnel: w1411 -> [w1431 _]
          tunnel: w1410 -> [w1430 _]
          tunnel: w1406 -> [w1425 _]
          tunnel: [w1419 w1448] -> w1404
          tunnel: w1403 -> [w1418 w1447]
          tunnel: [w1417 w1447] -> w1402
          tunnel: w1401 -> [w1416 _]
          frame No Error {
            n626 = property on="Module Selection" class="Ring (strict)"() -> ("StringsAndValues[]"=w1421:T22)  [unwired: 2 in, 2 out]
            n627 = Build Array(w1431, w1430) -> (w1429:string[][])
            n628 = Transpose 2D Array(2D array=w1429) -> (transposed array=w1422:string[][])
            n629 = for {
              tunnel: w1422 -> [w1438] mode=indexing
              shift-right: [w1439] -> w1420
              shift-left: w1421 -> [w1440]
              i -> [w1434]
              n630 = Index Array(array=w1438) -> (element=w1437:string)  [unwired: 1 in]
              n631 = Search/Split String(string=w1437, search string/char (-)="-PowerModule") -> (substring before match=w1432:string)  [unwired: 1 in, 2 out]
              n632 = Bundle By Name(cluster=cluster{"String":string, "Value":i16} {"String"="", "Value"=0} ("new element/subarray"), "Value"=w1434, "String"=w1432) -> (w1433:cluster{"String":string, "Value":i16})
              n633 = Insert Into Array(array=w1440, new element=w1433) -> (w1439:T22)  [unwired: 1 in]
            }
            n634 = property on="Power Module Plugins" class="MCListbox (strict)"(error in=w1424, "ItemNames"=w1422) -> (error out=w1419:errorcluster)  [unwired: 1 in, 1 out]
            n635 = flat-sequence {
              tunnel: [w1446] -> w1426
              tunnel: w1425 -> [w1444]
              tunnel: [w1441] -> w1423
              tunnel: w1419 -> [_]
              frame #0 {
                n636 = call "Get Timestamp String.vi"() -> ("date/time string"=w1446:string)  [unwired: 11 in]
                n637 = Tick Count (ms)() -> (millisecond timer value=w1445:u32)
                n638 = Subtract(x=w1445, y=w1444) -> (x-y=w1443:u32)
                n639 = Quotient & Remainder(x=w1443, y=u32 1000) -> (floor(x/y)=w1441:u32)  [unwired: 1 out]
              }
            }
            n640 = property on="Module Selection" class="Ring (strict)"("StringsAndValues[]"=w1420) -> ()  [unwired: 2 in, 2 out]
            n641 = Format Into String(format string="%s:  Loaded Power Modules in %d seconds", w1426, w1423) -> (resulting string=w1427:string)  [unwired: 2 in, 1 out]
            n642 = Bundle By Name(cluster=w1418, "Plugin Objects"=w1416) -> (w1417:T13)
            n643 = local write "Status Message"(w1427) -> ()
          }
          frame Error {
            n644 = Unbundle By Name(w1448) -> ("code"=w1449:i32)
            n645 = call "Get Timestamp String.vi"() -> ("date/time string"=w1450:string)  [unwired: 11 in]
            n646 = Format Into String(format string="%s: Error %d occured when loading power modules", w1450, w1449) -> (resulting string=w1452:string)  [unwired: 2 in, 1 out]
            n647 = local write "Status Message"(w1452) -> ()
          }
        }
      }
      frame "UI: Uninitialize" {
        # "Cleanup the User Interface, here.\n(this is called automatically, by the Macro: Exit)"
      }
      frame "UI: Self Test Start" {
        w1457 = T14."Disabled and Grayed Out" ("Disabled")
        n648 = property on="Apply Mode & Range" class="Bool"("DisabledEnum"=w1457) -> ()  [unwired: 2 in, 2 out]
        n649 = property on="Apply Limits" class="Bool"("DisabledEnum"=w1457) -> ()  [unwired: 2 in, 2 out]
        n650 = property on="Apply Setpoints" class="Bool"("DisabledEnum"=w1457) -> ()  [unwired: 2 in, 2 out]
        n651 = property on="Apply Slew Rates" class="Bool"("DisabledEnum"=w1457) -> ()  [unwired: 2 in, 2 out]
        n652 = property on="Energize" class="Bool (strict)"("DisabledEnum"=w1457) -> ()  [unwired: 2 in, 2 out]
        n653 = property on="Output" class="Bool (strict)"("DisabledEnum"=w1457) -> ()  [unwired: 2 in, 2 out]
      }
      frame "UI: Self Test Stop" {
        w1463 = T14."Enabled" ("Disabled")
        n654 = property on="Apply Mode & Range" class="Bool"("DisabledEnum"=w1463) -> ()  [unwired: 2 in, 2 out]
        n655 = property on="Apply Limits" class="Bool"("DisabledEnum"=w1463) -> ()  [unwired: 2 in, 2 out]
        n656 = property on="Apply Setpoints" class="Bool"("DisabledEnum"=w1463) -> ()  [unwired: 2 in, 2 out]
        n657 = property on="Apply Slew Rates" class="Bool"("DisabledEnum"=w1463) -> ()  [unwired: 2 in, 2 out]
        n658 = property on="Energize" class="Bool (strict)"("DisabledEnum"=w1463) -> ()  [unwired: 2 in, 2 out]
        n659 = property on="Output" class="Bool (strict)"("DisabledEnum"=w1463) -> ()  [unwired: 2 in, 2 out]
      }
      frame "UI: Start Profile" {
        w1470 = T14."Disabled and Grayed Out" ("Disabled")
        n660 = Format Into String(format string="%s:  Profile Started", w1467) -> (resulting string=w1469:string)  [unwired: 2 in, 1 out]
        n661 = local write "Status Message"(w1469) -> ()
        n662 = property on="Start Profile" class="Bool (strict)"("DisabledEnum"=w1470) -> ()  [unwired: 2 in, 2 out]
        n663 = property on="Apply Slew Rates" class="Bool"("DisabledEnum"=w1470) -> ()  [unwired: 2 in, 2 out]
        n664 = property on="Energize" class="Bool (strict)"("DisabledEnum"=w1470) -> ()  [unwired: 2 in, 2 out]
        n665 = property on="Output" class="Bool (strict)"("DisabledEnum"=w1470) -> ()  [unwired: 2 in, 2 out]
        n666 = property on="Apply Setpoints" class="Bool"("DisabledEnum"=w1470) -> ()  [unwired: 2 in, 2 out]
        n667 = property on="Apply Mode & Range" class="Bool"("DisabledEnum"=w1470) -> ()  [unwired: 2 in, 2 out]
        n668 = property on="Apply Limits" class="Bool"("DisabledEnum"=w1470) -> ()  [unwired: 2 in, 2 out]
        n669 = property on="Start Logging" class="Bool (strict)"("DisabledEnum"=w1470) -> ()  [unwired: 2 in, 2 out]
      }
      frame "UI: Stop Profile" {
        w1478 = T14."Enabled" ("Disabled")
        n670 = Format Into String(format string="%s:  Profile Stopped", w1475) -> (resulting string=w1477:string)  [unwired: 2 in, 1 out]
        n671 = local write "Status Message"(w1477) -> ()
        n672 = property on="Start Profile" class="Bool (strict)"("DisabledEnum"=w1478) -> ()  [unwired: 2 in, 2 out]
        n673 = property on="Apply Slew Rates" class="Bool"("DisabledEnum"=w1478) -> ()  [unwired: 2 in, 2 out]
        n674 = property on="Energize" class="Bool (strict)"("DisabledEnum"=w1478) -> ()  [unwired: 2 in, 2 out]
        n675 = property on="Output" class="Bool (strict)"("DisabledEnum"=w1478) -> ()  [unwired: 2 in, 2 out]
        n676 = property on="Apply Setpoints" class="Bool"("DisabledEnum"=w1478) -> ()  [unwired: 2 in, 2 out]
        n677 = property on="Apply Mode & Range" class="Bool"("DisabledEnum"=w1478) -> ()  [unwired: 2 in, 2 out]
        n678 = property on="Apply Limits" class="Bool"("DisabledEnum"=w1478) -> ()  [unwired: 2 in, 2 out]
        n679 = property on="Start Logging" class="Bool (strict)"("DisabledEnum"=w1478) -> ()  [unwired: 2 in, 2 out]
      }
      frame "UI: Reservation Complete" {
        n680 = Format Into String(format string="%s: Reservation Successful", w1483) -> (resulting string=w1485:string)  [unwired: 2 in, 1 out]
        n681 = local write "Status Message"(w1485) -> ()
      }
      frame "UI: Reservation Failed" {
        n682 = Format Into String(format string="%s: Reservation Failed", w1490) -> (resulting string=w1492:string)  [unwired: 2 in, 1 out]
        n683 = local write "Status Message"(w1492) -> ()
      }
      frame "UI: Connection Complete" {
        n684 = Format Into String(format string="%s: Connection Successful", w1497) -> (resulting string=w1499:string)  [unwired: 2 in, 1 out]
        n685 = local write "Status Message"(w1499) -> ()
      }
      frame "UI: Connection Failed" {
        n686 = Format Into String(format string="%s: Connection Failed", w1504) -> (resulting string=w1506:string)  [unwired: 2 in, 1 out]
        n687 = local write "Status Message"(w1506) -> ()
      }
      frame "UI: Cursor Set" {
        # "Argument"
        # "Set and Unset Cursor Busy.\n(Usage: \"UI: Cursor Set >> Busy|Idle\")"
        n688 = disable-structure shown="TARGET_TYPE==RT" {
          disable-tunnel: w1514 -> [w1519 w1524]
          disable-tunnel: [w1518 w1524] -> w1513
          disable-tunnel: w1512 -> [w1517 _]
          frame condition #0 (active) {
            n689 = case shown="\"Idle\", Default" w1517 {
              tunnel: w1519 -> [w1521 w1523]
              tunnel: [w1520 w1522] -> w1518
              frame "Idle", Default {
                n690 = call <vilib>:"Unset Busy.vi"("error in (no error)"=w1521) -> ("error out"=w1520:errorcluster)  [unwired: 10 in]
              }
              frame "Busy" {
                n691 = call <vilib>:"Set Busy.vi"("error in (no error)"=w1523) -> ("error out"=w1522:errorcluster)  [unwired: 9 in, 1 out]
              }
            }
          }
          frame condition #1 {
          }
        }
      }
      frame "UI: Front Panel State" {
        # "Argument"
        # "Set Front Panel Open or Closed\n(Usage: \"UI: Front Panel State >> Open|Close\")"
        n692 = Unbundle By Name(w1528) -> ("Core.Current VI Reference"=w1527:refnum<vi>)
        n693 = case shown="\"Open\", \"Standard\", Default" w1526 {
          tunnel: w1530 -> [w1537 w1552 w1563 w1576 w1589]
          tunnel: [w1539 w1553 w1565 w1578 w1591] -> w1529
          tunnel: w1527 -> [w1538 w1550 w1564 w1577 w1590]
          frame "Open", "Standard", Default {
            w1532 = T15."Standard" ("State")
            n694 = property class="VI"(reference=w1538, error in=w1537) -> (reference out=w1535:refnum<vi>, error out=w1536:errorcluster, "FP.State"=w1534:T15)
            n695 = Not Equal?(x=w1534, y=w1532) -> (x != y?=w1533:bool)
            n696 = case shown="True" w1533 {
              tunnel: [w1543 w1545] -> w1539
              tunnel: w1536 -> [w1542 w1545]
              tunnel: w1535 -> [w1541 _]
              tunnel: w1532 -> [w1540 _]
              frame True {
                n697 = invoke class="VI" method="FP.Open"(reference=w1541, error in=w1542, "Activate"=TRUE, "State"=w1540) -> (error out=w1543:errorcluster)  [unwired: 1 in, 4 out]
              }
              frame False {
              }
            }
          }
          frame "Close", "Closed" {
            n698 = property class="VI"(reference=w1550, error in=w1552) -> (reference out=w1549:refnum<vi>, error out=w1551:errorcluster, "FP.State"=w1547:T15)
            n699 = Not Equal?(x=w1547, y=T15."Closed" ("Front Panel Window:State")) -> (x != y?=w1546:bool)
            n700 = case shown="True" w1546 {
              tunnel: [w1554 w1557] -> w1553
              tunnel: w1551 -> [w1554 w1556]
              tunnel: w1549 -> [_ w1555]
              frame False {
              }
              frame True {
                n701 = invoke class="VI" method="FP.Close"(reference=w1555, error in=w1556) -> (error out=w1557:errorcluster)  [unwired: 1 in, 2 out]
              }
            }
          }
          frame "Hidden", "Hide" {
            w1558 = T15."Hidden" ("State")
            n702 = property class="VI"(reference=w1564, error in=w1563) -> (reference out=w1561:refnum<vi>, error out=w1562:errorcluster, "FP.State"=w1560:T15)
            n703 = Not Equal?(x=w1560, y=w1558) -> (x != y?=w1559:bool)
            n704 = case shown="True" w1559 {
              tunnel: [w1569 w1570] -> w1565
              tunnel: w1562 -> [w1568 w1570]
              tunnel: w1561 -> [w1567 _]
              tunnel: w1558 -> [w1566 _]
              frame True {
                n705 = invoke class="VI" method="FP.Open"(reference=w1567, error in=w1568, "State"=w1566) -> (error out=w1569:errorcluster)  [unwired: 2 in, 4 out]
              }
              frame False {
              }
            }
          }
          frame "Minimize", "Minimized" {
            w1571 = T15."Minimized" ("State")
            n706 = property class="VI"(reference=w1577, error in=w1576) -> (reference out=w1574:refnum<vi>, error out=w1575:errorcluster, "FP.State"=w1573:T15)
            n707 = Not Equal?(x=w1573, y=w1571) -> (x != y?=w1572:bool)
            n708 = case shown="True" w1572 {
              tunnel: [w1582 w1583] -> w1578
              tunnel: w1575 -> [w1581 w1583]
              tunnel: w1574 -> [w1580 _]
              tunnel: w1571 -> [w1579 _]
              frame True {
                n709 = invoke class="VI" method="FP.Open"(reference=w1580, error in=w1581, "State"=w1579) -> (error out=w1582:errorcluster)  [unwired: 2 in, 4 out]
              }
              frame False {
              }
            }
          }
          frame "Maximize", "Maximized" {
            w1584 = T15."Maximized" ("State")
            n710 = property class="VI"(reference=w1590, error in=w1589) -> (reference out=w1587:refnum<vi>, error out=w1588:errorcluster, "FP.State"=w1586:T15)
            n711 = Not Equal?(x=w1586, y=w1584) -> (x != y?=w1585:bool)
            n712 = case shown="True" w1585 {
              tunnel: [w1595 w1596] -> w1591
              tunnel: w1588 -> [w1594 w1596]
              tunnel: w1587 -> [w1593 _]
              tunnel: w1584 -> [w1592 _]
              frame True {
                n713 = invoke class="VI" method="FP.Open"(reference=w1593, error in=w1594, "State"=w1592) -> (error out=w1595:errorcluster)  [unwired: 2 in, 4 out]
              }
              frame False {
              }
            }
          }
        }
      }
      frame "---------- Macro ----------" {
        # "Do not put any code in this frame.\n(It is a separator no-op. You can make a copy of this frame to create a new Macro frame)"
      }
      frame "Macro: Initialize" {
        # "Initialization Macro\n(This is called once, when the VI starts)"
        n714 = call <vilib>:"Add State(s) to Queue__jki_lib_state_machine.vi"("State(s) in Front (\"\")"="UI: Cursor Set >> Busy\nData: Initialize\nInitialize Core Data\nUI: Initialize\nUI: Front Panel State >> Open\nUI: Load Power Modules\nUI: Cursor Set >> Idle", "State(s) in (\"\")"=w1606) -> ("States Out"=w1605:string)  [unwired: 13 in]
      }
      frame "Macro: Unreserve" {
        w1607 = FALSE ("Energize")
        # "Unreserve Macro\n(This is called when we unreserve the Power Module)"
        n715 = local write "Energize"(w1607) -> ()
        n716 = local write "Output"(w1607) -> ()
        n717 = call <vilib>:"Add State(s) to Queue__jki_lib_state_machine.vi"("State(s) in Front (\"\")"="UI: Cursor Set >> Busy\nPMOD: Output\nPMOD: Energize\nPMOD: Unreserve\nScript: Stop Battery\nUI: Cursor Set >> Idle", "State(s) in (\"\")"=w1613) -> ("States Out"=w1612:string)  [unwired: 13 in]
      }
      frame "Macro: Reserve" {
        # "Reserve Macro\n(This is called when we reserve the Power Module)"
        n718 = call <vilib>:"Add State(s) to Queue__jki_lib_state_machine.vi"("State(s) in Front (\"\")"="UI: Cursor Set >> Busy\nPMOD: Reserve\nPMOD: Get Limits\nPMOD: Read Slew Rates\nData: Update Periodic\nUI: Reservation Complete\nUI: Cursor Set >> Idle", "State(s) in (\"\")"=w1619) -> ("States Out"=w1618:string)  [unwired: 13 in]
      }
      frame "Macro: Connect" {
        # "Connect Macro\n(This is called when we connect to the HPS17K)"
        n719 = call <vilib>:"Add State(s) to Queue__jki_lib_state_machine.vi"("State(s) in Front (\"\")"="UI: Cursor Set >> Busy\nPMOD: Connect\nPMOD: Get Mode and Range\nScript: Launch Grapher\nScript: Launch Logger\nEvents: Register\nUI: Connection Complete\nUI: Cursor Set >> Idle", "State(s) in (\"\")"=w1625) -> ("States Out"=w1624:string)  [unwired: 13 in]
      }
      frame "Macro: Disconnect" {
        # "Disconnect Macro\n(This is called when we disconnect from the Power Module)"
        n720 = Unbundle By Name(w1633) -> ("Reserved"=w1632:bool, "Connected"=w1628:bool)
        n721 = Select(t="UI: Cursor Set >> Busy\nMacro: Unreserve\nScript: Stop Grapher\nScript: Destroy Logger\nPMOD: Disconnect\nUI: Cursor Set >> Idle", s=w1632, f="UI: Cursor Set >> Busy\nScript: Stop Grapher\nScript: Destroy Logger\nPMOD: Disconnect\nUI: Cursor Set >> Idle") -> (s? t:f=w1629:string)
        n722 = Select(t=w1629, s=w1628, f="") -> (s? t:f=w1626:string)
        n723 = call <vilib>:"Add State(s) to Queue__jki_lib_state_machine.vi"("State(s) in Front (\"\")"=w1626, "State(s) in (\"\")"=w1637) -> ("States Out"=w1636:string)  [unwired: 13 in]
      }
      frame "Macro: Exit" {
        # "Exit Macro\n(This is called once, when the VI exits)"
        n724 = Unbundle By Name(w1646) -> ("Core.Close Panel on Exit?"=w1642:bool)
        n725 = call <vilib>:"Conditional State String__jki_lib_state_machine.vi"("Do State(s)?"=w1642, "State"="UI: Front Panel State >> Close") -> ("State Out"=w1641:string)  [unwired: 7 in]
        n726 = call <vilib>:"Add State(s) to Queue__jki_lib_state_machine.vi"("State(s) in Front (\"\")"="Script: Stop Battery\nScript: Stop Logger\nUI: Uninitialize\nData: Cleanup\nMacro: Disconnect", "State(s) in (\"\")"=w1641, "State(s) at Back (\"\")"="Exit") -> ("States Out"=w1639:string)  [unwired: 12 in]
      }
    }
  }
